vi "VIP_Phase_5.vi"() -> ()   [LabVIEW 2024]
uses:
  <vilib>/DAQmx/read.llb/DAQmx Read (Digital 1D Bool 1Chan 1Samp).vi
  <vilib>/Utility/file.llb/Write To Spreadsheet File (DBL).vi
  <vilib>/DAQmx/create/channels.llb/DAQmx Create Channel (DI-Digital Input).vi
  <vilib>/DAQmx/miscellaneous.llb/DAQmx Fill In Error Info.vi
  <vilib>/ptbypt/NI_PtbyPt.lvlib
panel:
  out "fault 4":dbl
  out "fault 3":dbl
  out "fault 2":dbl
  out "fault 1":dbl
  in  "LED 4":tag="Dev1/port0/line23"
  in  "LED 3":tag="Dev1/port0/line22"
  in  "LED 2":tag="Dev1/port0/line21"
  out "LED 4 (i)":dbl
  out "LED 3 (i)":dbl
  out "LED 2 (i)":dbl
  in  "LED 1":tag="Dev1/port0/line20"
  out "LED 1(i)":dbl
  out "4.2":bool
  out "mouse 4.2":cluster{"Y":dbl[], "Y":dbl[]}[](graph)
  out "mouse 4.1":cluster{"Y":dbl[], "Y":dbl[]}[](graph)
  in  "fake 4.2":bool
  in  "fake 4.1":bool
  out "ratio 4.2R":cluster{"Y":dbl[], "Y":dbl[]}[](graph)=[{"Y"=[2.5380001068115234, 12.063000202178955, 24.592000007629395, 36.145999908447266, 48.69600009918213, 58.23899984359741, 67.79099988937378, 81.40899991989136, 91.96199989318848, 99.9980001449585], "Y"=[0.0, 0.0, 0.0, 0.0, 0.0, 0.0, 0.0, 0.0, 0.0, 0.0]}]
  out "ratio 4.1L":cluster{"Y":dbl[], "Y":dbl[]}[](graph)=[{"Y"=[2.5380001068115234, 12.063000202178955, 24.592000007629395, 36.145999908447266, 48.69600009918213, 58.23899984359741, 67.79099988937378, 81.40899991989136, 91.96199989318848, 99.9980001449585], "Y"=[0.0, 0.0, 0.0, 0.0, 0.0, 0.0, 0.0, 0.0, 0.0, 0.0]}]
  out "ratio 4.2R":dbl
  out "ratio 4.1L":dbl
  in  "water dur (ms) 4.2":dbl=11.5
  in  "water port 4.2":tag="Dev1/port2/line0"
  out "Mouse path 4":path=path "C:/Users/Administrator/Documents/LabVIEW Data/a-lick-20140707-145848"
  out "Mouse file 4":string="a-lick-20140707-145848"
  in  "Mouse ID 4":string="test_4"
  in  "water dur (ms) 4.1":dbl=8.5
  in  "water port 4.1":tag="Dev1/port1/line7"
  in  "free water 4.2":bool
  in  "free water 4.1":bool
  out "4.1":bool
  out "state 4.2":enum16{"waiting", "sound", "ITI"}(ring)=enum."ITI"
  out "state 4.1":enum16{"waiting", "sound", "ITI"}(ring)=enum."ITI"
  out "water # 4.1L":dbl
  out "water # 4.2R":dbl
  out "lick # 4.2R":dbl
  out "lick # 4.1L":dbl
  out "last water 4.2R":dbl
  out "last water 4.1L":dbl
  out "mistake # 4.2R":dbl
  out "mistake # 4.1L":dbl
  out "ratio 3.2R":cluster{"Y":dbl[], "Y":dbl[]}[](graph)=[{"Y"=[2.5380001068115234, 12.063000202178955, 24.592000007629395, 36.145999908447266, 48.69600009918213, 58.23899984359741, 67.79099988937378, 81.40899991989136, 91.96199989318848, 99.9980001449585], "Y"=[0.0, 0.0, 0.0, 0.0, 0.0, 0.0, 0.0, 0.0, 0.0, 0.0]}]
  out "ratio 3.1L":cluster{"Y":dbl[], "Y":dbl[]}[](graph)=[{"Y"=[2.5380001068115234, 12.063000202178955, 24.592000007629395, 36.145999908447266, 48.69600009918213, 58.23899984359741, 67.79099988937378, 81.40899991989136, 91.96199989318848, 99.9980001449585], "Y"=[0.0, 0.0, 0.0, 0.0, 0.0, 0.0, 0.0, 0.0, 0.0, 0.0]}]
  in  "free water 3.2":bool
  in  "free water 3.1":bool
  in  "water dur (ms) 3. 2":dbl=25.0
  in  "water dur (ms) 3.1":dbl=25.0
  out "mouse 3.2":cluster{"Y":dbl[], "Y":dbl[]}[](graph)
  out "mouse 3.1":cluster{"Y":dbl[], "Y":dbl[]}[](graph)
  in  "fake 3.2":bool
  in  "fake 3.1":bool
  out "last water 3.2R":dbl
  out "last water 3.1L":dbl
  out "mistake # 3.2R":dbl
  out "mistake # 3.1L":dbl
  out "water # 3.2R":dbl
  out "water # 3.1L":dbl
  out "lick # 3.2R":dbl
  out "lick # 3.1L":dbl
  out "ratio 3.2R":dbl
  out "ratio 3.1L":dbl
  in  "water port 3.2":tag="Dev1/port1/line6"
  out "3.2":bool
  out "state 3.2":enum16{"waiting", "sound", "ITI"}(ring)=enum."ITI"
  out "state 3.1":enum16{"waiting", "sound", "ITI"}(ring)=enum."ITI"
  out "3.1":bool
  out "Mouse path 3":path=path "C:/Users/Administrator/Documents/LabVIEW Data/a-lick-20140707-145848"
  out "Mouse file 3":string="a-lick-20140707-145848"
  in  "water port 3.1":tag="Dev1/port1/line5"
  in  "Mouse ID 3":string="test_3"
  out "ratio 2.2R":cluster{"Y":dbl[], "Y":dbl[]}[](graph)=[{"Y"=[2.5380001068115234, 12.063000202178955, 24.592000007629395, 36.145999908447266, 48.69600009918213, 58.23899984359741, 67.79099988937378, 81.40899991989136, 91.96199989318848, 99.9980001449585], "Y"=[0.0, 0.0, 0.0, 0.0, 0.0, 0.0, 0.0, 0.0, 0.0, 0.0]}]
  out "ratio 2.1L":cluster{"Y":dbl[], "Y":dbl[]}[](graph)=[{"Y"=[2.5380001068115234, 12.063000202178955, 24.592000007629395, 36.145999908447266, 48.69600009918213, 58.23899984359741, 67.79099988937378, 81.40899991989136, 91.96199989318848, 99.9980001449585], "Y"=[0.0, 0.0, 0.0, 0.0, 0.0, 0.0, 0.0, 0.0, 0.0, 0.0]}]
  out "ratio 1.2R":cluster{"Y":dbl[], "Y":dbl[]}[](graph)=[{"Y"=[2.5380001068115234, 12.063000202178955, 24.592000007629395, 36.145999908447266, 48.69600009918213, 58.23899984359741, 67.79099988937378, 81.40899991989136, 91.96199989318848, 99.9980001449585], "Y"=[0.0, 0.0, 0.0, 0.0, 0.0, 0.0, 0.0, 0.0, 0.0, 0.0]}]
  out "mouse 2.2":cluster{"Y":dbl[], "Y":dbl[]}[](graph)
  out "mouse 2.1":cluster{"Y":dbl[], "Y":dbl[]}[](graph)
  in  "free water 2.2":bool
  in  "free water 2.1":bool
  out "last water 2.2R":dbl
  out "last water 2.1L":dbl
  out "mistake # 2.2R":dbl
  out "mistake # 2.1L":dbl
  out "water # 2.2R":dbl
  out "water # 2.1L":dbl
  out "lick  #  2.2R":dbl
  out "lick  #  2.1L":dbl
  out "2.1":bool
  out "ratio 2.2R":dbl
  out "ratio 2.1L":dbl
  out "2.2":bool
  in  "fake 2.2":bool
  in  "fake 2.1":bool
  out "Mouse path 2":path=path "C:/Users/Administrator/Documents/LabVIEW Data/a-lick-20140707-145848"
  out "Mouse file 2":string="a-lick-20140707-145848"
  in  "Mouse ID 2":string="test_2"
  in  "water dur (ms) 2.2":dbl=25.5
  in  "water dur (ms) 2.1":dbl=34.5
  in  "water port 2.2":tag="Dev1/port1/line4"
  in  "water port 2.1":tag="Dev1/port1/line3"
  out "state 2.2":enum16{"waiting", "sound", "ITI"}(ring)=enum."ITI"
  out "state 2.1":enum16{"waiting", "sound", "ITI"}(ring)=enum."ITI"
  in  "sound port 2":tag="Dev1/ao1"
  out "time (s)":dbl=103.38100004196167
  out "mistake # 1.2R":dbl
  out "mistake # 1.1L":dbl
  in  "water dur (ms) 1.1":dbl=31.0
  in  "water port 1.1":tag="Dev1/port1/line1"
  in  "water dur (ms) 1.2":dbl=25.0
  in  "water port 1.2":tag="Dev1/port1/line2"
  out "1.1":bool
  out "1.2":bool
  out "state 1.2":enum16{"waiting", "sound", "ITI"}(ring)=enum."ITI"
  out "lick # 1.2R":dbl
  out "water # 1.2R":dbl
  in  "fake 1.2":bool
  in  "free water 1.2":bool
  out "mouse 1.2":cluster{"Y":dbl[], "Y":dbl[]}[](graph)
  out "ratio 1.2R":dbl
  out "last water 1.2R":dbl
  out "ratio 1.1L":dbl
  out "ratio 1.1L":cluster{"Y":dbl[], "Y":dbl[]}[](graph)=[{"Y"=[2.5380001068115234, 12.063000202178955, 24.592000007629395, 36.145999908447266, 48.69600009918213, 58.23899984359741, 67.79099988937378, 81.40899991989136, 91.96199989318848, 99.9980001449585], "Y"=[0.0, 0.0, 0.0, 0.0, 0.0, 0.0, 0.0, 0.0, 0.0, 0.0]}]
  in  "free water 1.1":bool
  out "Right Speaker":dbl=5.0
  out "Left Speaker":dbl=5.0
  in  "sound file 2":path=path "C:/Users/cvm-gritton-lab/Documents/Lab View Programs/Lab View Programs/LabVIEW VIs/Tones/New_Phase_2_Sounds/200k_target2.wav"
  in  "ITI max (ms)":dbl=7000.0
  in  "ITI min (ms)":dbl=5000.0
  in  "reaction dur (ms)":dbl=1750.0
  in  "sound dur (ms)":dbl=3000.0
  in  "sound file 1":path=path "C:/Users/cvm-gritton-lab/Documents/Lab View Programs/Lab View Programs/LabVIEW VIs/Tones/New_Phase_2_Sounds/200k_target1.wav"
  in  "sound port 1":tag="Dev1/ao0"
  out "trial state":T1(ring)=enum."ITI"
  out "trial #":dbl=10.0
  out "current sound":dbl=1.0
  out "next sound":dbl[](array[numeric])
  out "Mouse path 1":path=path "C:/Users/Administrator/Documents/LabVIEW Data/a-lick-20140707-145848"
  in  "fake 1.1":bool
  out "mouse 1.1":cluster{"Y":dbl[], "Y":dbl[]}[](graph)
  out "ITI (s)":dbl=6.5
  out "last water 1.1L":dbl
  out "state 1.1":enum16{"waiting", "sound", "ITI"}(ring)=enum."ITI"
  out "water # 1.1L":dbl
  out "lick # 1.1L":dbl
  out "Mouse file 1":string="a-lick-20140707-145848"
  out "data folder":path=path "C:/LabVIEW VIs/LabVIEW data"
  in  "Mouse ID 1":string="test_1"
  in  "lick port":tag="Dev1/port0/line0:7"
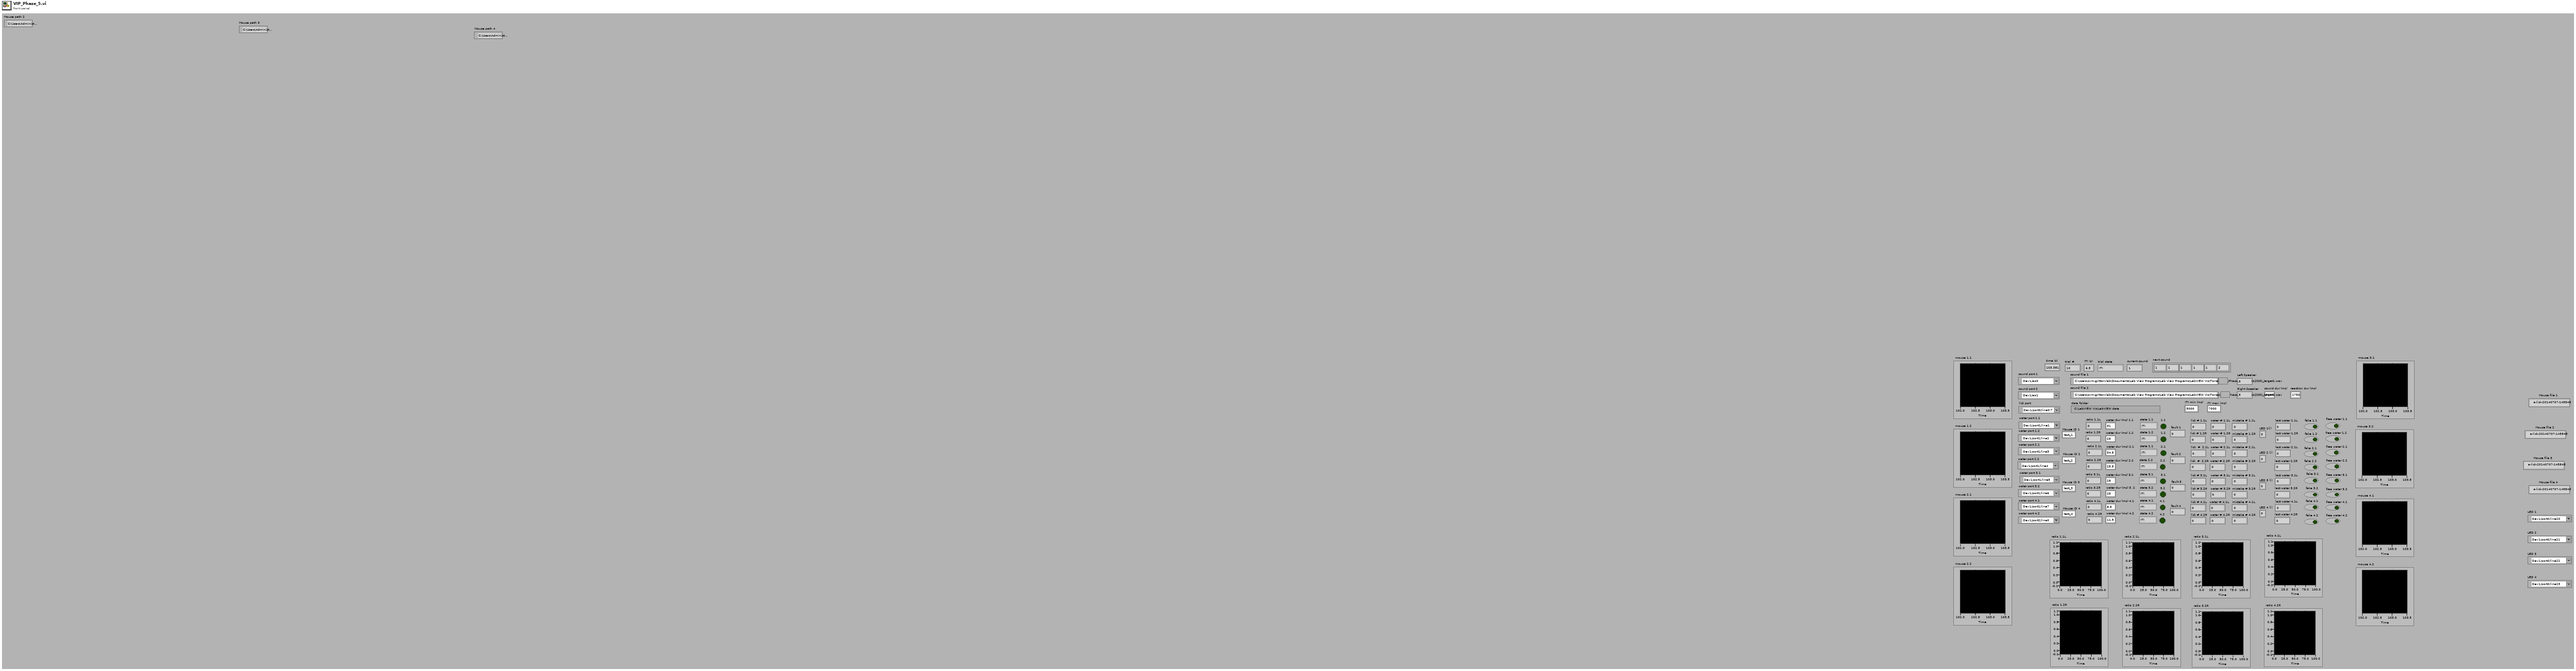
[diagram p1: front panel]
types:
  T1 = enum16{"prepare", "sound", "reaction window", "ITI", "free water", "graph", "data collection"}
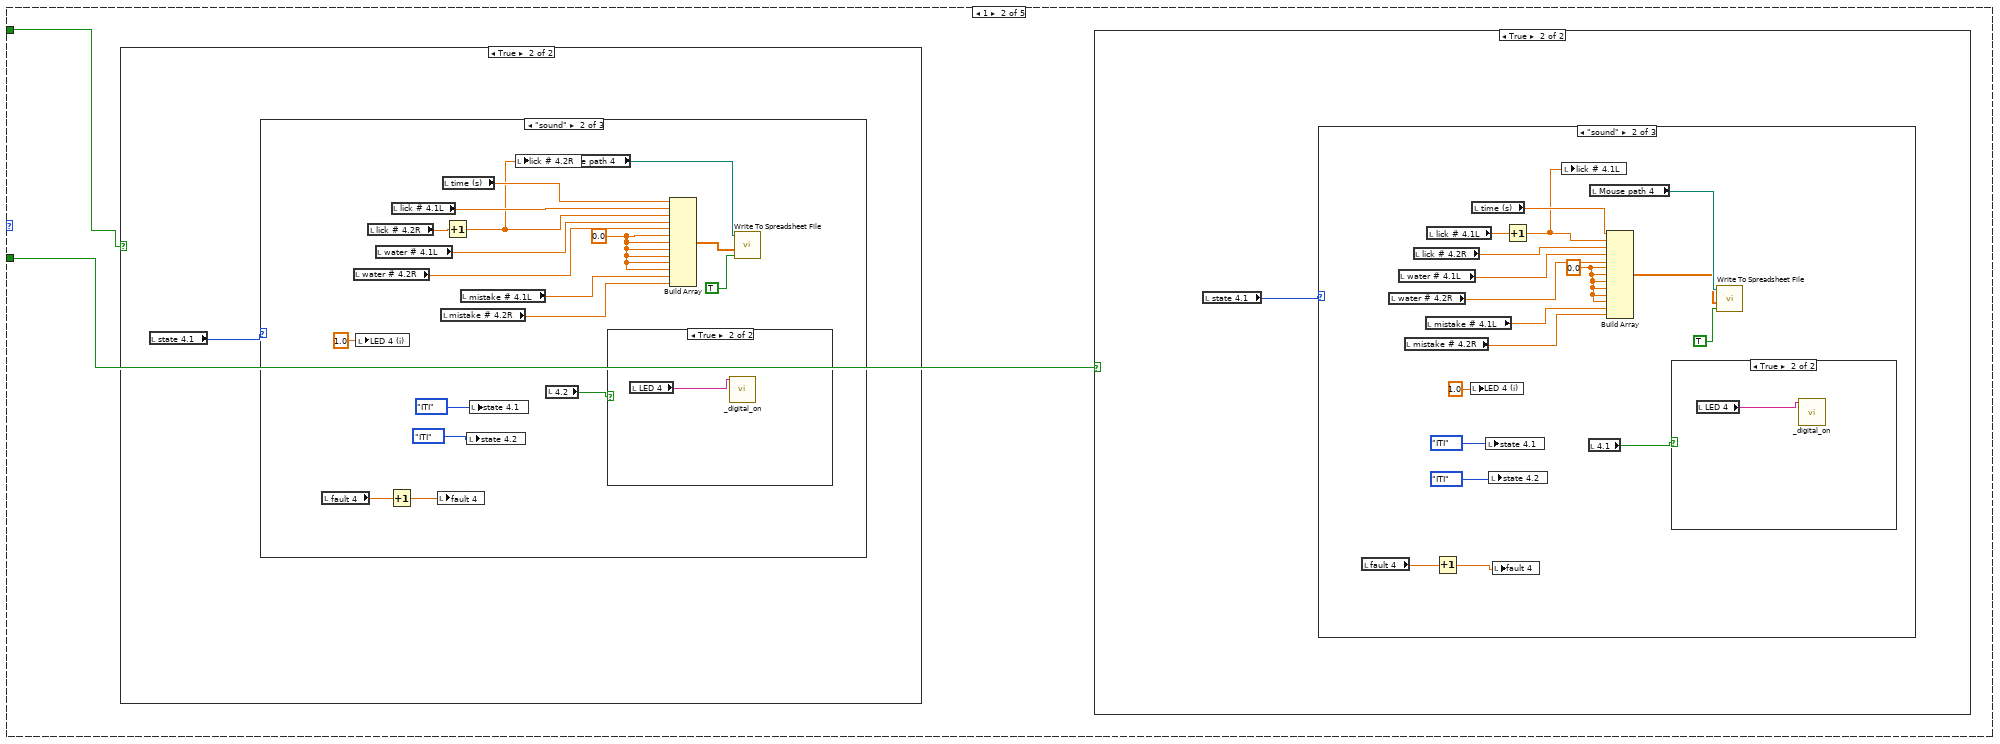
[diagram p3: hidden frame]
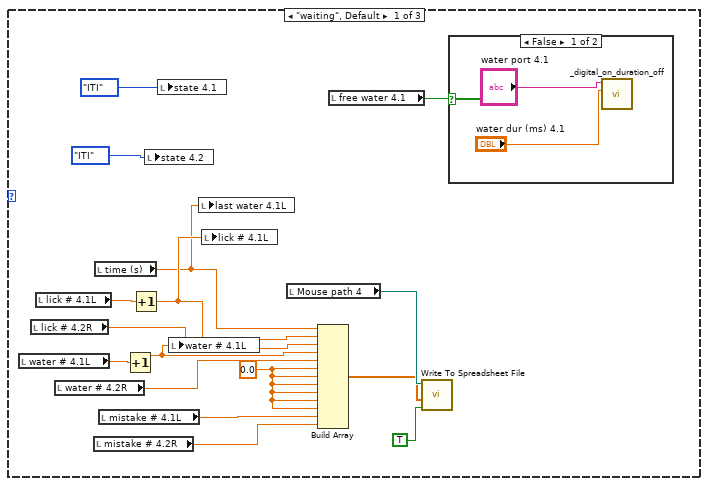
[diagram p5: hidden frame]
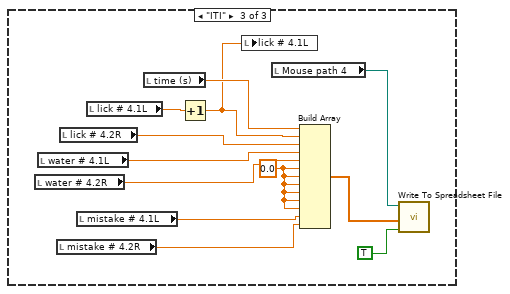
[diagram p8: hidden frame]
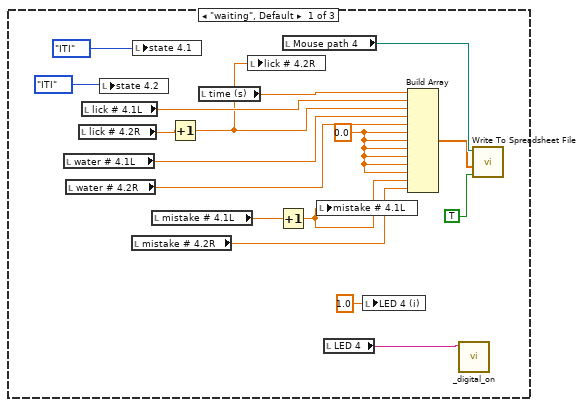
[diagram p10: hidden frame]
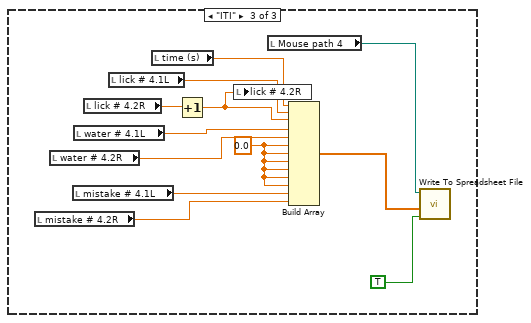
[diagram p12: hidden frame]
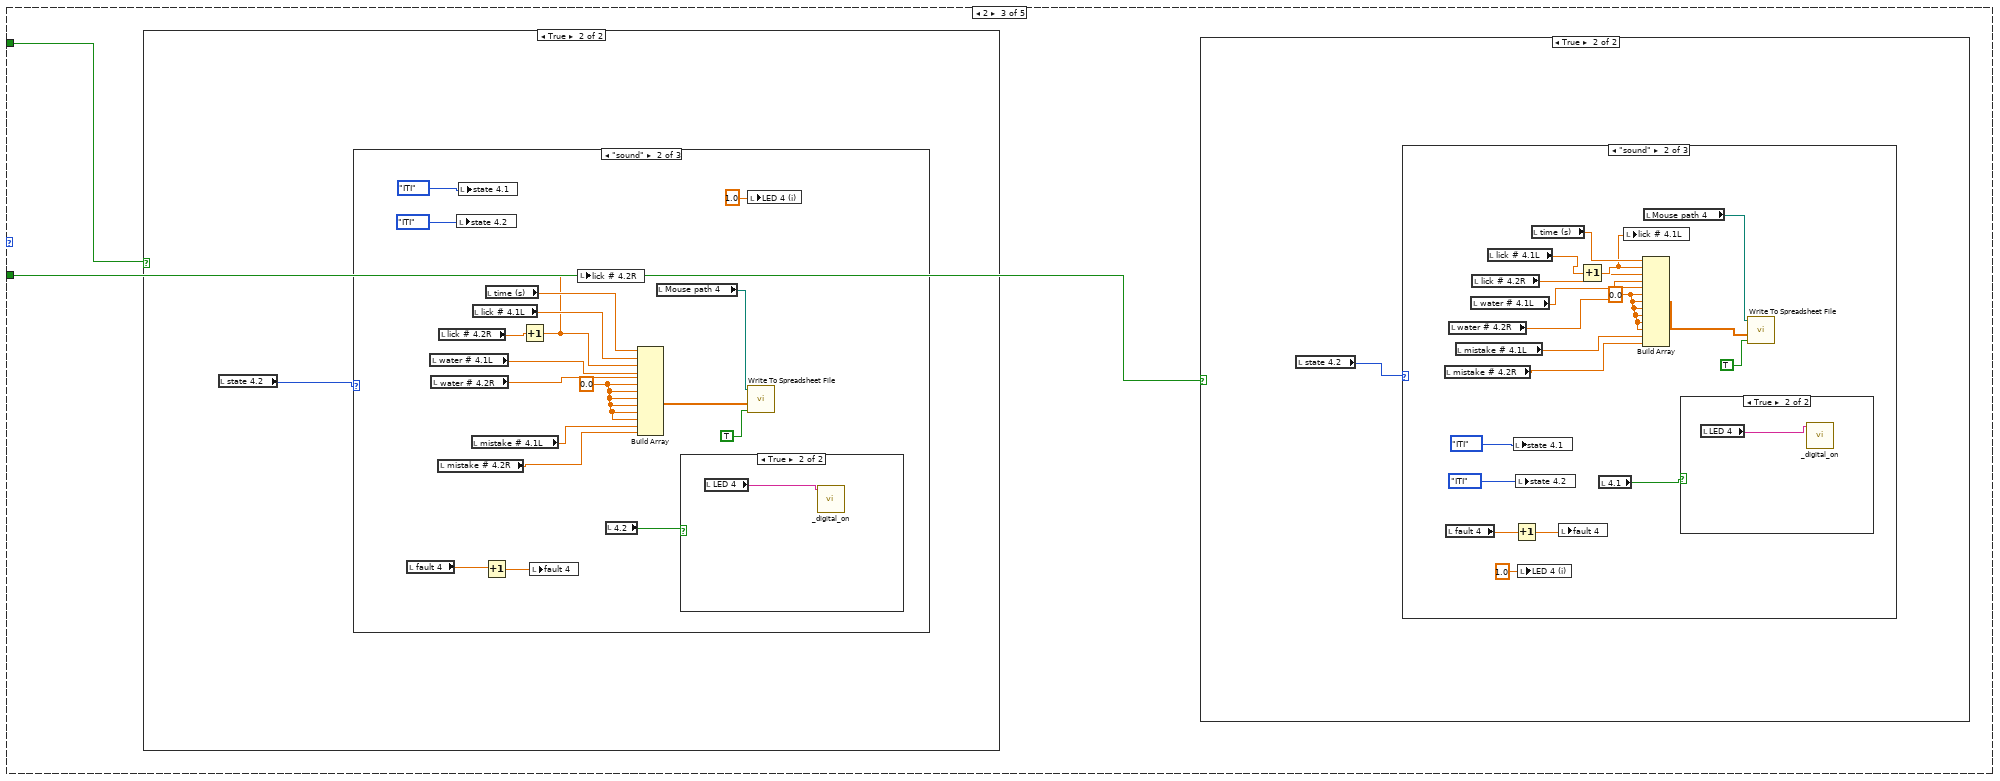
[diagram p13: hidden frame]
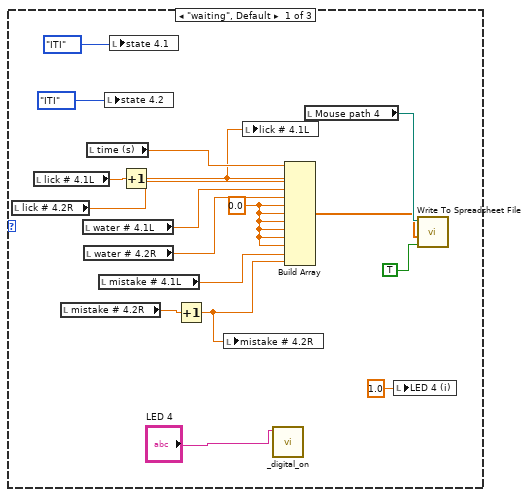
[diagram p15: hidden frame]
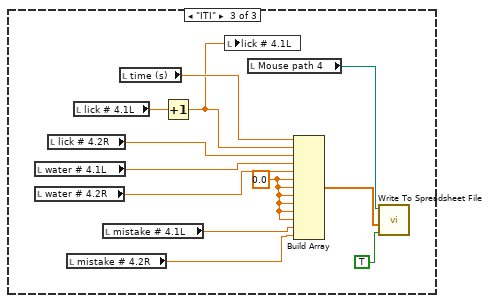
[diagram p17: hidden frame]
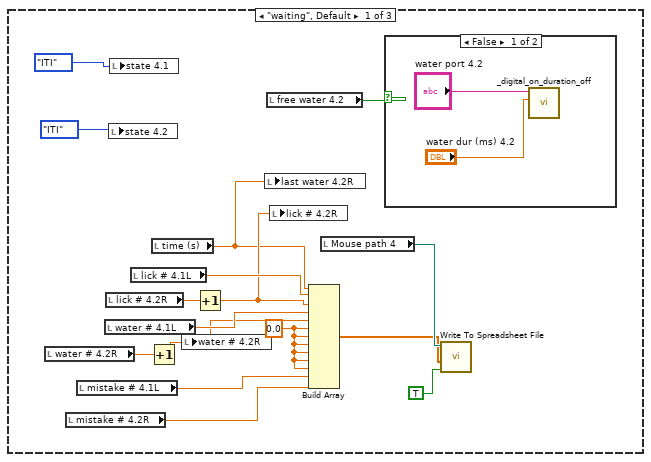
[diagram p19: hidden frame]
diagram:
  n1 = flat-sequence {
    frame #0 {
      w1 = 0.0 ("fault 1")
      w2 = 0.0 ("LED 1 (R)")
      w12 = 0.0 ("mistake # 1.1L")
      w4 = 0
      w22 = 0
      w11 = 0
      w3 = 0
      w10 = enum16{"waiting", "sound", "ITI"}."sound"
      n2 = Get Date/Time In Seconds() -> (seconds since 1Jan1904=w24:timestamp)
      n3 = call <vilib>:"Dflt Data Dir.vi"() -> ("App:Default Data Directory"=w6:path)
      "data folder" <- w6
      n4 = Format Date/Time String(time format string (%c)="%m%d%Y-%H%M%S-", seconds (now)=w24) -> (date/time string=w9:string)  [unwired: 1 in]
      n5 = Concatenate Strings(w9, "Mouse ID 1") -> (w27:string)
      "Mouse file 1" <- w27
      n6 = Concatenate Strings(w9, "Mouse ID 4") -> (w7:string)
      "Mouse file 4" <- w7
      n7 = Concatenate Strings(w9, "Mouse ID 2") -> (w17:string)
      "Mouse file 2" <- w17
      n8 = Concatenate Strings(w9, "Mouse ID 3") -> (w14:string)
      "Mouse file 3" <- w14
      n9 = Build Path(base path=w6, name or relative path=w27) -> (appended path=→"Mouse path 1":path)
      n10 = Build Path(base path=w6, name or relative path=w17) -> (appended path=→"Mouse path 2":path)
      n11 = Build Path(base path=w6, name or relative path=w14) -> (appended path=→"Mouse path 3":path)
      n12 = Build Path(base path=w6, name or relative path=w7) -> (appended path=→"Mouse path 4":path)
      n13 = call "_array_shuffle.vi"("total number"=40, "input array"=i32[] [1, 2, 3, 4, 1, 2, 3, 4]) -> ("output array"=→"next sound":dbl[])  [unwired: 9 in]
      n14 = local write "time (s)"(w22) -> ()
      "water # 1.1L" <- w3
      "lick # 1.1L" <- w3
      "state 1.1" <- w10
      "last water 1.1L" <- w11
      "current sound" <- w22
      "trial #" <- w22
      "ITI (s)" <- w22
      "Left Speaker" <- w22
      "Right Speaker" <- w22
      "ratio 1.1L" <- w4
      "last water 1.2R" <- w11
      "ratio 1.2R" <- w4
      "water # 1.2R" <- w3
      "lick # 1.2R" <- w3
      "state 1.2" <- w10
      "mistake # 1.1L" <- w12
      "mistake # 1.2R" <- w12
      "state 2.1" <- w10
      "state 2.2" <- w10
      "ratio 2.1L" <- w4
      "ratio 2.2R" <- w4
      "lick  #  2.1L" <- w3
      "lick  #  2.2R" <- w3
      "water # 2.1L" <- w3
      "water # 2.2R" <- w3
      "mistake # 2.1L" <- w12
      "mistake # 2.2R" <- w12
      "last water 2.1L" <- w11
      "last water 2.2R" <- w11
      "state 3.1" <- w10
      "state 3.2" <- w10
      "ratio 3.1L" <- w4
      "ratio 3.2R" <- w4
      "lick # 3.1L" <- w3
      "lick # 3.2R" <- w3
      "water # 3.1L" <- w3
      "water # 3.2R" <- w3
      "mistake # 3.1L" <- w12
      "mistake # 3.2R" <- w12
      "last water 3.1L" <- w11
      "last water 3.2R" <- w11
      "mistake # 4.1L" <- w12
      "mistake # 4.2R" <- w12
      "last water 4.1L" <- w11
      "last water 4.2R" <- w11
      "lick # 4.1L" <- w3
      "lick # 4.2R" <- w3
      "water # 4.2R" <- w3
      "water # 4.1L" <- w3
      "state 4.1" <- w10
      "state 4.2" <- w10
      "ratio 4.1L" <- w4
      "ratio 4.2R" <- w4
      "LED 1(i)" <- w2
      "LED 2 (i)" <- w2
      "LED 3 (i)" <- w2
      "LED 4 (i)" <- w2
      "fault 1" <- w1
      "fault 2" <- w1
      "fault 3" <- w1
      "fault 4" <- w1
    }
    frame #1 {
      # "file format:\n1. time stamp\n2. lick #\n3. water #\n4. water triggered by lick?\n5. trial start?\n6. trial #\n7. trial sound\n8. trial ITI\n9. free water?"
      n15 = call-poly <vilib>:"DAQmx Create Virtual Channel.vi"("lines"="lick port") -> ("task out"=w29:refnum<k21>)  [unwired: 13 in, 1 out]
      n16 = call <vilib>:"DAQmx Start Task.vi"("task/channels in"=w29) -> ("task out"=w30:refnum<k21>)  [unwired: 13 in, 1 out]
      n17 = while {
        tunnel: w30 -> [w89]
        tunnel: [w88] -> w31
        shift-right: [w79] -> _
        shift-left: _ -> [w87]
        shift-right: [w84] -> _
        shift-left: _ -> [w85]
        stop <- FALSE stop-if-true
        n18 = call-poly <vilib>:"DAQmx Read.vi"("task/channels in"=w89) -> ("task out"=w88:refnum<k21>, "data"=w80:bool[])  [unwired: 12 in, 1 out]
        n19 = Build Array("fake 1.1", "fake 1.2", "fake 2.1", "fake 2.2", "fake 3.1", "fake 3.2", "fake 4.1", "fake 4.2") -> (w76:bool[])
        n20 = Or(x=w80, y=w76) -> (x .or. y?=w79:bool[])
        n21 = Index Array(array=w79) -> (element #1=w82:bool, element #2=w68:bool, element #3=w59:bool, element #4=w56:bool, element #5=w48:bool, element #6=w45:bool, element #7=w40:bool, element #8=w36:bool)  [unwired: 8 in]
        n22 = call "Collector1."("Signals"=w59) -> ("Collected Signals"=w60:dynamicdata)  [unwired: 9 in, 1 out]
        n23 = call "Collector1.2"("Signals"=w68) -> ("Collected Signals"=w67:dynamicdata)  [unwired: 9 in, 1 out]
        n24 = call "Collector1.7"("Signals"=w36) -> ("Collected Signals"=w38:dynamicdata)  [unwired: 9 in, 1 out]
        n25 = call "Collector1.3"("Signals"=w56) -> ("Collected Signals"=w57:dynamicdata)  [unwired: 9 in, 1 out]
        n26 = call "Collector1.6"("Signals"=w40) -> ("Collected Signals"=w41:dynamicdata)  [unwired: 9 in, 1 out]
        n27 = call "Collector1.1"("Signals"=w82) -> ("Collected Signals"=w69:dynamicdata)  [unwired: 9 in, 1 out]
        n28 = call "Collector1.5"("Signals"=w45) -> ("Collected Signals"=w46:dynamicdata)  [unwired: 9 in, 1 out]
        n29 = call "Collector1.4"("Signals"=w48) -> ("Collected Signals"=w49:dynamicdata)  [unwired: 9 in, 1 out]
        n30 = local read "time (s)"() -> (w83:dbl)
        n31 = call "Collector"("Signals"=w83) -> ("Collected Signals"=w35:dynamicdata)  [unwired: 9 in, 1 out]
        n32 = call "Build XY Graph1.1"("Y Input"=w69, "X Input"=w35) -> ("XY Graph"=→"mouse 1.1":cluster{"Y":dbl[], "Y":dbl[]}[])  [unwired: 3 in, 6 out]
        n33 = call "Build XY Graph1."("Y Input"=w60, "X Input"=w35) -> ("XY Graph"=→"mouse 2.1":cluster{"Y":dbl[], "Y":dbl[]}[])  [unwired: 3 in, 6 out]
        n34 = call "Build XY Graph1.2"("Y Input"=w67, "X Input"=w35) -> ("XY Graph"=→"mouse 1.2":cluster{"Y":dbl[], "Y":dbl[]}[])  [unwired: 3 in, 6 out]
        n35 = call "Build XY Graph1.7"("Y Input"=w38, "X Input"=w35) -> ("XY Graph"=→"mouse 4.2":cluster{"Y":dbl[], "Y":dbl[]}[])  [unwired: 3 in, 6 out]
        n36 = call "Build XY Graph1.3"("Y Input"=w57, "X Input"=w35) -> ("XY Graph"=→"mouse 2.2":cluster{"Y":dbl[], "Y":dbl[]}[])  [unwired: 3 in, 6 out]
        n37 = call "Build XY Graph1.6"("Y Input"=w41, "X Input"=w35) -> ("XY Graph"=→"mouse 4.1":cluster{"Y":dbl[], "Y":dbl[]}[])  [unwired: 3 in, 6 out]
        n38 = call "Build XY Graph1.5"("Y Input"=w46, "X Input"=w35) -> ("XY Graph"=→"mouse 3.2":cluster{"Y":dbl[], "Y":dbl[]}[])  [unwired: 3 in, 6 out]
        n39 = call "Build XY Graph1.4"("Y Input"=w49, "X Input"=w35) -> ("XY Graph"=→"mouse 3.1":cluster{"Y":dbl[], "Y":dbl[]}[])  [unwired: 3 in, 6 out]
        n40 = Greater?(x=w79, y=w87) -> (0:w86:bool[])
        n41 = Index Array(array=w86) -> (element #1=w74:bool, element #2=w73:bool, element #3=w62:bool, element #4=w63:bool, element #5=w54:bool, element #6=w53:bool, element #7=w33:bool, element #8=w34:bool)  [unwired: 8 in]
        "1.2" <- w73
        "1.1" <- w74
        "2.2" <- w63
        "2.1" <- w62
        "3.1" <- w54
        "3.2" <- w53
        "4.1" <- w33
        "4.2" <- w34
        n42 = local read "current sound"() -> (w72:dbl)
        n43 = local read "current sound"() -> (w66:dbl)
        n44 = local read "current sound"() -> (w44:dbl)
        n45 = local read "current sound"() -> (w55:dbl)
        n46 = case shown="1" w55 {
          tunnel: w54 -> [_ w495 w596 w697 w798]
          tunnel: w53 -> [_ w494 w595 w696 w797]
          frame 0, Default {
          }
          frame 1 {
            n47 = case shown="True" w495 {
              frame False {
              }
              frame True {
                n48 = local read "state 3.1"() -> (w545:enum16{"waiting", "sound", "ITI"})
                n49 = case shown="\"sound\"" w545 {
                  frame "waiting", Default {
                    w550 = 0.0 ("element")
                    n50 = local write "state 3.2"(enum16{"waiting", "sound", "ITI"}."ITI") -> ()
                    n51 = local read "free water 3.1"() -> (w561:bool)
                    n52 = local write "state 3.1"(enum16{"waiting", "sound", "ITI"}."ITI") -> ()
                    n53 = local read "water # 3.1L"() -> (w553:dbl)
                    n54 = local read "lick # 3.2R"() -> (w554:dbl)
                    n55 = local read "lick # 3.1L"() -> (w556:dbl)
                    n56 = local read "water # 3.2R"() -> (w551:dbl)
                    n57 = case shown="False" w561 {
                      frame False {
                        n58 = call "_digital_on_duration_off.vi"("duration (ms)"="water dur (ms) 3.1", "digital port"="water port 3.1") -> ()  [unwired: 10 in]
                      }
                      frame True {
                      }
                    }
                    n59 = local read "mistake # 3.2R"() -> (w548:dbl)
                    n60 = local read "mistake # 3.1L"() -> (w549:dbl)
                    n61 = Increment(x=w553) -> (x+1=w552:dbl)
                    n62 = Increment(x=w556) -> (x+1=w555:dbl)
                    n63 = local read "time (s)"() -> (w557:dbl)
                    n64 = local write "water # 3.1L"(w552) -> ()
                    n65 = local write "lick # 3.1L"(w555) -> ()
                    n66 = local write "last water 3.1L"(w557) -> ()
                    n67 = local read "Mouse path 3"() -> (w560:path)
                    n68 = Build Array(w557, w555, w554, w552, w551, w550, w550, w550, w550, w550, w550, w549, w548) -> (w558:dbl[])
                    n69 = call-poly <vilib>:"Write To Spreadsheet File.vi"("append to file? (new file:F)"=TRUE, "1D data"=w558, "file path (dialog if empty)"=w560) -> ()  [unwired: 5 in, 1 out]
                  }
                  frame "sound" {
                    w572 = 0.0 ("element")
                    n70 = local write "LED 3 (i)"(1.0 ("LED 3 (i)")) -> ()
                    n71 = local write "state 3.2"(enum16{"waiting", "sound", "ITI"}."ITI") -> ()
                    n72 = local write "state 3.1"(enum16{"waiting", "sound", "ITI"}."ITI") -> ()
                    n73 = local read "fault 3"() -> (w565:dbl)
                    n74 = local read "water # 3.2R"() -> (w573:dbl)
                    n75 = local read "water # 3.1L"() -> (w574:dbl)
                    n76 = local read "lick # 3.2R"() -> (w575:dbl)
                    n77 = local read "mistake # 3.2R"() -> (w570:dbl)
                    n78 = local read "lick # 3.1L"() -> (w577:dbl)
                    n79 = local read "mistake # 3.1L"() -> (w571:dbl)
                    n80 = Increment(x=w565) -> (x+1=w566:dbl)
                    n81 = local read "time (s)"() -> (w578:dbl)
                    n82 = Increment(x=w577) -> (x+1=w576:dbl)
                    n83 = local read "3.1"() -> (w567:bool)
                    n84 = local write "fault 3"(w566) -> ()
                    n85 = local write "lick # 3.1L"(w576) -> ()
                    n86 = local read "Mouse path 3"() -> (w581:path)
                    n87 = case shown="True" w567 {
                      frame False {
                      }
                      frame True {
                        n88 = local read "LED 3"() -> (w582:tag)
                        n89 = call "_digital_on.vi"("digital port"=w582) -> ()  [unwired: 11 in]
                      }
                    }
                    n90 = Build Array(w578, w576, w575, w574, w573, w572, w572, w572, w572, w572, w572, w571, w570) -> (w579:dbl[])
                    n91 = call-poly <vilib>:"Write To Spreadsheet File.vi"("append to file? (new file:F)"=TRUE, "1D data"=w579, "file path (dialog if empty)"=w581) -> ()  [unwired: 5 in, 1 out]
                  }
                  frame "ITI" {
                    w585 = 0.0 ("element")
                    n92 = local read "water # 3.2R"() -> (w586:dbl)
                    n93 = local read "lick # 3.2R"() -> (w588:dbl)
                    n94 = local read "lick # 3.1L"() -> (w590:dbl)
                    n95 = local read "water # 3.1L"() -> (w587:dbl)
                    n96 = local read "time (s)"() -> (w591:dbl)
                    n97 = Increment(x=w590) -> (x+1=w589:dbl)
                    n98 = local read "mistake # 3.1L"() -> (w584:dbl)
                    n99 = local read "mistake # 3.2R"() -> (w583:dbl)
                    n100 = local write "lick # 3.1L"(w589) -> ()
                    n101 = local read "Mouse path 3"() -> (w594:path)
                    n102 = Build Array(w591, w589, w588, w587, w586, w585, w585, w585, w585, w585, w585, w584, w583) -> (w592:dbl[])
                    n103 = call-poly <vilib>:"Write To Spreadsheet File.vi"("append to file? (new file:F)"=TRUE, "1D data"=w592, "file path (dialog if empty)"=w594) -> ()  [unwired: 5 in, 1 out]
                  }
                }
              }
            }
            n104 = case shown="True" w494 {
              frame False {
              }
              frame True {
                n105 = local read "state 3.1"() -> (w496:enum16{"waiting", "sound", "ITI"})
                n106 = case shown="\"sound\"" w496 {
                  frame "waiting", Default {
                    w502 = 0.0 ("element")
                    n107 = local write "state 3.2"(enum16{"waiting", "sound", "ITI"}."ITI") -> ()
                    n108 = local write "state 3.1"(enum16{"waiting", "sound", "ITI"}."ITI") -> ()
                    n109 = local read "water # 3.2R"() -> (w503:dbl)
                    n110 = local read "water # 3.1L"() -> (w504:dbl)
                    n111 = local read "lick # 3.2R"() -> (w506:dbl)
                    n112 = local read "mistake # 3.1L"() -> (w501:dbl)
                    n113 = local read "lick # 3.1L"() -> (w507:dbl)
                    n114 = local read "mistake # 3.2R"() -> (w499:dbl)
                    n115 = local read "time (s)"() -> (w508:dbl)
                    n116 = Increment(x=w506) -> (x+1=w505:dbl)
                    n117 = local write "lick # 3.2R"(w505) -> ()
                    n118 = Increment(x=w501) -> (x+1=w500:dbl)
                    n119 = local write "mistake # 3.1L"(w500) -> ()
                    n120 = Build Array(w508, w507, w505, w504, w503, w502, w502, w502, w502, w502, w502, w500, w499) -> (w509:dbl[])
                    n121 = local read "Mouse path 3"() -> (w511:path)
                    n122 = call "_digital_on.vi"("digital port"="LED 3") -> ()  [unwired: 11 in]
                    n123 = call-poly <vilib>:"Write To Spreadsheet File.vi"("append to file? (new file:F)"=TRUE, "1D data"=w509, "file path (dialog if empty)"=w511) -> ()  [unwired: 5 in, 1 out]
                    n124 = local write "LED 3 (i)"(1.0 ("LED 3 (i)")) -> ()
                  }
                  frame "sound" {
                    w522 = 0.0 ("element")
                    n125 = local write "LED 3 (i)"(1.0 ("LED 3 (i)")) -> ()
                    n126 = local read "water # 3.1L"() -> (w524:dbl)
                    n127 = local read "lick # 3.2R"() -> (w526:dbl)
                    n128 = local write "state 3.1"(enum16{"waiting", "sound", "ITI"}."ITI") -> ()
                    n129 = local write "state 3.2"(enum16{"waiting", "sound", "ITI"}."ITI") -> ()
                    n130 = local read "water # 3.2R"() -> (w523:dbl)
                    n131 = local read "lick # 3.1L"() -> (w527:dbl)
                    n132 = local read "fault 3"() -> (w515:dbl)
                    n133 = local read "time (s)"() -> (w528:dbl)
                    n134 = Increment(x=w526) -> (x+1=w525:dbl)
                    n135 = local read "mistake # 3.2R"() -> (w520:dbl)
                    n136 = local read "mistake # 3.1L"() -> (w521:dbl)
                    n137 = local write "lick # 3.2R"(w525) -> ()
                    n138 = Increment(x=w515) -> (x+1=w516:dbl)
                    n139 = local read "3.2"() -> (w517:bool)
                    n140 = local write "fault 3"(w516) -> ()
                    n141 = case shown="True" w517 {
                      frame False {
                      }
                      frame True {
                        n142 = local read "LED 3"() -> (w532:tag)
                        n143 = call "_digital_on.vi"("digital port"=w532) -> ()  [unwired: 11 in]
                      }
                    }
                    n144 = local read "Mouse path 3"() -> (w530:path)
                    n145 = Build Array(w528, w527, w525, w524, w523, w522, w522, w522, w522, w522, w522, w521, w520) -> (w529:dbl[])
                    n146 = call-poly <vilib>:"Write To Spreadsheet File.vi"("append to file? (new file:F)"=TRUE, "1D data"=w529, "file path (dialog if empty)"=w530) -> ()  [unwired: 5 in, 1 out]
                  }
                  frame "ITI" {
                    w535 = 0.0 ("element")
                    n147 = local read "water # 3.2R"() -> (w536:dbl)
                    n148 = local read "water # 3.1L"() -> (w537:dbl)
                    n149 = local read "lick # 3.2R"() -> (w539:dbl)
                    n150 = local read "lick # 3.1L"() -> (w540:dbl)
                    n151 = Increment(x=w539) -> (x+1=w538:dbl)
                    n152 = local read "time (s)"() -> (w541:dbl)
                    n153 = local read "mistake # 3.2R"() -> (w533:dbl)
                    n154 = local read "mistake # 3.1L"() -> (w534:dbl)
                    n155 = local write "lick # 3.2R"(w538) -> ()
                    n156 = local read "Mouse path 3"() -> (w543:path)
                    n157 = Build Array(w541, w540, w538, w537, w536, w535, w535, w535, w535, w535, w535, w534, w533) -> (w542:dbl[])
                    n158 = call-poly <vilib>:"Write To Spreadsheet File.vi"("append to file? (new file:F)"=TRUE, "1D data"=w542, "file path (dialog if empty)"=w543) -> ()  [unwired: 5 in, 1 out]
                  }
                }
              }
            }
          }
          frame 2 {
            n159 = case shown="True" w596 {
              frame False {
              }
              frame True {
                n160 = local read "state 3.2"() -> (w647:enum16{"waiting", "sound", "ITI"})
                n161 = case shown="\"sound\"" w647 {
                  frame "waiting", Default {
                    w653 = 0.0 ("element")
                    n162 = local read "water # 3.2R"() -> (w654:dbl)
                    n163 = local read "water # 3.1L"() -> (w655:dbl)
                    n164 = local read "LED 3"() -> (w649:tag)
                    n165 = local read "lick # 3.2R"() -> (w656:dbl)
                    n166 = local read "lick # 3.1L"() -> (w658:dbl)
                    n167 = local write "state 3.2"(enum16{"waiting", "sound", "ITI"}."ITI") -> ()
                    n168 = local read "time (s)"() -> (w659:dbl)
                    n169 = local write "state 3.1"(enum16{"waiting", "sound", "ITI"}."ITI") -> ()
                    n170 = local read "mistake # 3.1L"() -> (w652:dbl)
                    n171 = local read "mistake # 3.2R"() -> (w651:dbl)
                    n172 = local write "LED 3 (i)"(1.0 ("LED 3 (i)")) -> ()
                    n173 = call "_digital_on.vi"("digital port"=w649) -> ()  [unwired: 11 in]
                    n174 = Increment(x=w658) -> (x+1=w657:dbl)
                    n175 = local write "lick # 3.1L"(w657) -> ()
                    n176 = local read "Mouse path 3"() -> (w661:path)
                    n177 = Increment(x=w651) -> (x+1=w650:dbl)
                    n178 = local write "mistake # 3.2R"(w650) -> ()
                    n179 = Build Array(w659, w657, w656, w655, w654, w653, w653, w653, w653, w653, w653, w652, w650) -> (w660:dbl[])
                    n180 = call-poly <vilib>:"Write To Spreadsheet File.vi"("append to file? (new file:F)"=TRUE, "1D data"=w660, "file path (dialog if empty)"=w661) -> ()  [unwired: 5 in, 1 out]
                  }
                  frame "sound" {
                    w673 = 0.0 ("element")
                    n181 = local read "water # 3.2R"() -> (w674:dbl)
                    n182 = local read "water # 3.1L"() -> (w675:dbl)
                    n183 = local read "lick # 3.2R"() -> (w676:dbl)
                    n184 = local read "fault 3"() -> (w665:dbl)
                    n185 = local read "lick # 3.1L"() -> (w678:dbl)
                    n186 = local read "mistake # 3.2R"() -> (w671:dbl)
                    n187 = local read "mistake # 3.1L"() -> (w672:dbl)
                    n188 = local read "time (s)"() -> (w679:dbl)
                    n189 = local write "LED 3 (i)"(1.0 ("LED 3 (i)")) -> ()
                    n190 = local write "state 3.2"(enum16{"waiting", "sound", "ITI"}."ITI") -> ()
                    n191 = Increment(x=w665) -> (x+1=w666:dbl)
                    n192 = local write "state 3.1"(enum16{"waiting", "sound", "ITI"}."ITI") -> ()
                    n193 = Increment(x=w678) -> (x+1=w677:dbl)
                    n194 = local write "fault 3"(w666) -> ()
                    n195 = local write "lick # 3.1L"(w677) -> ()
                    n196 = local read "3.1"() -> (w668:bool)
                    n197 = local read "Mouse path 3"() -> (w681:path)
                    n198 = Build Array(w679, w677, w676, w675, w674, w673, w673, w673, w673, w673, w673, w672, w671) -> (w680:dbl[])
                    n199 = case shown="True" w668 {
                      frame False {
                      }
                      frame True {
                        n200 = local read "LED 3"() -> (w683:tag)
                        n201 = call "_digital_on.vi"("digital port"=w683) -> ()  [unwired: 11 in]
                      }
                    }
                    n202 = call-poly <vilib>:"Write To Spreadsheet File.vi"("append to file? (new file:F)"=TRUE, "1D data"=w680, "file path (dialog if empty)"=w681) -> ()  [unwired: 5 in, 1 out]
                  }
                  frame "ITI" {
                    w686 = 0.0 ("element")
                    n203 = local read "mistake # 3.2R"() -> (w684:dbl)
                    n204 = local read "mistake # 3.1L"() -> (w685:dbl)
                    n205 = local read "water # 3.2R"() -> (w687:dbl)
                    n206 = local read "water # 3.1L"() -> (w688:dbl)
                    n207 = local read "lick # 3.2R"() -> (w689:dbl)
                    n208 = local read "lick # 3.1L"() -> (w691:dbl)
                    n209 = local read "time (s)"() -> (w692:dbl)
                    n210 = Increment(x=w691) -> (x+1=w690:dbl)
                    n211 = local write "lick # 3.1L"(w690) -> ()
                    n212 = local read "Mouse path 3"() -> (w694:path)
                    n213 = Build Array(w692, w690, w689, w688, w687, w686, w686, w686, w686, w686, w686, w685, w684) -> (w693:dbl[])
                    n214 = call-poly <vilib>:"Write To Spreadsheet File.vi"("append to file? (new file:F)"=TRUE, "1D data"=w693, "file path (dialog if empty)"=w694) -> ()  [unwired: 5 in, 1 out]
                  }
                }
              }
            }
            n215 = case shown="True" w595 {
              frame False {
              }
              frame True {
                n216 = local read "state 3.2"() -> (w597:enum16{"waiting", "sound", "ITI"})
                n217 = case shown="\"sound\"" w597 {
                  frame "waiting", Default {
                    w601 = 0.0 ("element")
                    n218 = local read "water # 3.2R"() -> (w603:dbl)
                    n219 = local read "mistake # 3.2R"() -> (w599:dbl)
                    n220 = local read "lick # 3.2R"() -> (w606:dbl)
                    n221 = local read "water # 3.1L"() -> (w604:dbl)
                    n222 = local read "mistake # 3.1L"() -> (w600:dbl)
                    n223 = local write "state 3.1"(enum16{"waiting", "sound", "ITI"}."ITI") -> ()
                    n224 = local write "state 3.2"(enum16{"waiting", "sound", "ITI"}."ITI") -> ()
                    n225 = local read "lick # 3.1L"() -> (w607:dbl)
                    n226 = local read "time (s)"() -> (w598:dbl)
                    n227 = Increment(x=w603) -> (x+1=w602:dbl)
                    n228 = Increment(x=w606) -> (x+1=w605:dbl)
                    n229 = local read "free water 3.2"() -> (w613:bool)
                    n230 = local write "water # 3.2R"(w602) -> ()
                    n231 = local write "last water 3.2R"(w598) -> ()
                    n232 = local write "lick # 3.2R"(w605) -> ()
                    n233 = local read "Mouse path 3"() -> (w609:path)
                    n234 = Build Array(w598, w607, w605, w604, w602, w601, w601, w601, w601, w601, w601, w600, w599) -> (w608:dbl[])
                    n235 = case shown="False" w613 {
                      frame False {
                        n236 = call "_digital_on_duration_off.vi"("duration (ms)"="water dur (ms) 3. 2", "digital port"="water port 3.2") -> ()  [unwired: 10 in]
                      }
                      frame True {
                      }
                    }
                    n237 = call-poly <vilib>:"Write To Spreadsheet File.vi"("append to file? (new file:F)"=TRUE, "1D data"=w608, "file path (dialog if empty)"=w609) -> ()  [unwired: 5 in, 1 out]
                  }
                  frame "sound" {
                    w624 = 0.0 ("element")
                    n238 = local read "fault 3"() -> (w616:dbl)
                    n239 = local read "lick # 3.2R"() -> (w628:dbl)
                    n240 = local read "water # 3.1L"() -> (w626:dbl)
                    n241 = local read "water # 3.2R"() -> (w625:dbl)
                    n242 = local read "lick # 3.1L"() -> (w629:dbl)
                    n243 = local read "mistake # 3.2R"() -> (w622:dbl)
                    n244 = Increment(x=w616) -> (x+1=w617:dbl)
                    n245 = local read "mistake # 3.1L"() -> (w623:dbl)
                    n246 = Increment(x=w628) -> (x+1=w627:dbl)
                    n247 = local write "LED 3 (i)"(1.0 ("LED 3 (i)")) -> ()
                    n248 = local read "time (s)"() -> (w630:dbl)
                    n249 = local write "state 3.2"(enum16{"waiting", "sound", "ITI"}."ITI") -> ()
                    n250 = local write "state 3.1"(enum16{"waiting", "sound", "ITI"}."ITI") -> ()
                    n251 = local write "fault 3"(w617) -> ()
                    n252 = local write "lick # 3.2R"(w627) -> ()
                    n253 = local read "Mouse path 3"() -> (w633:path)
                    n254 = local read "3.2"() -> (w619:bool)
                    n255 = case shown="True" w619 {
                      frame False {
                      }
                      frame True {
                        n256 = local read "LED 3"() -> (w634:tag)
                        n257 = call "_digital_on.vi"("digital port"=w634) -> ()  [unwired: 11 in]
                      }
                    }
                    n258 = Build Array(w630, w629, w627, w626, w625, w624, w624, w624, w624, w624, w624, w623, w622) -> (w631:dbl[])
                    n259 = call-poly <vilib>:"Write To Spreadsheet File.vi"("append to file? (new file:F)"=TRUE, "1D data"=w631, "file path (dialog if empty)"=w633) -> ()  [unwired: 5 in, 1 out]
                  }
                  frame "ITI" {
                    w637 = 0.0 ("element")
                    n260 = local read "water # 3.2R"() -> (w638:dbl)
                    n261 = local read "lick # 3.2R"() -> (w641:dbl)
                    n262 = local read "water # 3.1L"() -> (w639:dbl)
                    n263 = local read "lick # 3.1L"() -> (w642:dbl)
                    n264 = local read "mistake # 3.2R"() -> (w635:dbl)
                    n265 = local read "mistake # 3.1L"() -> (w636:dbl)
                    n266 = local read "time (s)"() -> (w643:dbl)
                    n267 = Increment(x=w641) -> (x+1=w640:dbl)
                    n268 = local write "lick # 3.2R"(w640) -> ()
                    n269 = local read "Mouse path 3"() -> (w645:path)
                    n270 = Build Array(w643, w642, w640, w639, w638, w637, w637, w637, w637, w637, w637, w636, w635) -> (w644:dbl[])
                    n271 = call-poly <vilib>:"Write To Spreadsheet File.vi"("append to file? (new file:F)"=TRUE, "1D data"=w644, "file path (dialog if empty)"=w645) -> ()  [unwired: 5 in, 1 out]
                  }
                }
              }
            }
          }
          frame 3 {
            n272 = case shown="True" w697 {
              frame False {
              }
              frame True {
                n273 = local read "state 3.1"() -> (w747:enum16{"waiting", "sound", "ITI"})
                n274 = case shown="\"sound\"" w747 {
                  frame "waiting", Default {
                    w750 = 0.0 ("element")
                    n275 = local read "water # 3.2R"() -> (w752:dbl)
                    n276 = local read "water # 3.1L"() -> (w754:dbl)
                    n277 = local read "lick # 3.1L"() -> (w757:dbl)
                    n278 = local write "state 3.2"(enum16{"waiting", "sound", "ITI"}."ITI") -> ()
                    n279 = local read "lick # 3.2R"() -> (w755:dbl)
                    n280 = local write "state 3.1"(enum16{"waiting", "sound", "ITI"}."ITI") -> ()
                    n281 = local read "time (s)"() -> (w751:dbl)
                    n282 = Increment(x=w757) -> (x+1=w756:dbl)
                    n283 = Increment(x=w754) -> (x+1=w753:dbl)
                    n284 = local read "mistake # 3.2R"() -> (w748:dbl)
                    n285 = local read "mistake # 3.1L"() -> (w749:dbl)
                    n286 = local read "free water 3.1"() -> (w761:bool)
                    n287 = local write "water # 3.1L"(w753) -> ()
                    n288 = local write "lick # 3.1L"(w756) -> ()
                    n289 = local write "last water 3.1L"(w751) -> ()
                    n290 = local read "Mouse path 3"() -> (w760:path)
                    n291 = case shown="False" w761 {
                      frame False {
                        n292 = local read "water dur (ms) 3.1"() -> (w764:dbl)
                        n293 = local read "water port 3.1"() -> (w765:tag)
                        n294 = call "_digital_on_duration_off.vi"("duration (ms)"=w764, "digital port"=w765) -> ()  [unwired: 10 in]
                      }
                      frame True {
                      }
                    }
                    n295 = Build Array(w751, w756, w755, w753, w752, w750, w750, w750, w750, w750, w750, w749, w748) -> (w758:dbl[])
                    n296 = call-poly <vilib>:"Write To Spreadsheet File.vi"("append to file? (new file:F)"=TRUE, "1D data"=w758, "file path (dialog if empty)"=w760) -> ()  [unwired: 5 in, 1 out]
                  }
                  frame "sound" {
                    w774 = 0.0 ("element")
                    n297 = local read "lick # 3.2R"() -> (w777:dbl)
                    n298 = local read "water # 3.2R"() -> (w775:dbl)
                    n299 = local read "water # 3.1L"() -> (w776:dbl)
                    n300 = local read "lick # 3.1L"() -> (w779:dbl)
                    n301 = local read "mistake # 3.2R"() -> (w772:dbl)
                    n302 = local read "mistake # 3.1L"() -> (w773:dbl)
                    n303 = local read "fault 3"() -> (w766:dbl)
                    n304 = Increment(x=w779) -> (x+1=w778:dbl)
                    n305 = local read "time (s)"() -> (w780:dbl)
                    n306 = local write "state 3.2"(enum16{"waiting", "sound", "ITI"}."ITI") -> ()
                    n307 = Increment(x=w766) -> (x+1=w767:dbl)
                    n308 = local write "state 3.1"(enum16{"waiting", "sound", "ITI"}."ITI") -> ()
                    n309 = local write "LED 3 (i)"(1.0 ("LED 3 (i)")) -> ()
                    n310 = local write "lick # 3.1L"(w778) -> ()
                    n311 = local read "Mouse path 3"() -> (w782:path)
                    n312 = local write "fault 3"(w767) -> ()
                    n313 = local read "3.1"() -> (w769:bool)
                    n314 = Build Array(w780, w778, w777, w776, w775, w774, w774, w774, w774, w774, w774, w773, w772) -> (w781:dbl[])
                    n315 = case shown="True" w769 {
                      frame False {
                      }
                      frame True {
                        n316 = local read "LED 3"() -> (w784:tag)
                        n317 = call "_digital_on.vi"("digital port"=w784) -> ()  [unwired: 11 in]
                      }
                    }
                    n318 = call-poly <vilib>:"Write To Spreadsheet File.vi"("append to file? (new file:F)"=TRUE, "1D data"=w781, "file path (dialog if empty)"=w782) -> ()  [unwired: 5 in, 1 out]
                  }
                  frame "ITI" {
                    w787 = 0.0 ("element")
                    n319 = local read "water # 3.2R"() -> (w788:dbl)
                    n320 = local read "water # 3.1L"() -> (w789:dbl)
                    n321 = local read "lick # 3.2R"() -> (w790:dbl)
                    n322 = local read "lick # 3.1L"() -> (w792:dbl)
                    n323 = local read "mistake # 3.2R"() -> (w785:dbl)
                    n324 = local read "mistake # 3.1L"() -> (w786:dbl)
                    n325 = local read "time (s)"() -> (w793:dbl)
                    n326 = Increment(x=w792) -> (x+1=w791:dbl)
                    n327 = local write "lick # 3.1L"(w791) -> ()
                    n328 = local read "Mouse path 3"() -> (w795:path)
                    n329 = Build Array(w793, w791, w790, w789, w788, w787, w787, w787, w787, w787, w787, w786, w785) -> (w794:dbl[])
                    n330 = call-poly <vilib>:"Write To Spreadsheet File.vi"("append to file? (new file:F)"=TRUE, "1D data"=w794, "file path (dialog if empty)"=w795) -> ()  [unwired: 5 in, 1 out]
                  }
                }
              }
            }
            n331 = case shown="True" w696 {
              frame False {
              }
              frame True {
                n332 = local read "state 3.1"() -> (w698:enum16{"waiting", "sound", "ITI"})
                n333 = case shown="\"sound\"" w698 {
                  frame "waiting", Default {
                    w704 = 0.0 ("element")
                    n334 = local write "state 3.2"(enum16{"waiting", "sound", "ITI"}."ITI") -> ()
                    n335 = local write "state 3.1"(enum16{"waiting", "sound", "ITI"}."ITI") -> ()
                    n336 = local read "LED 3"() -> (w700:tag)
                    n337 = local read "lick # 3.2R"() -> (w708:dbl)
                    n338 = local read "water # 3.2R"() -> (w705:dbl)
                    n339 = local read "water # 3.1L"() -> (w706:dbl)
                    n340 = local write "LED 3 (i)"(1.0 ("LED 3 (i)")) -> ()
                    n341 = local read "lick # 3.1L"() -> (w709:dbl)
                    n342 = local read "mistake # 3.1L"() -> (w703:dbl)
                    n343 = local read "mistake # 3.2R"() -> (w701:dbl)
                    n344 = local read "time (s)"() -> (w710:dbl)
                    n345 = call "_digital_on.vi"("digital port"=w700) -> ()  [unwired: 11 in]
                    n346 = Increment(x=w708) -> (x+1=w707:dbl)
                    n347 = local write "lick # 3.2R"(w707) -> ()
                    n348 = Increment(x=w703) -> (x+1=w702:dbl)
                    n349 = local write "mistake # 3.1L"(w702) -> ()
                    n350 = local read "Mouse path 3"() -> (w711:path)
                    n351 = Build Array(w710, w709, w707, w706, w705, w704, w704, w704, w704, w704, w704, w702, w701) -> (w712:dbl[])
                    n352 = call-poly <vilib>:"Write To Spreadsheet File.vi"("append to file? (new file:F)"=TRUE, "1D data"=w712, "file path (dialog if empty)"=w711) -> ()  [unwired: 5 in, 1 out]
                  }
                  frame "sound" {
                    w724 = 0.0 ("element")
                    n353 = local read "fault 3"() -> (w717:dbl)
                    n354 = Increment(x=w717) -> (x+1=w718:dbl)
                    n355 = local write "LED 3 (i)"(1.0 ("LED 3 (i)")) -> ()
                    n356 = local write "state 3.2"(enum16{"waiting", "sound", "ITI"}."ITI") -> ()
                    n357 = local write "state 3.1"(enum16{"waiting", "sound", "ITI"}."ITI") -> ()
                    n358 = local write "fault 3"(w718) -> ()
                    n359 = local read "water # 3.2R"() -> (w725:dbl)
                    n360 = local read "water # 3.1L"() -> (w726:dbl)
                    n361 = local read "mistake # 3.2R"() -> (w722:dbl)
                    n362 = local read "lick # 3.2R"() -> (w728:dbl)
                    n363 = local read "mistake # 3.1L"() -> (w723:dbl)
                    n364 = local read "lick # 3.1L"() -> (w729:dbl)
                    n365 = local read "time (s)"() -> (w730:dbl)
                    n366 = Increment(x=w728) -> (x+1=w727:dbl)
                    n367 = local read "3.2"() -> (w716:bool)
                    n368 = local read "Mouse path 3"() -> (w732:path)
                    n369 = local write "lick # 3.2R"(w727) -> ()
                    n370 = case shown="True" w716 {
                      frame False {
                      }
                      frame True {
                        n371 = local read "LED 3"() -> (w734:tag)
                        n372 = call "_digital_on.vi"("digital port"=w734) -> ()  [unwired: 11 in]
                      }
                    }
                    n373 = Build Array(w730, w729, w727, w726, w725, w724, w724, w724, w724, w724, w724, w723, w722) -> (w731:dbl[])
                    n374 = call-poly <vilib>:"Write To Spreadsheet File.vi"("append to file? (new file:F)"=TRUE, "1D data"=w731, "file path (dialog if empty)"=w732) -> ()  [unwired: 5 in, 1 out]
                  }
                  frame "ITI" {
                    w737 = 0.0 ("element")
                    n375 = local read "lick # 3.2R"() -> (w741:dbl)
                    n376 = local read "water # 3.2R"() -> (w738:dbl)
                    n377 = local read "water # 3.1L"() -> (w739:dbl)
                    n378 = local read "lick # 3.1L"() -> (w742:dbl)
                    n379 = local read "mistake # 3.1L"() -> (w736:dbl)
                    n380 = local read "mistake # 3.2R"() -> (w735:dbl)
                    n381 = Increment(x=w741) -> (x+1=w740:dbl)
                    n382 = local read "time (s)"() -> (w743:dbl)
                    n383 = local write "lick # 3.2R"(w740) -> ()
                    n384 = local read "Mouse path 3"() -> (w745:path)
                    n385 = Build Array(w743, w742, w740, w739, w738, w737, w737, w737, w737, w737, w737, w736, w735) -> (w744:dbl[])
                    n386 = call-poly <vilib>:"Write To Spreadsheet File.vi"("append to file? (new file:F)"=TRUE, "1D data"=w744, "file path (dialog if empty)"=w745) -> ()  [unwired: 5 in, 1 out]
                  }
                }
              }
            }
          }
          frame 4 {
            n387 = case shown="True" w798 {
              frame False {
              }
              frame True {
                n388 = local read "state 3.2"() -> (w847:enum16{"waiting", "sound", "ITI"})
                n389 = case shown="\"sound\"" w847 {
                  frame "waiting", Default {
                    w853 = 0.0 ("element")
                    n390 = local read "mistake # 3.2R"() -> (w851:dbl)
                    n391 = local read "mistake # 3.1L"() -> (w852:dbl)
                    n392 = local read "water # 3.2R"() -> (w854:dbl)
                    n393 = local read "water # 3.1L"() -> (w855:dbl)
                    n394 = local read "lick # 3.2R"() -> (w856:dbl)
                    n395 = local read "lick # 3.1L"() -> (w858:dbl)
                    n396 = local write "state 3.2"(enum16{"waiting", "sound", "ITI"}."ITI") -> ()
                    n397 = local read "LED 3"() -> (w848:tag)
                    n398 = local write "state 3.1"(enum16{"waiting", "sound", "ITI"}."ITI") -> ()
                    n399 = local write "LED 3 (i)"(1.0 ("LED 3 (i)")) -> ()
                    n400 = local read "time (s)"() -> (w859:dbl)
                    n401 = Increment(x=w851) -> (x+1=w850:dbl)
                    n402 = Increment(x=w858) -> (x+1=w857:dbl)
                    n403 = local write "mistake # 3.2R"(w850) -> ()
                    n404 = local write "lick # 3.1L"(w857) -> ()
                    n405 = local read "Mouse path 3"() -> (w861:path)
                    n406 = Build Array(w859, w857, w856, w855, w854, w853, w853, w853, w853, w853, w853, w852, w850) -> (w860:dbl[])
                    n407 = call "_digital_on.vi"("digital port"=w848) -> ()  [unwired: 11 in]
                    n408 = call-poly <vilib>:"Write To Spreadsheet File.vi"("append to file? (new file:F)"=TRUE, "1D data"=w860, "file path (dialog if empty)"=w861) -> ()  [unwired: 5 in, 1 out]
                  }
                  frame "sound" {
                    w873 = 0.0 ("element")
                    n409 = local read "mistake # 3.2R"() -> (w871:dbl)
                    n410 = local read "water # 3.2R"() -> (w874:dbl)
                    n411 = local read "mistake # 3.1L"() -> (w872:dbl)
                    n412 = local read "water # 3.1L"() -> (w875:dbl)
                    n413 = local read "lick # 3.2R"() -> (w876:dbl)
                    n414 = local read "lick # 3.1L"() -> (w878:dbl)
                    n415 = local read "fault 3"() -> (w865:dbl)
                    n416 = local write "state 3.2"(enum16{"waiting", "sound", "ITI"}."ITI") -> ()
                    n417 = local read "time (s)"() -> (w879:dbl)
                    n418 = Increment(x=w878) -> (x+1=w877:dbl)
                    n419 = local write "state 3.1"(enum16{"waiting", "sound", "ITI"}."ITI") -> ()
                    n420 = Increment(x=w865) -> (x+1=w866:dbl)
                    n421 = local read "Mouse path 3"() -> (w881:path)
                    n422 = local write "lick # 3.1L"(w877) -> ()
                    n423 = local write "fault 3"(w866) -> ()
                    n424 = Build Array(w879, w877, w876, w875, w874, w873, w873, w873, w873, w873, w873, w872, w871) -> (w880:dbl[])
                    n425 = local read "3.1"() -> (w868:bool)
                    n426 = call-poly <vilib>:"Write To Spreadsheet File.vi"("append to file? (new file:F)"=TRUE, "1D data"=w880, "file path (dialog if empty)"=w881) -> ()  [unwired: 5 in, 1 out]
                    n427 = case shown="True" w868 {
                      frame False {
                      }
                      frame True {
                        n428 = local read "LED 3"() -> (w883:tag)
                        n429 = call "_digital_on.vi"("digital port"=w883) -> ()  [unwired: 11 in]
                      }
                    }
                    n430 = local write "LED 3 (i)"(1.0 ("LED 3 (i)")) -> ()
                  }
                  frame "ITI" {
                    w886 = 0.0 ("element")
                    n431 = local read "water # 3.1L"() -> (w888:dbl)
                    n432 = local read "water # 3.2R"() -> (w887:dbl)
                    n433 = local read "lick # 3.2R"() -> (w889:dbl)
                    n434 = local read "lick # 3.1L"() -> (w891:dbl)
                    n435 = local read "mistake # 3.1L"() -> (w885:dbl)
                    n436 = local read "mistake # 3.2R"() -> (w884:dbl)
                    n437 = local read "time (s)"() -> (w892:dbl)
                    n438 = Increment(x=w891) -> (x+1=w890:dbl)
                    n439 = local write "lick # 3.1L"(w890) -> ()
                    n440 = Build Array(w892, w890, w889, w888, w887, w886, w886, w886, w886, w886, w886, w885, w884) -> (w893:dbl[])
                    n441 = local read "Mouse path 3"() -> (w894:path)
                    n442 = call-poly <vilib>:"Write To Spreadsheet File.vi"("append to file? (new file:F)"=TRUE, "1D data"=w893, "file path (dialog if empty)"=w894) -> ()  [unwired: 5 in, 1 out]
                  }
                }
              }
            }
            n443 = case shown="True" w797 {
              frame False {
              }
              frame True {
                n444 = local read "state 3.2"() -> (w799:enum16{"waiting", "sound", "ITI"})
                n445 = case shown="\"sound\"" w799 {
                  frame "waiting", Default {
                    w804 = 0.0 ("element")
                    n446 = local read "lick # 3.2R"() -> (w809:dbl)
                    n447 = local read "water # 3.2R"() -> (w806:dbl)
                    n448 = local read "water # 3.1L"() -> (w807:dbl)
                    n449 = local read "lick # 3.1L"() -> (w810:dbl)
                    n450 = local read "mistake # 3.1L"() -> (w803:dbl)
                    n451 = local read "mistake # 3.2R"() -> (w802:dbl)
                    n452 = local read "time (s)"() -> (w800:dbl)
                    n453 = Increment(x=w809) -> (x+1=w808:dbl)
                    n454 = Increment(x=w806) -> (x+1=w805:dbl)
                    n455 = local write "water # 3.2R"(w805) -> ()
                    n456 = local write "state 3.2"(enum16{"waiting", "sound", "ITI"}."ITI") -> ()
                    n457 = local write "state 3.1"(enum16{"waiting", "sound", "ITI"}."ITI") -> ()
                    n458 = local write "last water 3.2R"(w800) -> ()
                    n459 = local write "lick # 3.2R"(w808) -> ()
                    n460 = local read "Mouse path 3"() -> (w812:path)
                    n461 = local read "free water 3.2"() -> (w801:bool)
                    n462 = Build Array(w800, w810, w808, w807, w805, w804, w804, w804, w804, w804, w804, w803, w802) -> (w811:dbl[])
                    n463 = call-poly <vilib>:"Write To Spreadsheet File.vi"("append to file? (new file:F)"=TRUE, "1D data"=w811, "file path (dialog if empty)"=w812) -> ()  [unwired: 5 in, 1 out]
                    n464 = case shown="False" w801 {
                      frame False {
                        n465 = local read "water dur (ms) 3. 2"() -> (w817:dbl)
                        n466 = local read "water port 3.2"() -> (w816:tag)
                        n467 = call "_digital_on_duration_off.vi"("duration (ms)"=w817, "digital port"=w816) -> ()  [unwired: 10 in]
                      }
                      frame True {
                      }
                    }
                  }
                  frame "sound" {
                    w824 = 0.0 ("element")
                    n468 = local read "water # 3.2R"() -> (w825:dbl)
                    n469 = local read "water # 3.1L"() -> (w826:dbl)
                    n470 = local read "lick # 3.2R"() -> (w828:dbl)
                    n471 = local read "mistake # 3.2R"() -> (w822:dbl)
                    n472 = local read "lick # 3.1L"() -> (w829:dbl)
                    n473 = local read "mistake # 3.1L"() -> (w823:dbl)
                    n474 = local read "time (s)"() -> (w830:dbl)
                    n475 = local write "state 3.2"(enum16{"waiting", "sound", "ITI"}."ITI") -> ()
                    n476 = Increment(x=w828) -> (x+1=w827:dbl)
                    n477 = local write "state 3.1"(enum16{"waiting", "sound", "ITI"}."ITI") -> ()
                    n478 = local write "lick # 3.2R"(w827) -> ()
                    n479 = local read "Mouse path 3"() -> (w832:path)
                    n480 = Build Array(w830, w829, w827, w826, w825, w824, w824, w824, w824, w824, w824, w823, w822) -> (w831:dbl[])
                    n481 = local read "3.2"() -> (w818:bool)
                    n482 = case shown="True" w818 {
                      frame False {
                      }
                      frame True {
                        n483 = local read "LED 3"() -> (w834:tag)
                        n484 = call "_digital_on.vi"("digital port"=w834) -> ()  [unwired: 11 in]
                      }
                    }
                    n485 = call-poly <vilib>:"Write To Spreadsheet File.vi"("append to file? (new file:F)"=TRUE, "1D data"=w831, "file path (dialog if empty)"=w832) -> ()  [unwired: 5 in, 1 out]
                    n486 = local write "LED 3 (i)"(1.0 ("LED 3 (i)")) -> ()
                  }
                  frame "ITI" {
                    w837 = 0.0 ("element")
                    n487 = local read "water # 3.2R"() -> (w838:dbl)
                    n488 = local read "lick # 3.2R"() -> (w841:dbl)
                    n489 = local read "water # 3.1L"() -> (w839:dbl)
                    n490 = local read "mistake # 3.2R"() -> (w835:dbl)
                    n491 = local read "lick # 3.1L"() -> (w842:dbl)
                    n492 = local read "mistake # 3.1L"() -> (w836:dbl)
                    n493 = local read "time (s)"() -> (w843:dbl)
                    n494 = Increment(x=w841) -> (x+1=w840:dbl)
                    n495 = local write "lick # 3.2R"(w840) -> ()
                    n496 = local read "Mouse path 3"() -> (w845:path)
                    n497 = Build Array(w843, w842, w840, w839, w838, w837, w837, w837, w837, w837, w837, w836, w835) -> (w844:dbl[])
                    n498 = call-poly <vilib>:"Write To Spreadsheet File.vi"("append to file? (new file:F)"=TRUE, "1D data"=w844, "file path (dialog if empty)"=w845) -> ()  [unwired: 5 in, 1 out]
                  }
                }
              }
            }
          }
        }
        n499 = case shown="1" w66 {
          tunnel: w62 -> [_ w897 w998 w1099 w1200]
          tunnel: w63 -> [_ w896 w997 w1098 w1199]
          frame 0, Default {
          }
          frame 1 {
            n500 = case shown="True" w897 {
              frame False {
              }
              frame True {
                n501 = local read "state 2.1"() -> (w947:enum16{"waiting", "sound", "ITI"})
                n502 = case shown="\"sound\"" w947 {
                  frame "waiting", Default {
                    w952 = 0.0 ("element")
                    n503 = local read "free water 2.1"() -> (w948:bool)
                    n504 = case shown="False" w948 {
                      frame False {
                        n505 = call "_digital_on_duration_off.vi"("duration (ms)"="water dur (ms) 2.1", "digital port"="water port 2.1") -> ()  [unwired: 10 in]
                      }
                      frame True {
                      }
                    }
                    n506 = local write "state 2.2"(enum16{"waiting", "sound", "ITI"}."ITI") -> ()
                    n507 = local write "state 2.1"(enum16{"waiting", "sound", "ITI"}."ITI") -> ()
                    n508 = local read "lick  #  2.1L"() -> (w958:dbl)
                    n509 = local read "water # 2.2R"() -> (w953:dbl)
                    n510 = local read "water # 2.1L"() -> (w955:dbl)
                    n511 = local read "lick  #  2.2R"() -> (w956:dbl)
                    n512 = Increment(x=w958) -> (x+1=w957:dbl)
                    n513 = local read "mistake # 2.2R"() -> (w950:dbl)
                    n514 = local read "mistake # 2.1L"() -> (w951:dbl)
                    n515 = Increment(x=w955) -> (x+1=w954:dbl)
                    n516 = local read "time (s)"() -> (w949:dbl)
                    n517 = local write "lick  #  2.1L"(w957) -> ()
                    n518 = local write "water # 2.1L"(w954) -> ()
                    n519 = local write "last water 2.1L"(w949) -> ()
                    n520 = local read "Mouse path 2"() -> (w961:path)
                    n521 = Build Array(w949, w957, w956, w954, w953, w952, w952, w952, w952, w952, w952, w951, w950) -> (w959:dbl[])
                    n522 = call-poly <vilib>:"Write To Spreadsheet File.vi"("append to file? (new file:F)"=TRUE, "1D data"=w959, "file path (dialog if empty)"=w961) -> ()  [unwired: 5 in, 1 out]
                  }
                  frame "sound" {
                    w974 = 0.0 ("element")
                    n523 = local read "fault 2"() -> (w966:dbl)
                    n524 = local write "state 2.2"(enum16{"waiting", "sound", "ITI"}."ITI") -> ()
                    n525 = local write "state 2.1"(enum16{"waiting", "sound", "ITI"}."ITI") -> ()
                    n526 = Increment(x=w966) -> (x+1=w967:dbl)
                    n527 = local read "water # 2.2R"() -> (w975:dbl)
                    n528 = local read "water # 2.1L"() -> (w976:dbl)
                    n529 = local read "lick  #  2.2R"() -> (w977:dbl)
                    n530 = local read "lick  #  2.1L"() -> (w979:dbl)
                    n531 = local write "fault 2"(w967) -> ()
                    n532 = local read "mistake # 2.2R"() -> (w972:dbl)
                    n533 = local read "mistake # 2.1L"() -> (w973:dbl)
                    n534 = local read "time (s)"() -> (w980:dbl)
                    n535 = Increment(x=w979) -> (x+1=w978:dbl)
                    n536 = local write "lick  #  2.1L"(w978) -> ()
                    n537 = local read "2.1"() -> (w968:bool)
                    n538 = local read "Mouse path 2"() -> (w983:path)
                    n539 = Build Array(w980, w978, w977, w976, w975, w974, w974, w974, w974, w974, w974, w973, w972) -> (w981:dbl[])
                    n540 = case shown="True" w968 {
                      frame False {
                      }
                      frame True {
                        n541 = local read "LED 2"() -> (w984:tag)
                        n542 = call "_digital_on.vi"("digital port"=w984) -> ()  [unwired: 11 in]
                      }
                    }
                    n543 = call-poly <vilib>:"Write To Spreadsheet File.vi"("append to file? (new file:F)"=TRUE, "1D data"=w981, "file path (dialog if empty)"=w983) -> ()  [unwired: 5 in, 1 out]
                    n544 = local write "LED 2 (i)"(1.0 ("LED 2 (i)")) -> ()
                  }
                  frame "ITI" {
                    w987 = 0.0 ("element")
                    n545 = local read "water # 2.2R"() -> (w988:dbl)
                    n546 = local read "water # 2.1L"() -> (w989:dbl)
                    n547 = local read "lick  #  2.2R"() -> (w990:dbl)
                    n548 = local read "lick  #  2.1L"() -> (w992:dbl)
                    n549 = local read "time (s)"() -> (w993:dbl)
                    n550 = local read "mistake # 2.2R"() -> (w985:dbl)
                    n551 = local read "mistake # 2.1L"() -> (w986:dbl)
                    n552 = Increment(x=w992) -> (x+1=w991:dbl)
                    n553 = local write "lick  #  2.1L"(w991) -> ()
                    n554 = local read "Mouse path 2"() -> (w995:path)
                    n555 = Build Array(w993, w991, w990, w989, w988, w987, w987, w987, w987, w987, w987, w986, w985) -> (w994:dbl[])
                    n556 = call-poly <vilib>:"Write To Spreadsheet File.vi"("append to file? (new file:F)"=TRUE, "1D data"=w994, "file path (dialog if empty)"=w995) -> ()  [unwired: 5 in, 1 out]
                  }
                }
              }
            }
            n557 = case shown="True" w896 {
              frame False {
              }
              frame True {
                n558 = local read "state 2.1"() -> (w898:enum16{"waiting", "sound", "ITI"})
                n559 = case shown="\"sound\"" w898 {
                  frame "waiting", Default {
                    w904 = 0.0 ("element")
                    n560 = local read "mistake # 2.1L"() -> (w903:dbl)
                    n561 = local read "mistake # 2.2R"() -> (w901:dbl)
                    n562 = local read "water # 2.2R"() -> (w905:dbl)
                    n563 = local read "lick  #  2.2R"() -> (w909:dbl)
                    n564 = local read "water # 2.1L"() -> (w906:dbl)
                    n565 = local read "lick  #  2.1L"() -> (w908:dbl)
                    n566 = local write "state 2.2"(enum16{"waiting", "sound", "ITI"}."ITI") -> ()
                    n567 = local read "time (s)"() -> (w910:dbl)
                    n568 = Increment(x=w909) -> (x+1=w907:dbl)
                    n569 = Increment(x=w903) -> (x+1=w902:dbl)
                    n570 = local write "state 2.1"(enum16{"waiting", "sound", "ITI"}."ITI") -> ()
                    n571 = local write "mistake # 2.1L"(w902) -> ()
                    n572 = local write "lick  #  2.2R"(w907) -> ()
                    n573 = local write "LED 2 (i)"(1.0 ("LED 2 (i)")) -> ()
                    n574 = local read "Mouse path 2"() -> (w913:path)
                    n575 = Build Array(w910, w908, w907, w906, w905, w904, w904, w904, w904, w904, w904, w902, w901) -> (w912:dbl[])
                    n576 = call "_digital_on.vi"("digital port"="LED 2") -> ()  [unwired: 11 in]
                    n577 = call-poly <vilib>:"Write To Spreadsheet File.vi"("append to file? (new file:F)"=TRUE, "1D data"=w912, "file path (dialog if empty)"=w913) -> ()  [unwired: 5 in, 1 out]
                  }
                  frame "ITI" {
                    w918 = 0.0 ("element")
                    n578 = local read "water # 2.2R"() -> (w919:dbl)
                    n579 = local read "lick  #  2.2R"() -> (w922:dbl)
                    n580 = local read "water # 2.1L"() -> (w920:dbl)
                    n581 = local read "lick  #  2.1L"() -> (w923:dbl)
                    n582 = local read "mistake # 2.2R"() -> (w916:dbl)
                    n583 = Increment(x=w922) -> (x+1=w921:dbl)
                    n584 = local read "time (s)"() -> (w924:dbl)
                    n585 = local read "mistake # 2.1L"() -> (w917:dbl)
                    n586 = local write "lick  #  2.2R"(w921) -> ()
                    n587 = local read "Mouse path 2"() -> (w926:path)
                    n588 = Build Array(w924, w923, w921, w920, w919, w918, w918, w918, w918, w918, w918, w917, w916) -> (w925:dbl[])
                    n589 = call-poly <vilib>:"Write To Spreadsheet File.vi"("append to file? (new file:F)"=TRUE, "1D data"=w925, "file path (dialog if empty)"=w926) -> ()  [unwired: 5 in, 1 out]
                  }
                  frame "sound" {
                    w936 = 0.0 ("element")
                    n590 = local read "water # 2.2R"() -> (w937:dbl)
                    n591 = local read "water # 2.1L"() -> (w938:dbl)
                    n592 = local read "lick  #  2.2R"() -> (w940:dbl)
                    n593 = local write "state 2.2"(enum16{"waiting", "sound", "ITI"}."ITI") -> ()
                    n594 = local write "state 2.1"(enum16{"waiting", "sound", "ITI"}."ITI") -> ()
                    n595 = local read "lick  #  2.1L"() -> (w941:dbl)
                    n596 = local read "mistake # 2.2R"() -> (w934:dbl)
                    n597 = local read "mistake # 2.1L"() -> (w935:dbl)
                    n598 = local write "LED 2 (i)"(1.0 ("LED 2 (i)")) -> ()
                    n599 = Increment(x=w940) -> (x+1=w939:dbl)
                    n600 = local read "time (s)"() -> (w942:dbl)
                    n601 = local read "2.2"() -> (w931:bool)
                    n602 = local write "lick  #  2.2R"(w939) -> ()
                    n603 = local read "fault 2"() -> (w928:dbl)
                    n604 = case shown="True" w931 {
                      frame False {
                      }
                      frame True {
                        n605 = local read "LED 2"() -> (w946:tag)
                        n606 = call "_digital_on.vi"("digital port"=w946) -> ()  [unwired: 11 in]
                      }
                    }
                    n607 = Increment(x=w928) -> (x+1=w929:dbl)
                    n608 = local read "Mouse path 2"() -> (w944:path)
                    n609 = Build Array(w942, w941, w939, w938, w937, w936, w936, w936, w936, w936, w936, w935, w934) -> (w943:dbl[])
                    n610 = local write "fault 2"(w929) -> ()
                    n611 = call-poly <vilib>:"Write To Spreadsheet File.vi"("append to file? (new file:F)"=TRUE, "1D data"=w943, "file path (dialog if empty)"=w944) -> ()  [unwired: 5 in, 1 out]
                  }
                }
              }
            }
          }
          frame 2 {
            n612 = case shown="True" w998 {
              frame False {
              }
              frame True {
                n613 = local read "state 2.2"() -> (w1049:enum16{"waiting", "sound", "ITI"})
                n614 = case shown="\"sound\"" w1049 {
                  frame "waiting", Default {
                    w1055 = 0.0 ("element")
                    n615 = local read "LED 2"() -> (w1050:tag)
                    n616 = local write "state 2.2"(enum16{"waiting", "sound", "ITI"}."ITI") -> ()
                    n617 = local write "state 2.1"(enum16{"waiting", "sound", "ITI"}."ITI") -> ()
                    n618 = local read "mistake # 2.2R"() -> (w1053:dbl)
                    n619 = local read "water # 2.2R"() -> (w1056:dbl)
                    n620 = local read "water # 2.1L"() -> (w1057:dbl)
                    n621 = local read "lick  #  2.2R"() -> (w1058:dbl)
                    n622 = local read "mistake # 2.1L"() -> (w1054:dbl)
                    n623 = local read "lick  #  2.1L"() -> (w1060:dbl)
                    n624 = call "_digital_on.vi"("digital port"=w1050) -> ()  [unwired: 11 in]
                    n625 = Increment(x=w1053) -> (x+1=w1052:dbl)
                    n626 = local read "time (s)"() -> (w1061:dbl)
                    n627 = Increment(x=w1060) -> (x+1=w1059:dbl)
                    n628 = local write "mistake # 2.2R"(w1052) -> ()
                    n629 = local write "lick  #  2.1L"(w1059) -> ()
                    n630 = local read "Mouse path 2"() -> (w1063:path)
                    n631 = Build Array(w1061, w1059, w1058, w1057, w1056, w1055, w1055, w1055, w1055, w1055, w1055, w1054, w1052) -> (w1062:dbl[])
                    n632 = local write "LED 2 (i)"(1.0 ("LED 2 (i)")) -> ()
                    n633 = call-poly <vilib>:"Write To Spreadsheet File.vi"("append to file? (new file:F)"=TRUE, "1D data"=w1062, "file path (dialog if empty)"=w1063) -> ()  [unwired: 5 in, 1 out]
                  }
                  frame "sound" {
                    w1075 = 0.0 ("element")
                    n634 = local read "fault 2"() -> (w1067:dbl)
                    n635 = local read "water # 2.2R"() -> (w1076:dbl)
                    n636 = local read "water # 2.1L"() -> (w1077:dbl)
                    n637 = local read "lick  #  2.2R"() -> (w1078:dbl)
                    n638 = local read "mistake # 2.2R"() -> (w1073:dbl)
                    n639 = local read "mistake # 2.1L"() -> (w1074:dbl)
                    n640 = local read "lick  #  2.1L"() -> (w1080:dbl)
                    n641 = Increment(x=w1067) -> (x+1=w1068:dbl)
                    n642 = local write "state 2.1"(enum16{"waiting", "sound", "ITI"}."ITI") -> ()
                    n643 = local write "state 2.2"(enum16{"waiting", "sound", "ITI"}."ITI") -> ()
                    n644 = Increment(x=w1080) -> (x+1=w1079:dbl)
                    n645 = local write "fault 2"(w1068) -> ()
                    n646 = local read "time (s)"() -> (w1081:dbl)
                    n647 = local write "lick  #  2.1L"(w1079) -> ()
                    n648 = local read "Mouse path 2"() -> (w1083:path)
                    n649 = Build Array(w1081, w1079, w1078, w1077, w1076, w1075, w1075, w1075, w1075, w1075, w1075, w1074, w1073) -> (w1082:dbl[])
                    n650 = local read "2.1"() -> (w1069:bool)
                    n651 = call-poly <vilib>:"Write To Spreadsheet File.vi"("append to file? (new file:F)"=TRUE, "1D data"=w1082, "file path (dialog if empty)"=w1083) -> ()  [unwired: 5 in, 1 out]
                    n652 = case shown="True" w1069 {
                      frame False {
                      }
                      frame True {
                        n653 = local read "LED 2"() -> (w1085:tag)
                        n654 = call "_digital_on.vi"("digital port"=w1085) -> ()  [unwired: 11 in]
                      }
                    }
                    n655 = local write "LED 2 (i)"(1.0 ("LED 2 (i)")) -> ()
                  }
                  frame "ITI" {
                    w1088 = 0.0 ("element")
                    n656 = local read "water # 2.2R"() -> (w1089:dbl)
                    n657 = local read "water # 2.1L"() -> (w1090:dbl)
                    n658 = local read "lick  #  2.1L"() -> (w1093:dbl)
                    n659 = local read "lick  #  2.2R"() -> (w1091:dbl)
                    n660 = local read "time (s)"() -> (w1094:dbl)
                    n661 = Increment(x=w1093) -> (x+1=w1092:dbl)
                    n662 = local write "lick  #  2.1L"(w1092) -> ()
                    n663 = local read "Mouse path 2"() -> (w1096:path)
                    n664 = local read "mistake # 2.2R"() -> (w1086:dbl)
                    n665 = local read "mistake # 2.1L"() -> (w1087:dbl)
                    n666 = Build Array(w1094, w1092, w1091, w1090, w1089, w1088, w1088, w1088, w1088, w1088, w1088, w1087, w1086) -> (w1095:dbl[])
                    n667 = call-poly <vilib>:"Write To Spreadsheet File.vi"("append to file? (new file:F)"=TRUE, "1D data"=w1095, "file path (dialog if empty)"=w1096) -> ()  [unwired: 5 in, 1 out]
                  }
                }
              }
            }
            n668 = case shown="True" w997 {
              frame False {
              }
              frame True {
                n669 = local read "state 2.2"() -> (w999:enum16{"waiting", "sound", "ITI"})
                n670 = case shown="\"sound\"" w999 {
                  frame "waiting", Default {
                    w1006 = 0.0 ("element")
                    n671 = local read "water # 2.2R"() -> (w1001:dbl)
                    n672 = local read "water # 2.1L"() -> (w1007:dbl)
                    n673 = local read "lick  #  2.2R"() -> (w1009:dbl)
                    n674 = local read "mistake # 2.2R"() -> (w1004:dbl)
                    n675 = local read "mistake # 2.1L"() -> (w1005:dbl)
                    n676 = local read "lick  #  2.1L"() -> (w1010:dbl)
                    n677 = local read "time (s)"() -> (w1003:dbl)
                    n678 = Increment(x=w1001) -> (x+1=w1000:dbl)
                    n679 = Increment(x=w1009) -> (x+1=w1008:dbl)
                    n680 = local write "water # 2.2R"(w1000) -> ()
                    n681 = local read "free water 2.2"() -> (w1002:bool)
                    n682 = local write "lick  #  2.2R"(w1008) -> ()
                    n683 = local write "last water 2.2R"(w1003) -> ()
                    n684 = local read "Mouse path 2"() -> (w1012:path)
                    n685 = Build Array(w1003, w1010, w1008, w1007, w1000, w1006, w1006, w1006, w1006, w1006, w1006, w1005, w1004) -> (w1011:dbl[])
                    n686 = case shown="False" w1002 {
                      frame False {
                        n687 = call "_digital_on_duration_off.vi"("duration (ms)"="water dur (ms) 2.2", "digital port"="water port 2.2") -> ()  [unwired: 10 in]
                      }
                      frame True {
                      }
                    }
                    n688 = local write "state 2.2"(enum16{"waiting", "sound", "ITI"}."ITI") -> ()
                    n689 = call-poly <vilib>:"Write To Spreadsheet File.vi"("append to file? (new file:F)"=TRUE, "1D data"=w1011, "file path (dialog if empty)"=w1012) -> ()  [unwired: 5 in, 1 out]
                    n690 = local write "state 2.1"(enum16{"waiting", "sound", "ITI"}."ITI") -> ()
                  }
                  frame "ITI" {
                    w1020 = 0.0 ("element")
                    n691 = local read "water # 2.2R"() -> (w1021:dbl)
                    n692 = local read "water # 2.1L"() -> (w1022:dbl)
                    n693 = local read "lick  #  2.2R"() -> (w1024:dbl)
                    n694 = local read "mistake # 2.2R"() -> (w1018:dbl)
                    n695 = local read "mistake # 2.1L"() -> (w1019:dbl)
                    n696 = local read "lick  #  2.1L"() -> (w1025:dbl)
                    n697 = local read "time (s)"() -> (w1026:dbl)
                    n698 = Increment(x=w1024) -> (x+1=w1023:dbl)
                    n699 = local write "lick  #  2.2R"(w1023) -> ()
                    n700 = local read "Mouse path 2"() -> (w1029:path)
                    n701 = Build Array(w1026, w1025, w1023, w1022, w1021, w1020, w1020, w1020, w1020, w1020, w1020, w1019, w1018) -> (w1027:dbl[])
                    n702 = call-poly <vilib>:"Write To Spreadsheet File.vi"("append to file? (new file:F)"=TRUE, "1D data"=w1027, "file path (dialog if empty)"=w1029) -> ()  [unwired: 5 in, 1 out]
                  }
                  frame "sound" {
                    w1038 = 0.0 ("element")
                    n703 = local read "lick  #  2.2R"() -> (w1042:dbl)
                    n704 = local read "fault 2"() -> (w1030:dbl)
                    n705 = local read "water # 2.2R"() -> (w1039:dbl)
                    n706 = local read "water # 2.1L"() -> (w1040:dbl)
                    n707 = local write "state 2.2"(enum16{"waiting", "sound", "ITI"}."ITI") -> ()
                    n708 = local write "state 2.1"(enum16{"waiting", "sound", "ITI"}."ITI") -> ()
                    n709 = local read "lick  #  2.1L"() -> (w1043:dbl)
                    n710 = local write "LED 2 (i)"(1.0 ("LED 2 (i)")) -> ()
                    n711 = local read "mistake # 2.2R"() -> (w1036:dbl)
                    n712 = local read "time (s)"() -> (w1044:dbl)
                    n713 = Increment(x=w1042) -> (x+1=w1041:dbl)
                    n714 = Increment(x=w1030) -> (x+1=w1031:dbl)
                    n715 = local read "mistake # 2.1L"() -> (w1037:dbl)
                    n716 = local write "fault 2"(w1031) -> ()
                    n717 = local read "2.2"() -> (w1033:bool)
                    n718 = local write "lick  #  2.2R"(w1041) -> ()
                    n719 = case shown="True" w1033 {
                      frame False {
                      }
                      frame True {
                        n720 = local read "LED 2"() -> (w1048:tag)
                        n721 = call "_digital_on.vi"("digital port"=w1048) -> ()  [unwired: 11 in]
                      }
                    }
                    n722 = local read "Mouse path 2"() -> (w1047:path)
                    n723 = Build Array(w1044, w1043, w1041, w1040, w1039, w1038, w1038, w1038, w1038, w1038, w1038, w1037, w1036) -> (w1045:dbl[])
                    n724 = call-poly <vilib>:"Write To Spreadsheet File.vi"("append to file? (new file:F)"=TRUE, "1D data"=w1045, "file path (dialog if empty)"=w1047) -> ()  [unwired: 5 in, 1 out]
                  }
                }
              }
            }
          }
          frame 3 {
            n725 = case shown="True" w1099 {
              frame False {
              }
              frame True {
                n726 = local read "state 2.1"() -> (w1149:enum16{"waiting", "sound", "ITI"})
                n727 = case shown="\"sound\"" w1149 {
                  frame "waiting", Default {
                    w1154 = 0.0 ("element")
                    n728 = local read "water # 2.1L"() -> (w1157:dbl)
                    n729 = local read "lick  #  2.2R"() -> (w1158:dbl)
                    n730 = local read "lick  #  2.1L"() -> (w1160:dbl)
                    n731 = local read "water # 2.2R"() -> (w1155:dbl)
                    n732 = local write "state 2.2"(enum16{"waiting", "sound", "ITI"}."ITI") -> ()
                    n733 = local write "state 2.1"(enum16{"waiting", "sound", "ITI"}."ITI") -> ()
                    n734 = local read "mistake # 2.2R"() -> (w1152:dbl)
                    n735 = Increment(x=w1157) -> (x+1=w1156:dbl)
                    n736 = local read "mistake # 2.1L"() -> (w1153:dbl)
                    n737 = Increment(x=w1160) -> (x+1=w1159:dbl)
                    n738 = local read "time (s)"() -> (w1151:dbl)
                    n739 = local read "free water 2.1"() -> (w1150:bool)
                    n740 = local write "water # 2.1L"(w1156) -> ()
                    n741 = local write "lick  #  2.1L"(w1159) -> ()
                    n742 = local write "last water 2.1L"(w1151) -> ()
                    n743 = case shown="False" w1150 {
                      frame False {
                        n744 = local read "water dur (ms) 2.1"() -> (w1167:dbl)
                        n745 = local read "water port 2.1"() -> (w1166:tag)
                        n746 = call "_digital_on_duration_off.vi"("duration (ms)"=w1167, "digital port"=w1166) -> ()  [unwired: 10 in]
                      }
                      frame True {
                      }
                    }
                    n747 = Build Array(w1151, w1159, w1158, w1156, w1155, w1154, w1154, w1154, w1154, w1154, w1154, w1153, w1152) -> (w1161:dbl[])
                    n748 = local read "Mouse path 2"() -> (w1162:path)
                    n749 = call-poly <vilib>:"Write To Spreadsheet File.vi"("append to file? (new file:F)"=TRUE, "1D data"=w1161, "file path (dialog if empty)"=w1162) -> ()  [unwired: 5 in, 1 out]
                  }
                  frame "ITI" {
                    w1170 = 0.0 ("element")
                    n750 = local read "lick  #  2.2R"() -> (w1173:dbl)
                    n751 = local read "water # 2.2R"() -> (w1171:dbl)
                    n752 = local read "water # 2.1L"() -> (w1172:dbl)
                    n753 = local read "lick  #  2.1L"() -> (w1175:dbl)
                    n754 = local read "mistake # 2.2R"() -> (w1168:dbl)
                    n755 = local read "mistake # 2.1L"() -> (w1169:dbl)
                    n756 = local read "time (s)"() -> (w1176:dbl)
                    n757 = Increment(x=w1175) -> (x+1=w1174:dbl)
                    n758 = local write "lick  #  2.1L"(w1174) -> ()
                    n759 = local read "Mouse path 2"() -> (w1178:path)
                    n760 = Build Array(w1176, w1174, w1173, w1172, w1171, w1170, w1170, w1170, w1170, w1170, w1170, w1169, w1168) -> (w1177:dbl[])
                    n761 = call-poly <vilib>:"Write To Spreadsheet File.vi"("append to file? (new file:F)"=TRUE, "1D data"=w1177, "file path (dialog if empty)"=w1178) -> ()  [unwired: 5 in, 1 out]
                  }
                  frame "sound" {
                    w1188 = 0.0 ("element")
                    n762 = local write "state 2.1"(enum16{"waiting", "sound", "ITI"}."ITI") -> ()
                    n763 = local write "state 2.2"(enum16{"waiting", "sound", "ITI"}."ITI") -> ()
                    n764 = local read "water # 2.2R"() -> (w1189:dbl)
                    n765 = local read "water # 2.1L"() -> (w1190:dbl)
                    n766 = local read "mistake # 2.2R"() -> (w1186:dbl)
                    n767 = local read "lick  #  2.1L"() -> (w1193:dbl)
                    n768 = local read "mistake # 2.1L"() -> (w1187:dbl)
                    n769 = local read "lick  #  2.2R"() -> (w1191:dbl)
                    n770 = local write "LED 2 (i)"(1.0 ("LED 2 (i)")) -> ()
                    n771 = local read "time (s)"() -> (w1194:dbl)
                    n772 = local read "2.1"() -> (w1183:bool)
                    n773 = Increment(x=w1193) -> (x+1=w1192:dbl)
                    n774 = local read "Mouse path 2"() -> (w1196:path)
                    n775 = local read "fault 2"() -> (w1180:dbl)
                    n776 = local write "lick  #  2.1L"(w1192) -> ()
                    n777 = case shown="True" w1183 {
                      frame False {
                      }
                      frame True {
                        n778 = local read "LED 2"() -> (w1198:tag)
                        n779 = call "_digital_on.vi"("digital port"=w1198) -> ()  [unwired: 11 in]
                      }
                    }
                    n780 = Build Array(w1194, w1192, w1191, w1190, w1189, w1188, w1188, w1188, w1188, w1188, w1188, w1187, w1186) -> (w1195:dbl[])
                    n781 = Increment(x=w1180) -> (x+1=w1181:dbl)
                    n782 = call-poly <vilib>:"Write To Spreadsheet File.vi"("append to file? (new file:F)"=TRUE, "1D data"=w1195, "file path (dialog if empty)"=w1196) -> ()  [unwired: 5 in, 1 out]
                    n783 = local write "fault 2"(w1181) -> ()
                  }
                }
              }
            }
            n784 = case shown="True" w1098 {
              frame False {
              }
              frame True {
                n785 = local read "state 2.1"() -> (w1100:enum16{"waiting", "sound", "ITI"})
                n786 = case shown="\"sound\"" w1100 {
                  frame "waiting", Default {
                    w1106 = 0.0 ("element")
                    n787 = local write "state 2.2"(enum16{"waiting", "sound", "ITI"}."ITI") -> ()
                    n788 = local write "state 2.1"(enum16{"waiting", "sound", "ITI"}."ITI") -> ()
                    n789 = local read "water # 2.2R"() -> (w1107:dbl)
                    n790 = local read "mistake # 2.2R"() -> (w1103:dbl)
                    n791 = local read "water # 2.1L"() -> (w1108:dbl)
                    n792 = local read "lick  #  2.2R"() -> (w1110:dbl)
                    n793 = local read "mistake # 2.1L"() -> (w1105:dbl)
                    n794 = local read "LED 2"() -> (w1102:tag)
                    n795 = local write "LED 2 (i)"(1.0 ("LED 2 (i)")) -> ()
                    n796 = local read "lick  #  2.1L"() -> (w1111:dbl)
                    n797 = local read "time (s)"() -> (w1112:dbl)
                    n798 = Increment(x=w1110) -> (x+1=w1109:dbl)
                    n799 = Increment(x=w1105) -> (x+1=w1104:dbl)
                    n800 = local write "mistake # 2.1L"(w1104) -> ()
                    n801 = call "_digital_on.vi"("digital port"=w1102) -> ()  [unwired: 11 in]
                    n802 = local write "lick  #  2.2R"(w1109) -> ()
                    n803 = local read "Mouse path 2"() -> (w1115:path)
                    n804 = Build Array(w1112, w1111, w1109, w1108, w1107, w1106, w1106, w1106, w1106, w1106, w1106, w1104, w1103) -> (w1113:dbl[])
                    n805 = call-poly <vilib>:"Write To Spreadsheet File.vi"("append to file? (new file:F)"=TRUE, "1D data"=w1113, "file path (dialog if empty)"=w1115) -> ()  [unwired: 5 in, 1 out]
                  }
                  frame "ITI" {
                    w1120 = 0.0 ("element")
                    n806 = local read "water # 2.2R"() -> (w1121:dbl)
                    n807 = local read "water # 2.1L"() -> (w1122:dbl)
                    n808 = local read "lick  #  2.2R"() -> (w1124:dbl)
                    n809 = local read "lick  #  2.1L"() -> (w1125:dbl)
                    n810 = local read "mistake # 2.2R"() -> (w1118:dbl)
                    n811 = local read "mistake # 2.1L"() -> (w1119:dbl)
                    n812 = local read "time (s)"() -> (w1126:dbl)
                    n813 = Increment(x=w1124) -> (x+1=w1123:dbl)
                    n814 = local write "lick  #  2.2R"(w1123) -> ()
                    n815 = local read "Mouse path 2"() -> (w1128:path)
                    n816 = Build Array(w1126, w1125, w1123, w1122, w1121, w1120, w1120, w1120, w1120, w1120, w1120, w1119, w1118) -> (w1127:dbl[])
                    n817 = call-poly <vilib>:"Write To Spreadsheet File.vi"("append to file? (new file:F)"=TRUE, "1D data"=w1127, "file path (dialog if empty)"=w1128) -> ()  [unwired: 5 in, 1 out]
                  }
                  frame "sound" {
                    w1138 = 0.0 ("element")
                    n818 = local read "fault 2"() -> (w1130:dbl)
                    n819 = local read "water # 2.2R"() -> (w1139:dbl)
                    n820 = local write "state 2.2"(enum16{"waiting", "sound", "ITI"}."ITI") -> ()
                    n821 = local read "water # 2.1L"() -> (w1140:dbl)
                    n822 = local read "lick  #  2.2R"() -> (w1142:dbl)
                    n823 = Increment(x=w1130) -> (x+1=w1131:dbl)
                    n824 = local write "state 2.1"(enum16{"waiting", "sound", "ITI"}."ITI") -> ()
                    n825 = local read "mistake # 2.2R"() -> (w1136:dbl)
                    n826 = local read "mistake # 2.1L"() -> (w1137:dbl)
                    n827 = local read "lick  #  2.1L"() -> (w1143:dbl)
                    n828 = local write "fault 2"(w1131) -> ()
                    n829 = Increment(x=w1142) -> (x+1=w1141:dbl)
                    n830 = local read "time (s)"() -> (w1144:dbl)
                    n831 = local read "2.2"() -> (w1132:bool)
                    n832 = local write "LED 2 (i)"(1.0 ("LED 2 (i)")) -> ()
                    n833 = local write "lick  #  2.2R"(w1141) -> ()
                    n834 = local read "Mouse path 2"() -> (w1146:path)
                    n835 = Build Array(w1144, w1143, w1141, w1140, w1139, w1138, w1138, w1138, w1138, w1138, w1138, w1137, w1136) -> (w1145:dbl[])
                    n836 = case shown="True" w1132 {
                      frame False {
                      }
                      frame True {
                        n837 = local read "LED 2"() -> (w1148:tag)
                        n838 = call "_digital_on.vi"("digital port"=w1148) -> ()  [unwired: 11 in]
                      }
                    }
                    n839 = call-poly <vilib>:"Write To Spreadsheet File.vi"("append to file? (new file:F)"=TRUE, "1D data"=w1145, "file path (dialog if empty)"=w1146) -> ()  [unwired: 5 in, 1 out]
                  }
                }
              }
            }
          }
          frame 4 {
            n840 = case shown="True" w1200 {
              frame False {
              }
              frame True {
                n841 = local read "state 2.2"() -> (w1251:enum16{"waiting", "sound", "ITI"})
                n842 = case shown="\"sound\"" w1251 {
                  frame "waiting", Default {
                    w1257 = 0.0 ("element")
                    n843 = local read "LED 2"() -> (w1253:tag)
                    n844 = local read "lick  #  2.2R"() -> (w1260:dbl)
                    n845 = local read "lick  #  2.1L"() -> (w1262:dbl)
                    n846 = local read "water # 2.2R"() -> (w1258:dbl)
                    n847 = local read "water # 2.1L"() -> (w1259:dbl)
                    n848 = local write "LED 2 (i)"(1.0 ("LED 2 (i)")) -> ()
                    n849 = local read "mistake # 2.2R"() -> (w1255:dbl)
                    n850 = local read "mistake # 2.1L"() -> (w1256:dbl)
                    n851 = local read "time (s)"() -> (w1263:dbl)
                    n852 = call "_digital_on.vi"("digital port"=w1253) -> ()  [unwired: 11 in]
                    n853 = Increment(x=w1262) -> (x+1=w1261:dbl)
                    n854 = local write "lick  #  2.1L"(w1261) -> ()
                    n855 = local read "Mouse path 2"() -> (w1265:path)
                    n856 = Increment(x=w1255) -> (x+1=w1254:dbl)
                    n857 = local write "mistake # 2.2R"(w1254) -> ()
                    n858 = Build Array(w1263, w1261, w1260, w1259, w1258, w1257, w1257, w1257, w1257, w1257, w1257, w1256, w1254) -> (w1264:dbl[])
                    n859 = call-poly <vilib>:"Write To Spreadsheet File.vi"("append to file? (new file:F)"=TRUE, "1D data"=w1264, "file path (dialog if empty)"=w1265) -> ()  [unwired: 5 in, 1 out]
                    n860 = local write "state 2.2"(enum16{"waiting", "sound", "ITI"}."ITI") -> ()
                    n861 = local write "state 2.1"(enum16{"waiting", "sound", "ITI"}."ITI") -> ()
                  }
                  frame "sound" {
                    w1277 = 0.0 ("element")
                    n862 = local read "2.1"() -> (w1271:bool)
                    n863 = local read "fault 2"() -> (w1269:dbl)
                    n864 = local write "LED 2 (i)"(1.0 ("LED 2 (i)")) -> ()
                    n865 = case shown="True" w1271 {
                      frame False {
                      }
                      frame True {
                        n866 = local read "LED 2"() -> (w1287:tag)
                        n867 = call "_digital_on.vi"("digital port"=w1287) -> ()  [unwired: 11 in]
                      }
                    }
                    n868 = local read "lick  #  2.2R"() -> (w1280:dbl)
                    n869 = local read "lick  #  2.1L"() -> (w1282:dbl)
                    n870 = local read "water # 2.2R"() -> (w1278:dbl)
                    n871 = Increment(x=w1269) -> (x+1=w1270:dbl)
                    n872 = local write "fault 2"(w1270) -> ()
                    n873 = local read "water # 2.1L"() -> (w1279:dbl)
                    n874 = local read "mistake # 2.2R"() -> (w1275:dbl)
                    n875 = local read "mistake # 2.1L"() -> (w1276:dbl)
                    n876 = local read "time (s)"() -> (w1283:dbl)
                    n877 = Increment(x=w1282) -> (x+1=w1281:dbl)
                    n878 = local write "lick  #  2.1L"(w1281) -> ()
                    n879 = local read "Mouse path 2"() -> (w1285:path)
                    n880 = Build Array(w1283, w1281, w1280, w1279, w1278, w1277, w1277, w1277, w1277, w1277, w1277, w1276, w1275) -> (w1284:dbl[])
                    n881 = call-poly <vilib>:"Write To Spreadsheet File.vi"("append to file? (new file:F)"=TRUE, "1D data"=w1284, "file path (dialog if empty)"=w1285) -> ()  [unwired: 5 in, 1 out]
                    n882 = local write "state 2.2"(enum16{"waiting", "sound", "ITI"}."ITI") -> ()
                    n883 = local write "state 2.1"(enum16{"waiting", "sound", "ITI"}."ITI") -> ()
                  }
                  frame "ITI" {
                    w1290 = 0.0 ("element")
                    n884 = local read "water # 2.1L"() -> (w1292:dbl)
                    n885 = local read "water # 2.2R"() -> (w1291:dbl)
                    n886 = local read "lick  #  2.2R"() -> (w1293:dbl)
                    n887 = local read "lick  #  2.1L"() -> (w1295:dbl)
                    n888 = local read "mistake # 2.2R"() -> (w1288:dbl)
                    n889 = local read "mistake # 2.1L"() -> (w1289:dbl)
                    n890 = local read "time (s)"() -> (w1296:dbl)
                    n891 = Increment(x=w1295) -> (x+1=w1294:dbl)
                    n892 = local write "lick  #  2.1L"(w1294) -> ()
                    n893 = local read "Mouse path 2"() -> (w1298:path)
                    n894 = Build Array(w1296, w1294, w1293, w1292, w1291, w1290, w1290, w1290, w1290, w1290, w1290, w1289, w1288) -> (w1297:dbl[])
                    n895 = call-poly <vilib>:"Write To Spreadsheet File.vi"("append to file? (new file:F)"=TRUE, "1D data"=w1297, "file path (dialog if empty)"=w1298) -> ()  [unwired: 5 in, 1 out]
                  }
                }
              }
            }
            n896 = case shown="True" w1199 {
              frame False {
              }
              frame True {
                n897 = local read "state 2.2"() -> (w1201:enum16{"waiting", "sound", "ITI"})
                n898 = case shown="\"sound\"" w1201 {
                  frame "waiting", Default {
                    w1205 = 0.0 ("element")
                    n899 = local read "water # 2.2R"() -> (w1207:dbl)
                    n900 = local read "lick  #  2.2R"() -> (w1210:dbl)
                    n901 = local read "water # 2.1L"() -> (w1208:dbl)
                    n902 = local read "lick  #  2.1L"() -> (w1211:dbl)
                    n903 = local read "mistake # 2.2R"() -> (w1203:dbl)
                    n904 = local read "time (s)"() -> (w1212:dbl)
                    n905 = local read "mistake # 2.1L"() -> (w1204:dbl)
                    n906 = Increment(x=w1210) -> (x+1=w1209:dbl)
                    n907 = Increment(x=w1207) -> (x+1=w1206:dbl)
                    n908 = local write "state 2.1"(enum16{"waiting", "sound", "ITI"}."ITI") -> ()
                    n909 = local write "state 2.2"(enum16{"waiting", "sound", "ITI"}."ITI") -> ()
                    n910 = local write "water # 2.2R"(w1206) -> ()
                    n911 = local write "lick  #  2.2R"(w1209) -> ()
                    n912 = local read "Mouse path 2"() -> (w1214:path)
                    n913 = Build Array(w1212, w1211, w1209, w1208, w1206, w1205, w1205, w1205, w1205, w1205, w1205, w1204, w1203) -> (w1213:dbl[])
                    n914 = call-poly <vilib>:"Write To Spreadsheet File.vi"("append to file? (new file:F)"=TRUE, "1D data"=w1213, "file path (dialog if empty)"=w1214) -> ()  [unwired: 5 in, 1 out]
                    n915 = local read "free water 2.2"() -> (w1202:bool)
                    n916 = case shown="False" w1202 {
                      frame False {
                        n917 = local read "water dur (ms) 2.2"() -> (w1219:dbl)
                        n918 = local read "water port 2.2"() -> (w1218:tag)
                        n919 = call "_digital_on_duration_off.vi"("duration (ms)"=w1219, "digital port"=w1218) -> ()  [unwired: 10 in]
                      }
                      frame True {
                      }
                    }
                  }
                  frame "sound" {
                    w1228 = 0.0 ("element")
                    n920 = local read "2.2"() -> (w1222:bool)
                    n921 = local write "LED 2 (i)"(1.0 ("LED 2 (i)")) -> ()
                    n922 = local read "fault 2"() -> (w1220:dbl)
                    n923 = case shown="True" w1222 {
                      frame False {
                      }
                      frame True {
                        n924 = local read "LED 2"() -> (w1238:tag)
                        n925 = call "_digital_on.vi"("digital port"=w1238) -> ()  [unwired: 11 in]
                      }
                    }
                    n926 = local read "water # 2.1L"() -> (w1230:dbl)
                    n927 = local read "water # 2.2R"() -> (w1229:dbl)
                    n928 = local read "lick  #  2.2R"() -> (w1232:dbl)
                    n929 = local read "lick  #  2.1L"() -> (w1233:dbl)
                    n930 = Increment(x=w1220) -> (x+1=w1221:dbl)
                    n931 = local read "mistake # 2.2R"() -> (w1226:dbl)
                    n932 = local read "mistake # 2.1L"() -> (w1227:dbl)
                    n933 = local read "time (s)"() -> (w1234:dbl)
                    n934 = local write "fault 2"(w1221) -> ()
                    n935 = Increment(x=w1232) -> (x+1=w1231:dbl)
                    n936 = local write "lick  #  2.2R"(w1231) -> ()
                    n937 = local read "Mouse path 2"() -> (w1237:path)
                    n938 = Build Array(w1234, w1233, w1231, w1230, w1229, w1228, w1228, w1228, w1228, w1228, w1228, w1227, w1226) -> (w1235:dbl[])
                    n939 = local write "state 2.2"(enum16{"waiting", "sound", "ITI"}."ITI") -> ()
                    n940 = local write "state 2.1"(enum16{"waiting", "sound", "ITI"}."ITI") -> ()
                    n941 = call-poly <vilib>:"Write To Spreadsheet File.vi"("append to file? (new file:F)"=TRUE, "1D data"=w1235, "file path (dialog if empty)"=w1237) -> ()  [unwired: 5 in, 1 out]
                  }
                  frame "ITI" {
                    w1241 = 0.0 ("element")
                    n942 = local read "water # 2.2R"() -> (w1242:dbl)
                    n943 = local read "water # 2.1L"() -> (w1243:dbl)
                    n944 = local read "lick  #  2.2R"() -> (w1245:dbl)
                    n945 = local read "lick  #  2.1L"() -> (w1246:dbl)
                    n946 = local read "time (s)"() -> (w1247:dbl)
                    n947 = Increment(x=w1245) -> (x+1=w1244:dbl)
                    n948 = local read "mistake # 2.2R"() -> (w1239:dbl)
                    n949 = local read "mistake # 2.1L"() -> (w1240:dbl)
                    n950 = local write "lick  #  2.2R"(w1244) -> ()
                    n951 = local read "Mouse path 2"() -> (w1248:path)
                    n952 = Build Array(w1247, w1246, w1244, w1243, w1242, w1241, w1241, w1241, w1241, w1241, w1241, w1240, w1239) -> (w1249:dbl[])
                    n953 = call-poly <vilib>:"Write To Spreadsheet File.vi"("append to file? (new file:F)"=TRUE, "1D data"=w1249, "file path (dialog if empty)"=w1248) -> ()  [unwired: 5 in, 1 out]
                  }
                }
              }
            }
          }
        }
        n954 = case shown="4" w44 {
          tunnel: w33 -> [_ w90 w192 w293 w394]
          tunnel: w34 -> [_ w91 w191 w292 w393]
          frame 0, Default {
          }
          frame 1 {
            n955 = case shown="True" w91 {
              frame False {
              }
              frame True {
                n956 = local read "state 4.1"() -> (w142:enum16{"waiting", "sound", "ITI"})
                n957 = case shown="\"sound\"" w142 {
                  frame "waiting", Default {
                    w148 = 0.0 ("element")
                    n958 = local read "water # 4.1L"() -> (w150:dbl)
                    n959 = local read "water # 4.2R"() -> (w149:dbl)
                    n960 = local read "lick # 4.2R"() -> (w152:dbl)
                    n961 = local read "lick # 4.1L"() -> (w153:dbl)
                    n962 = local write "state 4.2"(enum16{"waiting", "sound", "ITI"}."ITI") -> ()
                    n963 = local read "mistake # 4.2R"() -> (w145:dbl)
                    n964 = local write "state 4.1"(enum16{"waiting", "sound", "ITI"}."ITI") -> ()
                    n965 = local read "mistake # 4.1L"() -> (w147:dbl)
                    n966 = Increment(x=w152) -> (x+1=w151:dbl)
                    n967 = local read "time (s)"() -> (w154:dbl)
                    n968 = local write "lick # 4.2R"(w151) -> ()
                    n969 = Increment(x=w147) -> (x+1=w146:dbl)
                    n970 = local read "Mouse path 4"() -> (w156:path)
                    n971 = local write "mistake # 4.1L"(w146) -> ()
                    n972 = local read "LED 4"() -> (w143:tag)
                    n973 = local write "LED 4 (i)"(1.0 ("LED 4 (i)")) -> ()
                    n974 = Build Array(w154, w153, w151, w150, w149, w148, w148, w148, w148, w148, w148, w146, w145) -> (w155:dbl[])
                    n975 = call "_digital_on.vi"("digital port"=w143) -> ()  [unwired: 11 in]
                    n976 = call-poly <vilib>:"Write To Spreadsheet File.vi"("append to file? (new file:F)"=TRUE, "1D data"=w155, "file path (dialog if empty)"=w156) -> ()  [unwired: 5 in, 1 out]
                  }
                  frame "sound" {
                    w168 = 0.0 ("element")
                    n977 = local read "fault 4"() -> (w162:dbl)
                    n978 = local read "water # 4.2R"() -> (w169:dbl)
                    n979 = local write "LED 4 (i)"(1.0 ("LED 4 (i)")) -> ()
                    n980 = local read "lick # 4.2R"() -> (w172:dbl)
                    n981 = local read "water # 4.1L"() -> (w170:dbl)
                    n982 = Increment(x=w162) -> (x+1=w161:dbl)
                    n983 = local read "lick # 4.1L"() -> (w173:dbl)
                    n984 = local write "fault 4"(w161) -> ()
                    n985 = local read "mistake # 4.2R"() -> (w166:dbl)
                    n986 = local read "time (s)"() -> (w174:dbl)
                    n987 = Increment(x=w172) -> (x+1=w171:dbl)
                    n988 = local read "mistake # 4.1L"() -> (w167:dbl)
                    n989 = local write "state 4.2"(enum16{"waiting", "sound", "ITI"}."ITI") -> ()
                    n990 = local write "state 4.1"(enum16{"waiting", "sound", "ITI"}."ITI") -> ()
                    n991 = local write "lick # 4.2R"(w171) -> ()
                    n992 = local read "4.2"() -> (w163:bool)
                    n993 = local read "Mouse path 4"() -> (w176:path)
                    n994 = case shown="True" w163 {
                      frame False {
                      }
                      frame True {
                        n995 = local read "LED 4"() -> (w178:tag)
                        n996 = call "_digital_on.vi"("digital port"=w178) -> ()  [unwired: 11 in]
                      }
                    }
                    n997 = Build Array(w174, w173, w171, w170, w169, w168, w168, w168, w168, w168, w168, w167, w166) -> (w175:dbl[])
                    n998 = call-poly <vilib>:"Write To Spreadsheet File.vi"("append to file? (new file:F)"=TRUE, "1D data"=w175, "file path (dialog if empty)"=w176) -> ()  [unwired: 5 in, 1 out]
                  }
                  frame "ITI" {
                    w181 = 0.0 ("element")
                    n999 = local read "mistake # 4.2R"() -> (w179:dbl)
                    n1000 = local read "water # 4.2R"() -> (w182:dbl)
                    n1001 = local read "mistake # 4.1L"() -> (w180:dbl)
                    n1002 = local read "water # 4.1L"() -> (w183:dbl)
                    n1003 = local read "lick # 4.2R"() -> (w185:dbl)
                    n1004 = local read "lick # 4.1L"() -> (w186:dbl)
                    n1005 = local read "time (s)"() -> (w187:dbl)
                    n1006 = Increment(x=w185) -> (x+1=w184:dbl)
                    n1007 = local write "lick # 4.2R"(w184) -> ()
                    n1008 = local read "Mouse path 4"() -> (w189:path)
                    n1009 = Build Array(w187, w186, w184, w183, w182, w181, w181, w181, w181, w181, w181, w180, w179) -> (w188:dbl[])
                    n1010 = call-poly <vilib>:"Write To Spreadsheet File.vi"("append to file? (new file:F)"=TRUE, "1D data"=w188, "file path (dialog if empty)"=w189) -> ()  [unwired: 5 in, 1 out]
                  }
                }
              }
            }
            n1011 = case shown="True" w90 {
              frame False {
              }
              frame True {
                n1012 = local read "state 4.1"() -> (w92:enum16{"waiting", "sound", "ITI"})
                n1013 = case shown="\"sound\"" w92 {
                  frame "waiting", Default {
                    w96 = 0.0 ("element")
                    n1014 = local read "water # 4.1L"() -> (w99:dbl)
                    n1015 = local read "lick # 4.2R"() -> (w100:dbl)
                    n1016 = local read "lick # 4.1L"() -> (w102:dbl)
                    n1017 = local read "water # 4.2R"() -> (w97:dbl)
                    n1018 = local read "mistake # 4.2R"() -> (w94:dbl)
                    n1019 = local read "time (s)"() -> (w93:dbl)
                    n1020 = local read "mistake # 4.1L"() -> (w95:dbl)
                    n1021 = Increment(x=w99) -> (x+1=w98:dbl)
                    n1022 = Increment(x=w102) -> (x+1=w101:dbl)
                    n1023 = local write "state 4.2"(enum16{"waiting", "sound", "ITI"}."ITI") -> ()
                    n1024 = local write "state 4.1"(enum16{"waiting", "sound", "ITI"}."ITI") -> ()
                    n1025 = local write "water # 4.1L"(w98) -> ()
                    n1026 = local write "last water 4.1L"(w93) -> ()
                    n1027 = local write "lick # 4.1L"(w101) -> ()
                    n1028 = local read "Mouse path 4"() -> (w104:path)
                    n1029 = Build Array(w93, w101, w100, w98, w97, w96, w96, w96, w96, w96, w96, w95, w94) -> (w103:dbl[])
                    n1030 = local read "free water 4.1"() -> (w106:bool)
                    n1031 = call-poly <vilib>:"Write To Spreadsheet File.vi"("append to file? (new file:F)"=TRUE, "1D data"=w103, "file path (dialog if empty)"=w104) -> ()  [unwired: 5 in, 1 out]
                    n1032 = case shown="False" w106 {
                      frame False {
                        n1033 = call "_digital_on_duration_off.vi"("duration (ms)"="water dur (ms) 4.1", "digital port"="water port 4.1") -> ()  [unwired: 10 in]
                      }
                      frame True {
                      }
                    }
                  }
                  frame "sound" {
                    w119 = 0.0 ("element")
                    n1034 = local read "fault 4"() -> (w112:dbl)
                    n1035 = local read "water # 4.2R"() -> (w120:dbl)
                    n1036 = local read "water # 4.1L"() -> (w121:dbl)
                    n1037 = local read "mistake # 4.2R"() -> (w117:dbl)
                    n1038 = local read "lick # 4.2R"() -> (w122:dbl)
                    n1039 = local read "mistake # 4.1L"() -> (w118:dbl)
                    n1040 = local read "lick # 4.1L"() -> (w124:dbl)
                    n1041 = Increment(x=w112) -> (x+1=w111:dbl)
                    n1042 = local write "LED 4 (i)"(1.0 ("LED 4 (i)")) -> ()
                    n1043 = local read "time (s)"() -> (w125:dbl)
                    n1044 = local write "state 4.1"(enum16{"waiting", "sound", "ITI"}."ITI") -> ()
                    n1045 = local write "state 4.2"(enum16{"waiting", "sound", "ITI"}."ITI") -> ()
                    n1046 = local write "fault 4"(w111) -> ()
                    n1047 = Increment(x=w124) -> (x+1=w123:dbl)
                    n1048 = local write "lick # 4.1L"(w123) -> ()
                    n1049 = local read "4.1"() -> (w113:bool)
                    n1050 = local read "Mouse path 4"() -> (w127:path)
                    n1051 = Build Array(w125, w123, w122, w121, w120, w119, w119, w119, w119, w119, w119, w118, w117) -> (w126:dbl[])
                    n1052 = case shown="True" w113 {
                      frame False {
                      }
                      frame True {
                        n1053 = local read "LED 4"() -> (w129:tag)
                        n1054 = call "_digital_on.vi"("digital port"=w129) -> ()  [unwired: 11 in]
                      }
                    }
                    n1055 = call-poly <vilib>:"Write To Spreadsheet File.vi"("append to file? (new file:F)"=TRUE, "1D data"=w126, "file path (dialog if empty)"=w127) -> ()  [unwired: 5 in, 1 out]
                  }
                  frame "ITI" {
                    w132 = 0.0 ("element")
                    n1056 = local read "water # 4.2R"() -> (w133:dbl)
                    n1057 = local read "water # 4.1L"() -> (w134:dbl)
                    n1058 = local read "mistake # 4.2R"() -> (w130:dbl)
                    n1059 = local read "lick # 4.2R"() -> (w135:dbl)
                    n1060 = local read "mistake # 4.1L"() -> (w131:dbl)
                    n1061 = local read "lick # 4.1L"() -> (w137:dbl)
                    n1062 = local read "time (s)"() -> (w138:dbl)
                    n1063 = Increment(x=w137) -> (x+1=w136:dbl)
                    n1064 = local write "lick # 4.1L"(w136) -> ()
                    n1065 = local read "Mouse path 4"() -> (w140:path)
                    n1066 = Build Array(w138, w136, w135, w134, w133, w132, w132, w132, w132, w132, w132, w131, w130) -> (w139:dbl[])
                    n1067 = call-poly <vilib>:"Write To Spreadsheet File.vi"("append to file? (new file:F)"=TRUE, "1D data"=w139, "file path (dialog if empty)"=w140) -> ()  [unwired: 5 in, 1 out]
                  }
                }
              }
            }
          }
          frame 2 {
            n1068 = case shown="True" w191 {
              frame False {
              }
              frame True {
                n1069 = local read "state 4.2"() -> (w242:enum16{"waiting", "sound", "ITI"})
                n1070 = case shown="\"sound\"" w242 {
                  frame "waiting", Default {
                    w246 = 0.0 ("element")
                    n1071 = local read "water # 4.2R"() -> (w248:dbl)
                    n1072 = local read "mistake # 4.2R"() -> (w244:dbl)
                    n1073 = local read "mistake # 4.1L"() -> (w245:dbl)
                    n1074 = local read "water # 4.1L"() -> (w249:dbl)
                    n1075 = local read "lick # 4.2R"() -> (w251:dbl)
                    n1076 = local write "state 4.2"(enum16{"waiting", "sound", "ITI"}."ITI") -> ()
                    n1077 = local write "state 4.1"(enum16{"waiting", "sound", "ITI"}."ITI") -> ()
                    n1078 = local read "lick # 4.1L"() -> (w252:dbl)
                    n1079 = Increment(x=w248) -> (x+1=w247:dbl)
                    n1080 = local read "time (s)"() -> (w243:dbl)
                    n1081 = local write "water # 4.2R"(w247) -> ()
                    n1082 = Increment(x=w251) -> (x+1=w250:dbl)
                    n1083 = local write "last water 4.2R"(w243) -> ()
                    n1084 = local read "free water 4.2"() -> (w256:bool)
                    n1085 = local write "lick # 4.2R"(w250) -> ()
                    n1086 = Build Array(w243, w252, w250, w249, w247, w246, w246, w246, w246, w246, w246, w245, w244) -> (w253:dbl[])
                    n1087 = local read "Mouse path 4"() -> (w254:path)
                    n1088 = case shown="False" w256 {
                      frame False {
                        n1089 = call "_digital_on_duration_off.vi"("duration (ms)"="water dur (ms) 4.2", "digital port"="water port 4.2") -> ()  [unwired: 10 in]
                      }
                      frame True {
                      }
                    }
                    n1090 = call-poly <vilib>:"Write To Spreadsheet File.vi"("append to file? (new file:F)"=TRUE, "1D data"=w253, "file path (dialog if empty)"=w254) -> ()  [unwired: 5 in, 1 out]
                  }
                  frame "sound" {
                    w269 = 0.0 ("element")
                    n1091 = local read "fault 4"() -> (w264:dbl)
                    n1092 = local read "water # 4.1L"() -> (w271:dbl)
                    n1093 = local read "water # 4.2R"() -> (w270:dbl)
                    n1094 = local read "mistake # 4.2R"() -> (w267:dbl)
                    n1095 = local read "lick # 4.2R"() -> (w273:dbl)
                    n1096 = local write "state 4.2"(enum16{"waiting", "sound", "ITI"}."ITI") -> ()
                    n1097 = local write "state 4.1"(enum16{"waiting", "sound", "ITI"}."ITI") -> ()
                    n1098 = local read "mistake # 4.1L"() -> (w268:dbl)
                    n1099 = local read "lick # 4.1L"() -> (w274:dbl)
                    n1100 = Increment(x=w264) -> (x+1=w263:dbl)
                    n1101 = local read "time (s)"() -> (w275:dbl)
                    n1102 = Increment(x=w273) -> (x+1=w272:dbl)
                    n1103 = local write "fault 4"(w263) -> ()
                    n1104 = local write "lick # 4.2R"(w272) -> ()
                    n1105 = local read "4.2"() -> (w262:bool)
                    n1106 = Build Array(w275, w274, w272, w271, w270, w269, w269, w269, w269, w269, w269, w268, w267) -> (w276:dbl[])
                    n1107 = local read "Mouse path 4"() -> (w277:path)
                    n1108 = case shown="True" w262 {
                      frame False {
                      }
                      frame True {
                        n1109 = local read "LED 4"() -> (w279:tag)
                        n1110 = call "_digital_on.vi"("digital port"=w279) -> ()  [unwired: 11 in]
                      }
                    }
                    n1111 = local write "LED 4 (i)"(1.0 ("LED 4 (i)")) -> ()
                    n1112 = call-poly <vilib>:"Write To Spreadsheet File.vi"("append to file? (new file:F)"=TRUE, "1D data"=w276, "file path (dialog if empty)"=w277) -> ()  [unwired: 5 in, 1 out]
                  }
                  frame "ITI" {
                    w282 = 0.0 ("element")
                    n1113 = local read "water # 4.2R"() -> (w283:dbl)
                    n1114 = local read "water # 4.1L"() -> (w284:dbl)
                    n1115 = local read "lick # 4.2R"() -> (w286:dbl)
                    n1116 = local read "lick # 4.1L"() -> (w287:dbl)
                    n1117 = local read "mistake # 4.2R"() -> (w280:dbl)
                    n1118 = Increment(x=w286) -> (x+1=w285:dbl)
                    n1119 = local read "mistake # 4.1L"() -> (w281:dbl)
                    n1120 = local read "time (s)"() -> (w288:dbl)
                    n1121 = local write "lick # 4.2R"(w285) -> ()
                    n1122 = Build Array(w288, w287, w285, w284, w283, w282, w282, w282, w282, w282, w282, w281, w280) -> (w289:dbl[])
                    n1123 = local read "Mouse path 4"() -> (w290:path)
                    n1124 = call-poly <vilib>:"Write To Spreadsheet File.vi"("append to file? (new file:F)"=TRUE, "1D data"=w289, "file path (dialog if empty)"=w290) -> ()  [unwired: 5 in, 1 out]
                  }
                }
              }
            }
            n1125 = case shown="True" w192 {
              frame False {
              }
              frame True {
                n1126 = local read "state 4.2"() -> (w193:enum16{"waiting", "sound", "ITI"})
                n1127 = case shown="\"sound\"" w193 {
                  frame "waiting", Default {
                    w199 = 0.0 ("element")
                    n1128 = local read "lick # 4.2R"() -> (w202:dbl)
                    n1129 = local read "lick # 4.1L"() -> (w204:dbl)
                    n1130 = local read "mistake # 4.2R"() -> (w197:dbl)
                    n1131 = local read "water # 4.1L"() -> (w201:dbl)
                    n1132 = local read "water # 4.2R"() -> (w200:dbl)
                    n1133 = local read "time (s)"() -> (w205:dbl)
                    n1134 = local read "mistake # 4.1L"() -> (w198:dbl)
                    n1135 = local write "state 4.2"(enum16{"waiting", "sound", "ITI"}."ITI") -> ()
                    n1136 = local write "state 4.1"(enum16{"waiting", "sound", "ITI"}."ITI") -> ()
                    n1137 = Increment(x=w204) -> (x+1=w203:dbl)
                    n1138 = Increment(x=w197) -> (x+1=w196:dbl)
                    n1139 = local write "mistake # 4.2R"(w196) -> ()
                    n1140 = local write "lick # 4.1L"(w203) -> ()
                    n1141 = call "_digital_on.vi"("digital port"="LED 4") -> ()  [unwired: 11 in]
                    n1142 = Build Array(w205, w203, w202, w201, w200, w199, w199, w199, w199, w199, w199, w198, w196) -> (w206:dbl[])
                    n1143 = local read "Mouse path 4"() -> (w207:path)
                    n1144 = local write "LED 4 (i)"(1.0 ("LED 4 (i)")) -> ()
                    n1145 = call-poly <vilib>:"Write To Spreadsheet File.vi"("append to file? (new file:F)"=TRUE, "1D data"=w206, "file path (dialog if empty)"=w207) -> ()  [unwired: 5 in, 1 out]
                  }
                  frame "sound" {
                    w219 = 0.0 ("element")
                    n1146 = local read "mistake # 4.2R"() -> (w217:dbl)
                    n1147 = local read "fault 4"() -> (w214:dbl)
                    n1148 = local read "water # 4.2R"() -> (w220:dbl)
                    n1149 = local read "mistake # 4.1L"() -> (w218:dbl)
                    n1150 = local read "water # 4.1L"() -> (w221:dbl)
                    n1151 = local read "lick # 4.2R"() -> (w222:dbl)
                    n1152 = local read "lick # 4.1L"() -> (w224:dbl)
                    n1153 = local write "state 4.1"(enum16{"waiting", "sound", "ITI"}."ITI") -> ()
                    n1154 = Increment(x=w214) -> (x+1=w213:dbl)
                    n1155 = local write "state 4.2"(enum16{"waiting", "sound", "ITI"}."ITI") -> ()
                    n1156 = local write "LED 4 (i)"(1.0 ("LED 4 (i)")) -> ()
                    n1157 = local read "time (s)"() -> (w225:dbl)
                    n1158 = local write "fault 4"(w213) -> ()
                    n1159 = Increment(x=w224) -> (x+1=w223:dbl)
                    n1160 = local read "4.1"() -> (w211:bool)
                    n1161 = local write "lick # 4.1L"(w223) -> ()
                    n1162 = Build Array(w225, w223, w222, w221, w220, w219, w219, w219, w219, w219, w219, w218, w217) -> (w226:dbl[])
                    n1163 = local read "Mouse path 4"() -> (w227:path)
                    n1164 = case shown="True" w211 {
                      frame False {
                      }
                      frame True {
                        n1165 = local read "LED 4"() -> (w229:tag)
                        n1166 = call "_digital_on.vi"("digital port"=w229) -> ()  [unwired: 11 in]
                      }
                    }
                    n1167 = call-poly <vilib>:"Write To Spreadsheet File.vi"("append to file? (new file:F)"=TRUE, "1D data"=w226, "file path (dialog if empty)"=w227) -> ()  [unwired: 5 in, 1 out]
                  }
                  frame "ITI" {
                    w232 = 0.0 ("element")
                    n1168 = local read "water # 4.1L"() -> (w234:dbl)
                    n1169 = local read "water # 4.2R"() -> (w233:dbl)
                    n1170 = local read "lick # 4.2R"() -> (w235:dbl)
                    n1171 = local read "mistake # 4.2R"() -> (w230:dbl)
                    n1172 = local read "lick # 4.1L"() -> (w237:dbl)
                    n1173 = local read "mistake # 4.1L"() -> (w231:dbl)
                    n1174 = local read "time (s)"() -> (w238:dbl)
                    n1175 = Increment(x=w237) -> (x+1=w236:dbl)
                    n1176 = local write "lick # 4.1L"(w236) -> ()
                    n1177 = local read "Mouse path 4"() -> (w240:path)
                    n1178 = Build Array(w238, w236, w235, w234, w233, w232, w232, w232, w232, w232, w232, w231, w230) -> (w239:dbl[])
                    n1179 = call-poly <vilib>:"Write To Spreadsheet File.vi"("append to file? (new file:F)"=TRUE, "1D data"=w239, "file path (dialog if empty)"=w240) -> ()  [unwired: 5 in, 1 out]
                  }
                }
              }
            }
          }
          frame 3 {
            n1180 = case shown="True" w292 {
              frame False {
              }
              frame True {
                n1181 = local read "state 4.1"() -> (w344:enum16{"waiting", "sound", "ITI"})
                n1182 = case shown="\"sound\"" w344 {
                  frame "waiting", Default {
                    w350 = 0.0 ("element")
                    n1183 = local write "state 4.2"(enum16{"waiting", "sound", "ITI"}."ITI") -> ()
                    n1184 = local write "state 4.1"(enum16{"waiting", "sound", "ITI"}."ITI") -> ()
                    n1185 = local read "water # 4.2R"() -> (w351:dbl)
                    n1186 = local read "mistake # 4.1L"() -> (w349:dbl)
                    n1187 = local read "water # 4.1L"() -> (w352:dbl)
                    n1188 = local read "mistake # 4.2R"() -> (w347:dbl)
                    n1189 = local read "lick # 4.2R"() -> (w354:dbl)
                    n1190 = local read "lick # 4.1L"() -> (w355:dbl)
                    n1191 = local read "time (s)"() -> (w356:dbl)
                    n1192 = Increment(x=w349) -> (x+1=w348:dbl)
                    n1193 = Increment(x=w354) -> (x+1=w353:dbl)
                    n1194 = local write "mistake # 4.1L"(w348) -> ()
                    n1195 = local write "lick # 4.2R"(w353) -> ()
                    n1196 = local read "Mouse path 4"() -> (w358:path)
                    n1197 = local read "LED 4"() -> (w345:tag)
                    n1198 = local write "LED 4 (i)"(1.0 ("LED 4 (i)")) -> ()
                    n1199 = Build Array(w356, w355, w353, w352, w351, w350, w350, w350, w350, w350, w350, w348, w347) -> (w357:dbl[])
                    n1200 = call "_digital_on.vi"("digital port"=w345) -> ()  [unwired: 11 in]
                    n1201 = call-poly <vilib>:"Write To Spreadsheet File.vi"("append to file? (new file:F)"=TRUE, "1D data"=w357, "file path (dialog if empty)"=w358) -> ()  [unwired: 5 in, 1 out]
                  }
                  frame "sound" {
                    w371 = 0.0 ("element")
                    n1202 = local read "lick # 4.2R"() -> (w375:dbl)
                    n1203 = local read "water # 4.1L"() -> (w373:dbl)
                    n1204 = local read "water # 4.2R"() -> (w372:dbl)
                    n1205 = local read "mistake # 4.2R"() -> (w369:dbl)
                    n1206 = local read "lick # 4.1L"() -> (w376:dbl)
                    n1207 = local read "time (s)"() -> (w377:dbl)
                    n1208 = local read "mistake # 4.1L"() -> (w370:dbl)
                    n1209 = local write "state 4.2"(enum16{"waiting", "sound", "ITI"}."ITI") -> ()
                    n1210 = local write "state 4.1"(enum16{"waiting", "sound", "ITI"}."ITI") -> ()
                    n1211 = Increment(x=w375) -> (x+1=w374:dbl)
                    n1212 = local write "LED 4 (i)"(1.0 ("LED 4 (i)")) -> ()
                    n1213 = local write "lick # 4.2R"(w374) -> ()
                    n1214 = local read "4.2"() -> (w366:bool)
                    n1215 = Build Array(w377, w376, w374, w373, w372, w371, w371, w371, w371, w371, w371, w370, w369) -> (w378:dbl[])
                    n1216 = local read "fault 4"() -> (w364:dbl)
                    n1217 = local read "Mouse path 4"() -> (w379:path)
                    n1218 = case shown="True" w366 {
                      frame False {
                      }
                      frame True {
                        (unwired) TRUE ("append to file? (new file:F)")
                        n1219 = local read "LED 4"() -> (w380:tag)
                        n1220 = call "_digital_on.vi"("digital port"=w380) -> ()  [unwired: 11 in]
                      }
                    }
                    n1221 = Increment(x=w364) -> (x+1=w363:dbl)
                    n1222 = call-poly <vilib>:"Write To Spreadsheet File.vi"("append to file? (new file:F)"=TRUE, "1D data"=w378, "file path (dialog if empty)"=w379) -> ()  [unwired: 5 in, 1 out]
                    n1223 = local write "fault 4"(w363) -> ()
                  }
                  frame "ITI" {
                    w383 = 0.0 ("element")
                    n1224 = local read "water # 4.2R"() -> (w384:dbl)
                    n1225 = local read "water # 4.1L"() -> (w385:dbl)
                    n1226 = local read "mistake # 4.1L"() -> (w382:dbl)
                    n1227 = local read "mistake # 4.2R"() -> (w381:dbl)
                    n1228 = local read "lick # 4.2R"() -> (w387:dbl)
                    n1229 = local read "lick # 4.1L"() -> (w388:dbl)
                    n1230 = local read "time (s)"() -> (w389:dbl)
                    n1231 = Increment(x=w387) -> (x+1=w386:dbl)
                    n1232 = local write "lick # 4.2R"(w386) -> ()
                    n1233 = local read "Mouse path 4"() -> (w391:path)
                    n1234 = Build Array(w389, w388, w386, w385, w384, w383, w383, w383, w383, w383, w383, w382, w381) -> (w390:dbl[])
                    n1235 = call-poly <vilib>:"Write To Spreadsheet File.vi"("append to file? (new file:F)"=TRUE, "1D data"=w390, "file path (dialog if empty)"=w391) -> ()  [unwired: 5 in, 1 out]
                  }
                }
              }
            }
            n1236 = case shown="True" w293 {
              frame False {
              }
              frame True {
                n1237 = local read "state 4.1"() -> (w294:enum16{"waiting", "sound", "ITI"})
                n1238 = case shown="\"sound\"" w294 {
                  frame "waiting", Default {
                    w298 = 0.0 ("element")
                    n1239 = local read "water # 4.1L"() -> (w301:dbl)
                    n1240 = local write "state 4.2"(enum16{"waiting", "sound", "ITI"}."ITI") -> ()
                    n1241 = local read "water # 4.2R"() -> (w299:dbl)
                    n1242 = local write "state 4.1"(enum16{"waiting", "sound", "ITI"}."ITI") -> ()
                    n1243 = local read "lick # 4.2R"() -> (w302:dbl)
                    n1244 = local read "lick # 4.1L"() -> (w304:dbl)
                    n1245 = local read "time (s)"() -> (w295:dbl)
                    n1246 = local read "mistake # 4.2R"() -> (w296:dbl)
                    n1247 = Increment(x=w301) -> (x+1=w300:dbl)
                    n1248 = local read "mistake # 4.1L"() -> (w297:dbl)
                    n1249 = Increment(x=w304) -> (x+1=w303:dbl)
                    n1250 = local write "water # 4.1L"(w300) -> ()
                    n1251 = local write "last water 4.1L"(w295) -> ()
                    n1252 = local read "free water 4.1"() -> (w310:bool)
                    n1253 = local write "lick # 4.1L"(w303) -> ()
                    n1254 = local read "Mouse path 4"() -> (w306:path)
                    n1255 = Build Array(w295, w303, w302, w300, w299, w298, w298, w298, w298, w298, w298, w297, w296) -> (w305:dbl[])
                    n1256 = case shown="False" w310 {
                      frame False {
                        n1257 = local read "water dur (ms) 4.1"() -> (w311:dbl)
                        n1258 = local read "water port 4.1"() -> (w312:tag)
                        n1259 = call "_digital_on_duration_off.vi"("duration (ms)"=w311, "digital port"=w312) -> ()  [unwired: 10 in]
                      }
                      frame True {
                      }
                    }
                    n1260 = call-poly <vilib>:"Write To Spreadsheet File.vi"("append to file? (new file:F)"=TRUE, "1D data"=w305, "file path (dialog if empty)"=w306) -> ()  [unwired: 5 in, 1 out]
                  }
                  frame "sound" {
                    w321 = 0.0 ("element")
                    n1261 = local read "fault 4"() -> (w314:dbl)
                    n1262 = local read "water # 4.1L"() -> (w323:dbl)
                    n1263 = local read "water # 4.2R"() -> (w322:dbl)
                    n1264 = local read "lick # 4.2R"() -> (w324:dbl)
                    n1265 = Increment(x=w314) -> (x+1=w313:dbl)
                    n1266 = local read "lick # 4.1L"() -> (w326:dbl)
                    n1267 = local write "state 4.2"(enum16{"waiting", "sound", "ITI"}."ITI") -> ()
                    n1268 = local write "fault 4"(w313) -> ()
                    n1269 = local write "LED 4 (i)"(1.0 ("LED 4 (i)")) -> ()
                    n1270 = local write "state 4.1"(enum16{"waiting", "sound", "ITI"}."ITI") -> ()
                    n1271 = local read "mistake # 4.2R"() -> (w319:dbl)
                    n1272 = local read "mistake # 4.1L"() -> (w320:dbl)
                    n1273 = Increment(x=w326) -> (x+1=w325:dbl)
                    n1274 = local read "time (s)"() -> (w327:dbl)
                    n1275 = local write "lick # 4.1L"(w325) -> ()
                    n1276 = local read "4.1"() -> (w316:bool)
                    n1277 = Build Array(w327, w325, w324, w323, w322, w321, w321, w321, w321, w321, w321, w320, w319) -> (w328:dbl[])
                    n1278 = local read "Mouse path 4"() -> (w329:path)
                    n1279 = case shown="True" w316 {
                      frame False {
                      }
                      frame True {
                        n1280 = local read "LED 4"() -> (w331:tag)
                        n1281 = call "_digital_on.vi"("digital port"=w331) -> ()  [unwired: 11 in]
                      }
                    }
                    n1282 = call-poly <vilib>:"Write To Spreadsheet File.vi"("append to file? (new file:F)"=TRUE, "1D data"=w328, "file path (dialog if empty)"=w329) -> ()  [unwired: 5 in, 1 out]
                  }
                  frame "ITI" {
                    w334 = 0.0 ("element")
                    n1283 = local read "water # 4.2R"() -> (w335:dbl)
                    n1284 = local read "lick # 4.2R"() -> (w337:dbl)
                    n1285 = local read "water # 4.1L"() -> (w336:dbl)
                    n1286 = local read "lick # 4.1L"() -> (w339:dbl)
                    n1287 = local read "mistake # 4.1L"() -> (w333:dbl)
                    n1288 = local read "mistake # 4.2R"() -> (w332:dbl)
                    n1289 = Increment(x=w339) -> (x+1=w338:dbl)
                    n1290 = local read "time (s)"() -> (w340:dbl)
                    n1291 = local write "lick # 4.1L"(w338) -> ()
                    n1292 = local read "Mouse path 4"() -> (w342:path)
                    n1293 = Build Array(w340, w338, w337, w336, w335, w334, w334, w334, w334, w334, w334, w333, w332) -> (w341:dbl[])
                    n1294 = call-poly <vilib>:"Write To Spreadsheet File.vi"("append to file? (new file:F)"=TRUE, "1D data"=w341, "file path (dialog if empty)"=w342) -> ()  [unwired: 5 in, 1 out]
                  }
                }
              }
            }
          }
          frame 4 {
            n1295 = case shown="True" w393 {
              frame False {
              }
              frame True {
                n1296 = local read "state 4.2"() -> (w444:enum16{"waiting", "sound", "ITI"})
                n1297 = case shown="\"sound\"" w444 {
                  frame "waiting", Default {
                    w448 = 0.0 ("element")
                    n1298 = local read "water # 4.2R"() -> (w450:dbl)
                    n1299 = local read "lick # 4.2R"() -> (w453:dbl)
                    n1300 = local read "water # 4.1L"() -> (w451:dbl)
                    n1301 = local read "lick # 4.1L"() -> (w454:dbl)
                    n1302 = local read "mistake # 4.2R"() -> (w446:dbl)
                    n1303 = local read "time (s)"() -> (w445:dbl)
                    n1304 = local read "mistake # 4.1L"() -> (w447:dbl)
                    n1305 = Increment(x=w453) -> (x+1=w452:dbl)
                    n1306 = Increment(x=w450) -> (x+1=w449:dbl)
                    n1307 = local write "state 4.2"(enum16{"waiting", "sound", "ITI"}."ITI") -> ()
                    n1308 = local write "water # 4.2R"(w449) -> ()
                    n1309 = local write "lick # 4.2R"(w452) -> ()
                    n1310 = local write "last water 4.2R"(w445) -> ()
                    n1311 = local read "Mouse path 4"() -> (w456:path)
                    n1312 = local write "state 4.1"(enum16{"waiting", "sound", "ITI"}."ITI") -> ()
                    n1313 = local read "free water 4.2"() -> (w458:bool)
                    n1314 = Build Array(w445, w454, w452, w451, w449, w448, w448, w448, w448, w448, w448, w447, w446) -> (w455:dbl[])
                    n1315 = call-poly <vilib>:"Write To Spreadsheet File.vi"("append to file? (new file:F)"=TRUE, "1D data"=w455, "file path (dialog if empty)"=w456) -> ()  [unwired: 5 in, 1 out]
                    n1316 = case shown="False" w458 {
                      frame False {
                        n1317 = local read "water dur (ms) 4.2"() -> (w461:dbl)
                        n1318 = local read "water port 4.2"() -> (w462:tag)
                        n1319 = call "_digital_on_duration_off.vi"("duration (ms)"=w461, "digital port"=w462) -> ()  [unwired: 10 in]
                      }
                      frame True {
                      }
                    }
                  }
                  frame "sound" {
                    w471 = 0.0 ("element")
                    n1320 = local read "fault 4"() -> (w464:dbl)
                    n1321 = local read "water # 4.2R"() -> (w472:dbl)
                    n1322 = local read "water # 4.1L"() -> (w473:dbl)
                    n1323 = local read "lick # 4.2R"() -> (w475:dbl)
                    n1324 = local write "LED 4 (i)"(1.0 ("LED 4 (i)")) -> ()
                    n1325 = Increment(x=w464) -> (x+1=w463:dbl)
                    n1326 = local read "lick # 4.1L"() -> (w476:dbl)
                    n1327 = local read "mistake # 4.2R"() -> (w469:dbl)
                    n1328 = local write "state 4.2"(enum16{"waiting", "sound", "ITI"}."ITI") -> ()
                    n1329 = local write "state 4.1"(enum16{"waiting", "sound", "ITI"}."ITI") -> ()
                    n1330 = local read "mistake # 4.1L"() -> (w470:dbl)
                    n1331 = local write "fault 4"(w463) -> ()
                    n1332 = Increment(x=w475) -> (x+1=w474:dbl)
                    n1333 = local write "lick # 4.2R"(w474) -> ()
                    n1334 = local read "time (s)"() -> (w477:dbl)
                    n1335 = local read "4.2"() -> (w466:bool)
                    n1336 = Build Array(w477, w476, w474, w473, w472, w471, w471, w471, w471, w471, w471, w470, w469) -> (w478:dbl[])
                    n1337 = local read "Mouse path 4"() -> (w479:path)
                    n1338 = case shown="True" w466 {
                      frame False {
                      }
                      frame True {
                        n1339 = local read "LED 4"() -> (w481:tag)
                        n1340 = call "_digital_on.vi"("digital port"=w481) -> ()  [unwired: 11 in]
                      }
                    }
                    n1341 = call-poly <vilib>:"Write To Spreadsheet File.vi"("append to file? (new file:F)"=TRUE, "1D data"=w478, "file path (dialog if empty)"=w479) -> ()  [unwired: 5 in, 1 out]
                  }
                  frame "ITI" {
                    w484 = 0.0 ("element")
                    n1342 = local read "water # 4.2R"() -> (w485:dbl)
                    n1343 = local read "lick # 4.2R"() -> (w488:dbl)
                    n1344 = local read "water # 4.1L"() -> (w486:dbl)
                    n1345 = local read "lick # 4.1L"() -> (w489:dbl)
                    n1346 = local read "mistake # 4.2R"() -> (w482:dbl)
                    n1347 = local read "mistake # 4.1L"() -> (w483:dbl)
                    n1348 = Increment(x=w488) -> (x+1=w487:dbl)
                    n1349 = local read "time (s)"() -> (w490:dbl)
                    n1350 = local write "lick # 4.2R"(w487) -> ()
                    n1351 = Build Array(w490, w489, w487, w486, w485, w484, w484, w484, w484, w484, w484, w483, w482) -> (w491:dbl[])
                    n1352 = local read "Mouse path 4"() -> (w492:path)
                    n1353 = call-poly <vilib>:"Write To Spreadsheet File.vi"("append to file? (new file:F)"=TRUE, "1D data"=w491, "file path (dialog if empty)"=w492) -> ()  [unwired: 5 in, 1 out]
                  }
                }
              }
            }
            n1354 = case shown="True" w394 {
              frame False {
              }
              frame True {
                n1355 = local read "state 4.2"() -> (w395:enum16{"waiting", "sound", "ITI"})
                n1356 = case shown="\"sound\"" w395 {
                  frame "waiting", Default {
                    w401 = 0.0 ("element")
                    n1357 = local read "LED 4"() -> (w397:tag)
                    n1358 = local read "water # 4.2R"() -> (w402:dbl)
                    n1359 = local read "water # 4.1L"() -> (w403:dbl)
                    n1360 = local read "lick # 4.2R"() -> (w404:dbl)
                    n1361 = local read "lick # 4.1L"() -> (w406:dbl)
                    n1362 = local write "LED 4 (i)"(1.0 ("LED 4 (i)")) -> ()
                    n1363 = local read "mistake # 4.2R"() -> (w399:dbl)
                    n1364 = local read "mistake # 4.1L"() -> (w400:dbl)
                    n1365 = local read "time (s)"() -> (w407:dbl)
                    n1366 = Increment(x=w406) -> (x+1=w405:dbl)
                    n1367 = call "_digital_on.vi"("digital port"=w397) -> ()  [unwired: 11 in]
                    n1368 = Increment(x=w399) -> (x+1=w398:dbl)
                    n1369 = local write "lick # 4.1L"(w405) -> ()
                    n1370 = local write "mistake # 4.2R"(w398) -> ()
                    n1371 = local read "Mouse path 4"() -> (w409:path)
                    n1372 = Build Array(w407, w405, w404, w403, w402, w401, w401, w401, w401, w401, w400, w398) -> (w408:dbl[])
                    n1373 = local write "state 4.1"(enum16{"waiting", "sound", "ITI"}."ITI") -> ()
                    n1374 = local write "state 4.2"(enum16{"waiting", "sound", "ITI"}."ITI") -> ()
                    n1375 = call-poly <vilib>:"Write To Spreadsheet File.vi"("append to file? (new file:F)"=TRUE, "1D data"=w408, "file path (dialog if empty)"=w409) -> ()  [unwired: 5 in, 1 out]
                  }
                  frame "sound" {
                    w421 = 0.0 ("element")
                    n1376 = local read "fault 4"() -> (w418:dbl)
                    n1377 = local read "lick # 4.2R"() -> (w424:dbl)
                    n1378 = local read "water # 4.2R"() -> (w422:dbl)
                    n1379 = local read "water # 4.1L"() -> (w423:dbl)
                    n1380 = local write "state 4.1"(enum16{"waiting", "sound", "ITI"}."ITI") -> ()
                    n1381 = local write "state 4.2"(enum16{"waiting", "sound", "ITI"}."ITI") -> ()
                    n1382 = local read "lick # 4.1L"() -> (w426:dbl)
                    n1383 = local write "LED 4 (i)"(1.0 ("LED 4 (i)")) -> ()
                    n1384 = Increment(x=w418) -> (x+1=w417:dbl)
                    n1385 = local read "mistake # 4.2R"() -> (w419:dbl)
                    n1386 = local read "mistake # 4.1L"() -> (w420:dbl)
                    n1387 = local read "time (s)"() -> (w427:dbl)
                    n1388 = local write "fault 4"(w417) -> ()
                    n1389 = Increment(x=w426) -> (x+1=w425:dbl)
                    n1390 = local read "4.1"() -> (w413:bool)
                    n1391 = local write "lick # 4.1L"(w425) -> ()
                    n1392 = local read "Mouse path 4"() -> (w429:path)
                    n1393 = Build Array(w427, w425, w424, w423, w422, w421, w421, w421, w421, w421, w421, w420, w419) -> (w428:dbl[])
                    n1394 = case shown="True" w413 {
                      frame False {
                      }
                      frame True {
                        n1395 = local read "LED 4"() -> (w431:tag)
                        n1396 = call "_digital_on.vi"("digital port"=w431) -> ()  [unwired: 11 in]
                      }
                    }
                    n1397 = call-poly <vilib>:"Write To Spreadsheet File.vi"("append to file? (new file:F)"=TRUE, "1D data"=w428, "file path (dialog if empty)"=w429) -> ()  [unwired: 5 in, 1 out]
                  }
                  frame "ITI" {
                    w434 = 0.0 ("element")
                    n1398 = local read "water # 4.2R"() -> (w435:dbl)
                    n1399 = local read "water # 4.1L"() -> (w436:dbl)
                    n1400 = local read "lick # 4.2R"() -> (w437:dbl)
                    n1401 = local read "lick # 4.1L"() -> (w439:dbl)
                    n1402 = local read "mistake # 4.1L"() -> (w433:dbl)
                    n1403 = local read "mistake # 4.2R"() -> (w432:dbl)
                    n1404 = local read "time (s)"() -> (w440:dbl)
                    n1405 = Increment(x=w439) -> (x+1=w438:dbl)
                    n1406 = local write "lick # 4.1L"(w438) -> ()
                    n1407 = local read "Mouse path 4"() -> (w442:path)
                    n1408 = Build Array(w440, w438, w437, w436, w435, w434, w434, w434, w434, w434, w434, w433, w432) -> (w441:dbl[])
                    n1409 = call-poly <vilib>:"Write To Spreadsheet File.vi"("append to file? (new file:F)"=TRUE, "1D data"=w441, "file path (dialog if empty)"=w442) -> ()  [unwired: 5 in, 1 out]
                  }
                }
              }
            }
          }
        }
        n1410 = case shown="4" w72 {
          tunnel: w74 -> [_ w1301 w1422 w1545 w1665]
          tunnel: w73 -> [_ w1300 w1423 w1544 w1664]
          frame 0, Default {
          }
          frame 1 {
            n1411 = case shown="True" w1300 {
              frame False {
              }
              frame True {
                n1412 = local read "state 1.2"() -> (w1302:enum16{"waiting", "sound", "ITI"})
                n1413 = case shown="\"sound\"" w1302 {
                  frame "waiting", Default {
                    w1313 = 0
                    n1414 = local read "LED 1"() -> (w1303:tag)
                    n1415 = local read "water # 1.2R"() -> (w1307:dbl)
                    n1416 = call "_digital_on.vi"("digital port"=w1303) -> ()  [unwired: 11 in]
                    n1417 = local read "lick # 1.2R"() -> (w1317:dbl)
                    n1418 = local read "lick # 1.1L"() -> (w1316:dbl)
                    n1419 = local read "water # 1.1L"() -> (w1319:dbl)
                    n1420 = local read "current sound"() -> (w1321:dbl)
                    n1421 = local read "time (s)"() -> (w1315:dbl)
                    n1422 = local read "trial #"() -> (w1320:dbl)
                    n1423 = local write "LED 1(i)"(1.0 ("LED 1(i)")) -> ()
                    n1424 = local read "mistake # 1.1L"() -> (w1309:dbl)
                    n1425 = Increment(x=w1317) -> (x+1=w1318:dbl)
                    n1426 = local read "mistake # 1.2R"() -> (w1311:dbl)
                    n1427 = local write "lick # 1.2R"(w1318) -> ()
                    n1428 = local write "state 1.2"(enum16{"waiting", "sound", "ITI"}."ITI") -> ()
                    n1429 = local write "state 1.1"(enum16{"waiting", "sound", "ITI"}."ITI") -> ()
                    n1430 = local read "ITI (s)"() -> (w1322:dbl)
                    n1431 = Increment(x=w1309) -> (x+1=w1308:dbl)
                    n1432 = local read "Mouse path 1"() -> (w1312:path)
                    n1433 = local write "mistake # 1.1L"(w1308) -> ()
                    n1434 = Build Array(w1315, w1316, w1318, w1319, w1307, 0.0 ("element"), w1313, w1320, w1321, w1322, w1313, w1308, w1311) -> (w1323:dbl[])
                    n1435 = call-poly <vilib>:"Write To Spreadsheet File.vi"("append to file? (new file:F)"=TRUE, "1D data"=w1323, "file path (dialog if empty)"=w1312) -> ()  [unwired: 5 in, 1 out]
                  }
                  frame "ITI" {
                    w1326 = 0 ("element")
                    n1436 = local read "lick # 1.2R"() -> (w1333:dbl)
                    n1437 = local read "water # 1.1L"() -> (w1331:dbl)
                    n1438 = local read "water # 1.2R"() -> (w1330:dbl)
                    n1439 = local read "lick # 1.1L"() -> (w1334:dbl)
                    n1440 = local read "mistake # 1.2R"() -> (w1324:dbl)
                    n1441 = local read "current sound"() -> (w1328:dbl)
                    n1442 = local read "mistake # 1.1L"() -> (w1325:dbl)
                    n1443 = local read "time (s)"() -> (w1335:dbl)
                    n1444 = local read "trial #"() -> (w1329:dbl)
                    n1445 = local read "ITI (s)"() -> (w1327:dbl)
                    n1446 = Increment(x=w1333) -> (x+1=w1332:dbl)
                    n1447 = local write "lick # 1.2R"(w1332) -> ()
                    n1448 = local read "Mouse path 1"() -> (w1338:path)
                    n1449 = Build Array(w1335, w1334, w1332, w1331, w1330, w1326, w1326, w1329, w1328, w1327, w1326, w1325, w1324) -> (w1336:dbl[])
                    n1450 = call-poly <vilib>:"Write To Spreadsheet File.vi"("append to file? (new file:F)"=TRUE, "1D data"=w1336, "file path (dialog if empty)"=w1338) -> ()  [unwired: 5 in, 1 out]
                  }
                  frame "sound" {
                    w1347 = 0 ("element")
                    n1451 = local read "1.2"() -> (w1343:bool)
                    n1452 = case shown="True" w1343 {
                      frame False {
                      }
                      frame True {
                        n1453 = local read "LED 1"() -> (w1360:tag)
                        n1454 = call "_digital_on.vi"("digital port"=w1360) -> ()  [unwired: 11 in]
                      }
                    }
                    n1455 = local read "water # 1.2R"() -> (w1351:dbl)
                    n1456 = local read "water # 1.1L"() -> (w1352:dbl)
                    n1457 = local read "lick # 1.2R"() -> (w1354:dbl)
                    n1458 = local read "lick # 1.1L"() -> (w1355:dbl)
                    n1459 = Increment(x=w1354) -> (x+1=w1353:dbl)
                    n1460 = local read "mistake # 1.2R"() -> (w1345:dbl)
                    n1461 = local read "mistake # 1.1L"() -> (w1346:dbl)
                    n1462 = local read "current sound"() -> (w1349:dbl)
                    n1463 = local read "time (s)"() -> (w1356:dbl)
                    n1464 = local write "lick # 1.2R"(w1353) -> ()
                    n1465 = local read "ITI (s)"() -> (w1348:dbl)
                    n1466 = local read "trial #"() -> (w1350:dbl)
                    n1467 = local read "Mouse path 1"() -> (w1359:path)
                    n1468 = local read "fault 1"() -> (w1341:dbl)
                    n1469 = Build Array(w1356, w1355, w1353, w1352, w1351, w1347, w1347, w1350, w1349, w1348, w1347, w1346, w1345) -> (w1357:dbl[])
                    n1470 = call-poly <vilib>:"Write To Spreadsheet File.vi"("append to file? (new file:F)"=TRUE, "1D data"=w1357, "file path (dialog if empty)"=w1359) -> ()  [unwired: 5 in, 1 out]
                    n1471 = Increment(x=w1341) -> (x+1=w1342:dbl)
                    n1472 = local write "state 1.2"(enum16{"waiting", "sound", "ITI"}."ITI") -> ()
                    n1473 = local write "state 1.1"(enum16{"waiting", "sound", "ITI"}."ITI") -> ()
                    n1474 = local write "LED 1(i)"(1.0 ("LED 1(i)")) -> ()
                    n1475 = local write "fault 1"(w1342) -> ()
                  }
                }
              }
            }
            n1476 = case shown="True" w1301 {
              frame False {
              }
              frame True {
                n1477 = local read "Mouse path 1"() -> (w1361:path)
                n1478 = local read "state 1.1"() -> (w1362:enum16{"waiting", "sound", "ITI"})
                n1479 = case shown="\"sound\"" w1362 {
                  tunnel: w1361 -> [w1369 _ w1409]
                  frame "waiting", Default {
                    w1374 = 0
                    n1480 = local read "time (s)"() -> (w1381:dbl)
                    n1481 = local read "lick # 1.1L"() -> (w1380:dbl)
                    n1482 = local read "water # 1.1L"() -> (w1379:dbl)
                    n1483 = local write "state 1.2"(enum16{"waiting", "sound", "ITI"}."ITI") -> ()
                    n1484 = local write "state 1.1"(enum16{"waiting", "sound", "ITI"}."ITI") -> ()
                    n1485 = local write "last water 1.1L"(w1381) -> ()
                    n1486 = Increment(x=w1379) -> (x+1=w1377:dbl)
                    n1487 = Increment(x=w1380) -> (x+1=w1378:dbl)
                    n1488 = local write "lick # 1.1L"(w1378) -> ()
                    n1489 = local write "water # 1.1L"(w1377) -> ()
                    n1490 = local read "lick # 1.2R"() -> (w1368:dbl)
                    n1491 = local read "free water 1.1"() -> (w1365:bool)
                    n1492 = local read "current sound"() -> (w1372:dbl)
                    n1493 = local read "trial #"() -> (w1373:dbl)
                    n1494 = local read "water # 1.2R"() -> (w1376:dbl)
                    n1495 = case shown="False" w1365 {
                      frame False {
                        n1496 = call "_digital_on_duration_off.vi"("duration (ms)"="water dur (ms) 1.1", "digital port"="water port 1.1") -> ()  [unwired: 10 in]
                      }
                      frame True {
                      }
                    }
                    n1497 = local read "ITI (s)"() -> (w1371:dbl)
                    n1498 = local read "mistake # 1.1L"() -> (w1367:dbl)
                    n1499 = local read "mistake # 1.2R"() -> (w1366:dbl)
                    n1500 = Build Array(w1381, w1378, w1368, w1377, w1376, 1, w1374, w1373, w1372, w1371, w1374, w1367, w1366) -> (w1370:dbl[])
                    n1501 = call-poly <vilib>:"Write To Spreadsheet File.vi"("append to file? (new file:F)"=TRUE, "1D data"=w1370, "file path (dialog if empty)"=w1369) -> ()  [unwired: 5 in, 1 out]
                  }
                  frame "sound" {
                    w1393 = 0 ("element")
                    n1502 = local read "1.1"() -> (w1389:bool)
                    n1503 = local read "fault 1"() -> (w1385:dbl)
                    n1504 = local write "state 1.2"(enum16{"waiting", "sound", "ITI"}."ITI") -> ()
                    n1505 = case shown="True" w1389 {
                      frame False {
                      }
                      frame True {
                        n1506 = local read "LED 1"() -> (w1406:tag)
                        n1507 = call "_digital_on.vi"("digital port"=w1406) -> ()  [unwired: 11 in]
                      }
                    }
                    n1508 = local write "state 1.1"(enum16{"waiting", "sound", "ITI"}."ITI") -> ()
                    n1509 = Increment(x=w1385) -> (x+1=w1386:dbl)
                    n1510 = local write "LED 1(i)"(1.0 ("LED 1(i)")) -> ()
                    n1511 = local write "fault 1"(w1386) -> ()
                    n1512 = local read "mistake # 1.2R"() -> (w1391:dbl)
                    n1513 = local read "water # 1.2R"() -> (w1397:dbl)
                    n1514 = local read "water # 1.1L"() -> (w1398:dbl)
                    n1515 = local read "mistake # 1.1L"() -> (w1392:dbl)
                    n1516 = local read "current sound"() -> (w1395:dbl)
                    n1517 = local read "trial #"() -> (w1396:dbl)
                    n1518 = local read "lick # 1.2R"() -> (w1399:dbl)
                    n1519 = local read "lick # 1.1L"() -> (w1401:dbl)
                    n1520 = local read "ITI (s)"() -> (w1394:dbl)
                    n1521 = Increment(x=w1401) -> (x+1=w1400:dbl)
                    n1522 = local read "time (s)"() -> (w1402:dbl)
                    n1523 = local write "lick # 1.1L"(w1400) -> ()
                    n1524 = local read "Mouse path 1"() -> (w1404:path)
                    n1525 = Build Array(w1402, w1400, w1399, w1398, w1397, w1393, w1393, w1396, w1395, w1394, w1393, w1392, w1391) -> (w1403:dbl[])
                    n1526 = call-poly <vilib>:"Write To Spreadsheet File.vi"("append to file? (new file:F)"=TRUE, "1D data"=w1403, "file path (dialog if empty)"=w1404) -> ()  [unwired: 5 in, 1 out]
                  }
                  frame "ITI" {
                    w1415 = 0
                    n1527 = local read "time (s)"() -> (w1420:dbl)
                    n1528 = local read "lick # 1.1L"() -> (w1419:dbl)
                    n1529 = local read "lick # 1.2R"() -> (w1410:dbl)
                    n1530 = Increment(x=w1419) -> (x+1=w1418:dbl)
                    n1531 = local read "water # 1.1L"() -> (w1417:dbl)
                    n1532 = local read "water # 1.2R"() -> (w1416:dbl)
                    n1533 = local write "lick # 1.1L"(w1418) -> ()
                    n1534 = local read "current sound"() -> (w1413:dbl)
                    n1535 = local read "ITI (s)"() -> (w1412:dbl)
                    n1536 = local read "trial #"() -> (w1414:dbl)
                    n1537 = local read "mistake # 1.2R"() -> (w1407:dbl)
                    n1538 = local read "mistake # 1.1L"() -> (w1408:dbl)
                    n1539 = Build Array(w1420, w1418, w1410, w1417, w1416, w1415, w1415, w1414, w1413, w1412, w1415, w1408, w1407) -> (w1411:dbl[])
                    n1540 = call-poly <vilib>:"Write To Spreadsheet File.vi"("append to file? (new file:F)"=TRUE, "1D data"=w1411, "file path (dialog if empty)"=w1409) -> ()  [unwired: 5 in, 1 out]
                  }
                }
              }
            }
          }
          frame 2 {
            n1541 = case shown="True" w1422 {
              frame False {
              }
              frame True {
                n1542 = local read "state 1.1"() -> (w1424:enum16{"waiting", "sound", "ITI"})
                n1543 = case shown="\"sound\"" w1424 {
                  frame "waiting", Default {
                    w1433 = 0
                    n1544 = local read "LED 1"() -> (w1425:tag)
                    n1545 = local read "water # 1.1L"() -> (w1427:dbl)
                    n1546 = local read "lick # 1.2R"() -> (w1439:dbl)
                    n1547 = call "_digital_on.vi"("digital port"=w1425) -> ()  [unwired: 11 in]
                    n1548 = local read "water # 1.2R"() -> (w1440:dbl)
                    n1549 = local read "time (s)"() -> (w1436:dbl)
                    n1550 = local read "current sound"() -> (w1442:dbl)
                    n1551 = local read "lick # 1.1L"() -> (w1437:dbl)
                    n1552 = local write "state 1.2"(enum16{"waiting", "sound", "ITI"}."ITI") -> ()
                    n1553 = local write "state 1.1"(enum16{"waiting", "sound", "ITI"}."ITI") -> ()
                    n1554 = local read "mistake # 1.2R"() -> (w1430:dbl)
                    n1555 = local read "ITI (s)"() -> (w1443:dbl)
                    n1556 = Increment(x=w1437) -> (x+1=w1438:dbl)
                    n1557 = local write "lick # 1.1L"(w1438) -> ()
                    n1558 = local read "mistake # 1.1L"() -> (w1432:dbl)
                    n1559 = local read "trial #"() -> (w1441:dbl)
                    n1560 = Increment(x=w1430) -> (x+1=w1429:dbl)
                    n1561 = local read "Mouse path 1"() -> (w1445:path)
                    n1562 = local write "mistake # 1.2R"(w1429) -> ()
                    n1563 = Build Array(w1436, w1438, w1439, w1427, w1440, 0.0 ("element"), w1433, w1441, w1442, w1443, w1433, w1432, w1429) -> (w1444:dbl[])
                    n1564 = call-poly <vilib>:"Write To Spreadsheet File.vi"("append to file? (new file:F)"=TRUE, "1D data"=w1444, "file path (dialog if empty)"=w1445) -> ()  [unwired: 5 in, 1 out]
                    n1565 = local write "LED 1(i)"(1.0 ("LED 1(i)")) -> ()
                  }
                  frame "ITI" {
                    w1448 = 0 ("element")
                    n1566 = local read "lick # 1.1L"() -> (w1456:dbl)
                    n1567 = local read "water # 1.2R"() -> (w1452:dbl)
                    n1568 = local read "water # 1.1L"() -> (w1453:dbl)
                    n1569 = local read "lick # 1.2R"() -> (w1454:dbl)
                    n1570 = local read "mistake # 1.2R"() -> (w1446:dbl)
                    n1571 = local read "current sound"() -> (w1450:dbl)
                    n1572 = local read "mistake # 1.1L"() -> (w1447:dbl)
                    n1573 = local read "trial #"() -> (w1451:dbl)
                    n1574 = Increment(x=w1456) -> (x+1=w1455:dbl)
                    n1575 = local read "time (s)"() -> (w1457:dbl)
                    n1576 = local read "ITI (s)"() -> (w1449:dbl)
                    n1577 = local write "lick # 1.1L"(w1455) -> ()
                    n1578 = Build Array(w1457, w1455, w1454, w1453, w1452, w1448, w1448, w1451, w1450, w1449, w1448, w1447, w1446) -> (w1458:dbl[])
                    n1579 = local read "Mouse path 1"() -> (w1460:path)
                    n1580 = call-poly <vilib>:"Write To Spreadsheet File.vi"("append to file? (new file:F)"=TRUE, "1D data"=w1458, "file path (dialog if empty)"=w1460) -> ()  [unwired: 5 in, 1 out]
                  }
                  frame "sound" {
                    w1469 = 0 ("element")
                    n1581 = local write "state 1.2"(enum16{"waiting", "sound", "ITI"}."ITI") -> ()
                    n1582 = local read "fault 1"() -> (w1461:dbl)
                    n1583 = local write "state 1.1"(enum16{"waiting", "sound", "ITI"}."ITI") -> ()
                    n1584 = local read "water # 1.2R"() -> (w1473:dbl)
                    n1585 = local read "water # 1.1L"() -> (w1474:dbl)
                    n1586 = local read "lick # 1.2R"() -> (w1475:dbl)
                    n1587 = local read "mistake # 1.2R"() -> (w1467:dbl)
                    n1588 = Increment(x=w1461) -> (x+1=w1462:dbl)
                    n1589 = local read "mistake # 1.1L"() -> (w1468:dbl)
                    n1590 = local read "current sound"() -> (w1471:dbl)
                    n1591 = local read "lick # 1.1L"() -> (w1477:dbl)
                    n1592 = local read "trial #"() -> (w1472:dbl)
                    n1593 = local read "ITI (s)"() -> (w1470:dbl)
                    n1594 = local read "time (s)"() -> (w1478:dbl)
                    n1595 = local write "fault 1"(w1462) -> ()
                    n1596 = Increment(x=w1477) -> (x+1=w1476:dbl)
                    n1597 = local write "lick # 1.1L"(w1476) -> ()
                    n1598 = local read "Mouse path 1"() -> (w1481:path)
                    n1599 = Build Array(w1478, w1476, w1475, w1474, w1473, w1469, w1469, w1472, w1471, w1470, w1469, w1468, w1467) -> (w1479:dbl[])
                    n1600 = local read "1.1"() -> (w1465:bool)
                    n1601 = case shown="True" w1465 {
                      frame False {
                      }
                      frame True {
                        n1602 = local read "LED 1"() -> (w1482:tag)
                        n1603 = call "_digital_on.vi"("digital port"=w1482) -> ()  [unwired: 11 in]
                      }
                    }
                    n1604 = call-poly <vilib>:"Write To Spreadsheet File.vi"("append to file? (new file:F)"=TRUE, "1D data"=w1479, "file path (dialog if empty)"=w1481) -> ()  [unwired: 5 in, 1 out]
                    n1605 = local write "LED 1(i)"(1.0 ("LED 1(i)")) -> ()
                  }
                }
              }
            }
            n1606 = case shown="True" w1423 {
              frame False {
              }
              frame True {
                n1607 = local read "Mouse path 1"() -> (w1483:path)
                n1608 = local read "state 1.2"() -> (w1484:enum16{"waiting", "sound", "ITI"})
                n1609 = case shown="\"sound\"" w1484 {
                  tunnel: w1483 -> [w1492 _ w1531]
                  frame "waiting", Default {
                    w1498 = 0
                    n1610 = local read "lick # 1.1L"() -> (w1491:dbl)
                    n1611 = local read "lick # 1.2R"() -> (w1490:dbl)
                    n1612 = local read "time (s)"() -> (w1503:dbl)
                    n1613 = local read "water # 1.2R"() -> (w1501:dbl)
                    n1614 = Increment(x=w1490) -> (x+1=w1489:dbl)
                    n1615 = local write "last water 1.2R"(w1503) -> ()
                    n1616 = local write "lick # 1.2R"(w1489) -> ()
                    n1617 = Increment(x=w1501) -> (x+1=w1500:dbl)
                    n1618 = local read "free water 1.2"() -> (w1486:bool)
                    n1619 = local write "water # 1.2R"(w1500) -> ()
                    n1620 = case shown="False" w1486 {
                      frame False {
                        n1621 = call "_digital_on_duration_off.vi"("duration (ms)"="water dur (ms) 1.2", "digital port"="water port 1.2") -> ()  [unwired: 10 in]
                      }
                      frame True {
                      }
                    }
                    n1622 = local read "water # 1.1L"() -> (w1502:dbl)
                    n1623 = local read "current sound"() -> (w1496:dbl)
                    n1624 = local read "trial #"() -> (w1497:dbl)
                    n1625 = local read "mistake # 1.2R"() -> (w1487:dbl)
                    n1626 = local read "mistake # 1.1L"() -> (w1488:dbl)
                    n1627 = local read "ITI (s)"() -> (w1495:dbl)
                    n1628 = Build Array(w1503, w1491, w1489, w1502, w1500, 1, w1498, w1497, w1496, w1495, w1498, w1488, w1487) -> (w1494:dbl[])
                    n1629 = local write "state 1.1"(enum16{"waiting", "sound", "ITI"}."ITI") -> ()
                    n1630 = local write "state 1.2"(enum16{"waiting", "sound", "ITI"}."ITI") -> ()
                    n1631 = call-poly <vilib>:"Write To Spreadsheet File.vi"("append to file? (new file:F)"=TRUE, "1D data"=w1494, "file path (dialog if empty)"=w1492) -> ()  [unwired: 5 in, 1 out]
                  }
                  frame "sound" {
                    w1515 = 0 ("element")
                    n1632 = local write "state 1.2"(enum16{"waiting", "sound", "ITI"}."ITI") -> ()
                    n1633 = local write "state 1.1"(enum16{"waiting", "sound", "ITI"}."ITI") -> ()
                    n1634 = local read "water # 1.2R"() -> (w1519:dbl)
                    n1635 = local read "water # 1.1L"() -> (w1520:dbl)
                    n1636 = local read "lick # 1.1L"() -> (w1522:dbl)
                    n1637 = local read "lick # 1.2R"() -> (w1523:dbl)
                    n1638 = local read "current sound"() -> (w1517:dbl)
                    n1639 = local read "mistake # 1.1L"() -> (w1514:dbl)
                    n1640 = local read "ITI (s)"() -> (w1516:dbl)
                    n1641 = local read "mistake # 1.2R"() -> (w1513:dbl)
                    n1642 = local read "trial #"() -> (w1518:dbl)
                    n1643 = local read "time (s)"() -> (w1524:dbl)
                    n1644 = Increment(x=w1523) -> (x+1=w1521:dbl)
                    n1645 = local write "lick # 1.2R"(w1521) -> ()
                    n1646 = local read "Mouse path 1"() -> (w1527:path)
                    n1647 = Build Array(w1524, w1522, w1521, w1520, w1519, w1515, w1515, w1518, w1517, w1516, w1515, w1514, w1513) -> (w1525:dbl[])
                    n1648 = call-poly <vilib>:"Write To Spreadsheet File.vi"("append to file? (new file:F)"=TRUE, "1D data"=w1525, "file path (dialog if empty)"=w1527) -> ()  [unwired: 5 in, 1 out]
                    n1649 = local read "fault 1"() -> (w1509:dbl)
                    n1650 = local read "1.2"() -> (w1511:bool)
                    n1651 = Increment(x=w1509) -> (x+1=w1510:dbl)
                    n1652 = case shown="True" w1511 {
                      frame False {
                      }
                      frame True {
                        n1653 = local read "LED 1"() -> (w1528:tag)
                        n1654 = call "_digital_on.vi"("digital port"=w1528) -> ()  [unwired: 11 in]
                      }
                    }
                    n1655 = local write "fault 1"(w1510) -> ()
                    n1656 = local write "LED 1(i)"(1.0 ("LED 1(i)")) -> ()
                  }
                  frame "ITI" {
                    w1537 = 0
                    n1657 = local read "lick # 1.1L"() -> (w1532:dbl)
                    n1658 = local read "lick # 1.2R"() -> (w1541:dbl)
                    n1659 = local read "time (s)"() -> (w1542:dbl)
                    n1660 = Increment(x=w1541) -> (x+1=w1540:dbl)
                    n1661 = local write "lick # 1.2R"(w1540) -> ()
                    n1662 = local read "water # 1.1L"() -> (w1539:dbl)
                    n1663 = local read "current sound"() -> (w1535:dbl)
                    n1664 = local read "water # 1.2R"() -> (w1538:dbl)
                    n1665 = local read "trial #"() -> (w1536:dbl)
                    n1666 = local read "mistake # 1.1L"() -> (w1530:dbl)
                    n1667 = local read "mistake # 1.2R"() -> (w1529:dbl)
                    n1668 = local read "ITI (s)"() -> (w1534:dbl)
                    n1669 = Build Array(w1542, w1532, w1540, w1539, w1538, w1537, w1537, w1536, w1535, w1534, w1537, w1530, w1529) -> (w1533:dbl[])
                    n1670 = call-poly <vilib>:"Write To Spreadsheet File.vi"("append to file? (new file:F)"=TRUE, "1D data"=w1533, "file path (dialog if empty)"=w1531) -> ()  [unwired: 5 in, 1 out]
                  }
                }
              }
            }
          }
          frame 3 {
            n1671 = case shown="True" w1545 {
              frame False {
              }
              frame True {
                n1672 = local read "state 1.1"() -> (w1604:enum16{"waiting", "sound", "ITI"})
                n1673 = case shown="\"sound\"" w1604 {
                  frame "waiting", Default {
                    w1609 = 0 ("element")
                    n1674 = local read "water # 1.2R"() -> (w1614:dbl)
                    n1675 = local read "water # 1.1L"() -> (w1616:dbl)
                    n1676 = local read "lick # 1.2R"() -> (w1617:dbl)
                    n1677 = local read "lick # 1.1L"() -> (w1619:dbl)
                    n1678 = local read "time (s)"() -> (w1620:dbl)
                    n1679 = Increment(x=w1616) -> (x+1=w1615:dbl)
                    n1680 = Increment(x=w1619) -> (x+1=w1618:dbl)
                    n1681 = local write "state 1.1"(enum16{"waiting", "sound", "ITI"}."ITI") -> ()
                    n1682 = local write "water # 1.1L"(w1615) -> ()
                    n1683 = local read "Mouse path 1"() -> (w1622:path)
                    n1684 = local write "lick # 1.1L"(w1618) -> ()
                    n1685 = local write "last water 1.1L"(w1620) -> ()
                    n1686 = local read "current sound"() -> (w1611:dbl)
                    n1687 = local read "mistake # 1.2R"() -> (w1607:dbl)
                    n1688 = local read "mistake # 1.1L"() -> (w1608:dbl)
                    n1689 = local read "ITI (s)"() -> (w1610:dbl)
                    n1690 = local read "trial #"() -> (w1612:dbl)
                    n1691 = local read "free water 1.1"() -> (w1605:bool)
                    n1692 = local write "state 1.2"(enum16{"waiting", "sound", "ITI"}."ITI") -> ()
                    n1693 = case shown="False" w1605 {
                      frame False {
                        n1694 = local read "water port 1.1"() -> (w1625:tag)
                        n1695 = local read "water dur (ms) 1.1"() -> (w1626:dbl)
                        n1696 = call "_digital_on_duration_off.vi"("duration (ms)"=w1626, "digital port"=w1625) -> ()  [unwired: 10 in]
                      }
                      frame True {
                      }
                    }
                    n1697 = Build Array(w1620, w1618, w1617, w1615, w1614, 1 ("element"), w1609, w1612, w1611, w1610, w1609, w1608, w1607) -> (w1621:dbl[])
                    n1698 = call-poly <vilib>:"Write To Spreadsheet File.vi"("append to file? (new file:F)"=TRUE, "1D data"=w1621, "file path (dialog if empty)"=w1622) -> ()  [unwired: 5 in, 1 out]
                  }
                  frame "ITI" {
                    w1629 = 0 ("element")
                    n1699 = local read "water # 1.2R"() -> (w1633:dbl)
                    n1700 = local read "water # 1.1L"() -> (w1634:dbl)
                    n1701 = local read "lick # 1.1L"() -> (w1637:dbl)
                    n1702 = local read "lick # 1.2R"() -> (w1635:dbl)
                    n1703 = local read "current sound"() -> (w1631:dbl)
                    n1704 = local read "trial #"() -> (w1632:dbl)
                    n1705 = local read "ITI (s)"() -> (w1630:dbl)
                    n1706 = local read "time (s)"() -> (w1638:dbl)
                    n1707 = Increment(x=w1637) -> (x+1=w1636:dbl)
                    n1708 = local read "mistake # 1.1L"() -> (w1628:dbl)
                    n1709 = local read "mistake # 1.2R"() -> (w1627:dbl)
                    n1710 = local write "lick # 1.1L"(w1636) -> ()
                    n1711 = local read "Mouse path 1"() -> (w1641:path)
                    n1712 = Build Array(w1638, w1636, w1635, w1634, w1633, w1629, w1629, w1632, w1631, w1630, w1629, w1628, w1627) -> (w1639:dbl[])
                    n1713 = call-poly <vilib>:"Write To Spreadsheet File.vi"("append to file? (new file:F)"=TRUE, "1D data"=w1639, "file path (dialog if empty)"=w1641) -> ()  [unwired: 5 in, 1 out]
                  }
                  frame "sound" {
                    w1650 = 0 ("element")
                    n1714 = local read "water # 1.2R"() -> (w1654:dbl)
                    n1715 = local read "1.1"() -> (w1646:bool)
                    n1716 = local read "water # 1.1L"() -> (w1655:dbl)
                    n1717 = local read "lick # 1.2R"() -> (w1656:dbl)
                    n1718 = local read "lick # 1.1L"() -> (w1658:dbl)
                    n1719 = local read "current sound"() -> (w1652:dbl)
                    n1720 = local read "mistake # 1.2R"() -> (w1648:dbl)
                    n1721 = local read "ITI (s)"() -> (w1651:dbl)
                    n1722 = local read "trial #"() -> (w1653:dbl)
                    n1723 = local read "mistake # 1.1L"() -> (w1649:dbl)
                    n1724 = case shown="True" w1646 {
                      frame False {
                      }
                      frame True {
                        n1725 = local read "LED 1"() -> (w1663:tag)
                        n1726 = call "_digital_on.vi"("digital port"=w1663) -> ()  [unwired: 11 in]
                      }
                    }
                    n1727 = local read "time (s)"() -> (w1659:dbl)
                    n1728 = Increment(x=w1658) -> (x+1=w1657:dbl)
                    n1729 = local write "lick # 1.1L"(w1657) -> ()
                    n1730 = local read "Mouse path 1"() -> (w1662:path)
                    n1731 = Build Array(w1659, w1657, w1656, w1655, w1654, w1650, w1650, w1653, w1652, w1651, w1650, w1649, w1648) -> (w1660:dbl[])
                    n1732 = local write "LED 1(i)"(1.0 ("LED 1(i)")) -> ()
                    n1733 = call-poly <vilib>:"Write To Spreadsheet File.vi"("append to file? (new file:F)"=TRUE, "1D data"=w1660, "file path (dialog if empty)"=w1662) -> ()  [unwired: 5 in, 1 out]
                    n1734 = local read "fault 1"() -> (w1642:dbl)
                    n1735 = Increment(x=w1642) -> (x+1=w1643:dbl)
                    n1736 = local write "state 1.1"(enum16{"waiting", "sound", "ITI"}."ITI") -> ()
                    n1737 = local write "state 1.2"(enum16{"waiting", "sound", "ITI"}."ITI") -> ()
                    n1738 = local write "fault 1"(w1643) -> ()
                  }
                }
              }
            }
            n1739 = case shown="True" w1544 {
              frame False {
              }
              frame True {
                n1740 = local read "state 1.2"() -> (w1546:enum16{"waiting", "sound", "ITI"})
                n1741 = case shown="\"sound\"" w1546 {
                  frame "waiting", Default {
                    w1553 = 0 ("element")
                    n1742 = local read "water # 1.2R"() -> (w1557:dbl)
                    n1743 = local read "water # 1.1L"() -> (w1558:dbl)
                    n1744 = local read "lick # 1.2R"() -> (w1560:dbl)
                    n1745 = local read "lick # 1.1L"() -> (w1561:dbl)
                    n1746 = local read "current sound"() -> (w1555:dbl)
                    n1747 = local read "mistake # 1.1L"() -> (w1551:dbl)
                    n1748 = Increment(x=w1560) -> (x+1=w1559:dbl)
                    n1749 = local read "time (s)"() -> (w1562:dbl)
                    n1750 = local read "mistake # 1.2R"() -> (w1552:dbl)
                    n1751 = local read "trial #"() -> (w1556:dbl)
                    n1752 = local read "ITI (s)"() -> (w1554:dbl)
                    n1753 = local write "lick # 1.2R"(w1559) -> ()
                    n1754 = local write "state 1.1"(enum16{"waiting", "sound", "ITI"}."ITI") -> ()
                    n1755 = Increment(x=w1551) -> (x+1=w1550:dbl)
                    n1756 = local read "Mouse path 1"() -> (w1565:path)
                    n1757 = local write "mistake # 1.1L"(w1550) -> ()
                    n1758 = local write "LED 1(i)"(1.0 ("LED 1(i)")) -> ()
                    n1759 = Build Array(w1562, w1561, w1559, w1558, w1557, w1553, w1553, w1556, w1555, w1554, w1553, w1550, w1552) -> (w1564:dbl[])
                    n1760 = call-poly <vilib>:"Write To Spreadsheet File.vi"("append to file? (new file:F)"=TRUE, "1D data"=w1564, "file path (dialog if empty)"=w1565) -> ()  [unwired: 5 in, 1 out]
                    n1761 = local read "LED 1"() -> (w1547:tag)
                    n1762 = local write "state 1.2"(enum16{"waiting", "sound", "ITI"}."ITI") -> ()
                    n1763 = call "_digital_on.vi"("digital port"=w1547) -> ()  [unwired: 11 in]
                  }
                  frame "sound" {
                    w1575 = 0 ("element")
                    n1764 = local write "state 1.2"(enum16{"waiting", "sound", "ITI"}."ITI") -> ()
                    n1765 = local read "1.2"() -> (w1571:bool)
                    n1766 = local write "state 1.1"(enum16{"waiting", "sound", "ITI"}."ITI") -> ()
                    n1767 = local read "water # 1.2R"() -> (w1579:dbl)
                    n1768 = local read "water # 1.1L"() -> (w1580:dbl)
                    n1769 = local read "lick # 1.2R"() -> (w1582:dbl)
                    n1770 = local read "current sound"() -> (w1577:dbl)
                    n1771 = case shown="True" w1571 {
                      frame False {
                      }
                      frame True {
                        n1772 = local read "LED 1"() -> (w1588:tag)
                        n1773 = call "_digital_on.vi"("digital port"=w1588) -> ()  [unwired: 11 in]
                      }
                    }
                    n1774 = local read "mistake # 1.2R"() -> (w1573:dbl)
                    n1775 = local read "lick # 1.1L"() -> (w1583:dbl)
                    n1776 = local read "ITI (s)"() -> (w1576:dbl)
                    n1777 = local read "mistake # 1.1L"() -> (w1574:dbl)
                    n1778 = local read "trial #"() -> (w1578:dbl)
                    n1779 = Increment(x=w1582) -> (x+1=w1581:dbl)
                    n1780 = local read "time (s)"() -> (w1584:dbl)
                    n1781 = local write "lick # 1.2R"(w1581) -> ()
                    n1782 = local read "Mouse path 1"() -> (w1586:path)
                    n1783 = local read "fault 1"() -> (w1568:dbl)
                    n1784 = Build Array(w1584, w1583, w1581, w1580, w1579, w1575, w1575, w1578, w1577, w1576, w1575, w1574, w1573) -> (w1585:dbl[])
                    n1785 = local write "LED 1(i)"(1.0 ("LED 1(i)")) -> ()
                    n1786 = Increment(x=w1568) -> (x+1=w1567:dbl)
                    n1787 = call-poly <vilib>:"Write To Spreadsheet File.vi"("append to file? (new file:F)"=TRUE, "1D data"=w1585, "file path (dialog if empty)"=w1586) -> ()  [unwired: 5 in, 1 out]
                    n1788 = local write "fault 1"(w1567) -> ()
                  }
                  frame "ITI" {
                    w1591 = 0 ("element")
                    n1789 = local read "water # 1.2R"() -> (w1595:dbl)
                    n1790 = local read "water # 1.1L"() -> (w1596:dbl)
                    n1791 = local read "lick # 1.2R"() -> (w1598:dbl)
                    n1792 = local read "current sound"() -> (w1593:dbl)
                    n1793 = local read "lick # 1.1L"() -> (w1599:dbl)
                    n1794 = local read "mistake # 1.2R"() -> (w1589:dbl)
                    n1795 = local read "mistake # 1.1L"() -> (w1590:dbl)
                    n1796 = local read "trial #"() -> (w1594:dbl)
                    n1797 = local read "ITI (s)"() -> (w1592:dbl)
                    n1798 = local read "time (s)"() -> (w1600:dbl)
                    n1799 = Increment(x=w1598) -> (x+1=w1597:dbl)
                    n1800 = local write "lick # 1.2R"(w1597) -> ()
                    n1801 = local read "Mouse path 1"() -> (w1603:path)
                    n1802 = Build Array(w1600, w1599, w1597, w1596, w1595, w1591, w1591, w1594, w1593, w1592, w1591, w1590, w1589) -> (w1601:dbl[])
                    n1803 = call-poly <vilib>:"Write To Spreadsheet File.vi"("append to file? (new file:F)"=TRUE, "1D data"=w1601, "file path (dialog if empty)"=w1603) -> ()  [unwired: 5 in, 1 out]
                  }
                }
              }
            }
          }
          frame 4 {
            n1804 = case shown="True" w1665 {
              frame False {
              }
              frame True {
                n1805 = local read "state 1.1"() -> (w1726:enum16{"waiting", "sound", "ITI"})
                n1806 = case shown="\"sound\"" w1726 {
                  frame "waiting", Default {
                    w1736 = 0 ("element")
                    n1807 = local read "water # 1.1L"() -> (w1738:dbl)
                    n1808 = local read "lick # 1.2R"() -> (w1739:dbl)
                    n1809 = local read "lick # 1.1L"() -> (w1741:dbl)
                    n1810 = local read "water # 1.2R"() -> (w1737:dbl)
                    n1811 = local read "mistake # 1.2R"() -> (w1731:dbl)
                    n1812 = local read "mistake # 1.1L"() -> (w1732:dbl)
                    n1813 = local read "current sound"() -> (w1734:dbl)
                    n1814 = local read "time (s)"() -> (w1742:dbl)
                    n1815 = Increment(x=w1741) -> (x+1=w1740:dbl)
                    n1816 = local read "trial #"() -> (w1735:dbl)
                    n1817 = local read "ITI (s)"() -> (w1733:dbl)
                    n1818 = local write "state 1.2"(enum16{"waiting", "sound", "ITI"}."ITI") -> ()
                    n1819 = local write "state 1.1"(enum16{"waiting", "sound", "ITI"}."ITI") -> ()
                    n1820 = local write "lick # 1.1L"(w1740) -> ()
                    n1821 = Increment(x=w1731) -> (x+1=w1730:dbl)
                    n1822 = local write "mistake # 1.2R"(w1730) -> ()
                    n1823 = local read "Mouse path 1"() -> (w1745:path)
                    n1824 = Build Array(w1742, w1740, w1739, w1738, w1737, w1736, w1736, w1735, w1734, w1733, w1732, w1730) -> (w1743:dbl[])
                    n1825 = local read "LED 1"() -> (w1727:tag)
                    n1826 = call-poly <vilib>:"Write To Spreadsheet File.vi"("append to file? (new file:F)"=TRUE, "1D data"=w1743, "file path (dialog if empty)"=w1745) -> ()  [unwired: 5 in, 1 out]
                    n1827 = call "_digital_on.vi"("digital port"=w1727) -> ()  [unwired: 11 in]
                    n1828 = local write "LED 1(i)"(1.0 ("LED 1(i)")) -> ()
                  }
                  frame "sound" {
                    w1755 = 0 ("element")
                    n1829 = local read "fault 1"() -> (w1747:dbl)
                    n1830 = local read "water # 1.2R"() -> (w1759:dbl)
                    n1831 = local read "water # 1.1L"() -> (w1760:dbl)
                    n1832 = local read "lick # 1.2R"() -> (w1761:dbl)
                    n1833 = local read "mistake # 1.2R"() -> (w1753:dbl)
                    n1834 = local read "current sound"() -> (w1757:dbl)
                    n1835 = local read "lick # 1.1L"() -> (w1763:dbl)
                    n1836 = local read "mistake # 1.1L"() -> (w1754:dbl)
                    n1837 = Increment(x=w1747) -> (x+1=w1748:dbl)
                    n1838 = local read "trial #"() -> (w1758:dbl)
                    n1839 = local read "ITI (s)"() -> (w1756:dbl)
                    n1840 = local read "time (s)"() -> (w1764:dbl)
                    n1841 = local write "fault 1"(w1748) -> ()
                    n1842 = local read "1.1"() -> (w1751:bool)
                    n1843 = Increment(x=w1763) -> (x+1=w1762:dbl)
                    n1844 = local read "Mouse path 1"() -> (w1767:path)
                    n1845 = local write "lick # 1.1L"(w1762) -> ()
                    n1846 = case shown="True" w1751 {
                      frame False {
                      }
                      frame True {
                        n1847 = local read "LED 1"() -> (w1768:tag)
                        n1848 = call "_digital_on.vi"("digital port"=w1768) -> ()  [unwired: 11 in]
                      }
                    }
                    n1849 = Build Array(w1764, w1762, w1761, w1760, w1759, w1755, w1755, w1758, w1757, w1756, w1755, w1754, w1753) -> (w1765:dbl[])
                    n1850 = call-poly <vilib>:"Write To Spreadsheet File.vi"("append to file? (new file:F)"=TRUE, "1D data"=w1765, "file path (dialog if empty)"=w1767) -> ()  [unwired: 5 in, 1 out]
                    n1851 = local write "state 1.2"(enum16{"waiting", "sound", "ITI"}."ITI") -> ()
                    n1852 = local write "state 1.1"(enum16{"waiting", "sound", "ITI"}."ITI") -> ()
                    n1853 = local write "LED 1(i)"(1.0 ("LED 1(i)")) -> ()
                  }
                  frame "ITI" {
                    w1771 = 0 ("element")
                    n1854 = local read "water # 1.2R"() -> (w1775:dbl)
                    n1855 = local read "lick # 1.1L"() -> (w1779:dbl)
                    n1856 = local read "water # 1.1L"() -> (w1776:dbl)
                    n1857 = local read "lick # 1.2R"() -> (w1777:dbl)
                    n1858 = local read "mistake # 1.2R"() -> (w1769:dbl)
                    n1859 = local read "current sound"() -> (w1773:dbl)
                    n1860 = local read "mistake # 1.1L"() -> (w1770:dbl)
                    n1861 = Increment(x=w1779) -> (x+1=w1778:dbl)
                    n1862 = local read "trial #"() -> (w1774:dbl)
                    n1863 = local read "ITI (s)"() -> (w1772:dbl)
                    n1864 = local read "time (s)"() -> (w1780:dbl)
                    n1865 = local write "lick # 1.1L"(w1778) -> ()
                    n1866 = local read "Mouse path 1"() -> (w1783:path)
                    n1867 = Build Array(w1780, w1778, w1777, w1776, w1775, w1771, w1771, w1774, w1773, w1772, w1771, w1770, w1769) -> (w1781:dbl[])
                    n1868 = call-poly <vilib>:"Write To Spreadsheet File.vi"("append to file? (new file:F)"=TRUE, "1D data"=w1781, "file path (dialog if empty)"=w1783) -> ()  [unwired: 5 in, 1 out]
                  }
                }
              }
            }
            n1869 = case shown="True" w1664 {
              frame False {
              }
              frame True {
                n1870 = local read "state 1.2"() -> (w1666:enum16{"waiting", "sound", "ITI"})
                n1871 = case shown="\"sound\"" w1666 {
                  frame "waiting", Default {
                    w1671 = 0 ("element")
                    n1872 = local read "water # 1.2R"() -> (w1677:dbl)
                    n1873 = local read "lick # 1.2R"() -> (w1680:dbl)
                    n1874 = local read "free water 1.2"() -> (w1667:bool)
                    n1875 = local read "water # 1.1L"() -> (w1678:dbl)
                    n1876 = local read "lick # 1.1L"() -> (w1681:dbl)
                    n1877 = local read "time (s)"() -> (w1682:dbl)
                    n1878 = local write "state 1.2"(enum16{"waiting", "sound", "ITI"}."ITI") -> ()
                    n1879 = local write "state 1.1"(enum16{"waiting", "sound", "ITI"}."ITI") -> ()
                    n1880 = Increment(x=w1677) -> (x+1=w1676:dbl)
                    n1881 = Increment(x=w1680) -> (x+1=w1679:dbl)
                    n1882 = case shown="False" w1667 {
                      frame False {
                        n1883 = local read "water dur (ms) 1.2"() -> (w1688:dbl)
                        n1884 = local read "water port 1.2"() -> (w1687:tag)
                        n1885 = call "_digital_on_duration_off.vi"("duration (ms)"=w1688, "digital port"=w1687) -> ()  [unwired: 10 in]
                      }
                      frame True {
                      }
                    }
                    n1886 = local write "water # 1.2R"(w1676) -> ()
                    n1887 = local write "lick # 1.2R"(w1679) -> ()
                    n1888 = local write "last water 1.2R"(w1682) -> ()
                    n1889 = local read "mistake # 1.2R"() -> (w1669:dbl)
                    n1890 = local read "mistake # 1.1L"() -> (w1670:dbl)
                    n1891 = local read "current sound"() -> (w1673:dbl)
                    n1892 = local read "ITI (s)"() -> (w1672:dbl)
                    n1893 = local read "trial #"() -> (w1674:dbl)
                    n1894 = local read "Mouse path 1"() -> (w1685:path)
                    n1895 = Build Array(w1682, w1681, w1679, w1678, w1676, 1 ("element"), w1671, w1674, w1673, w1672, w1671, w1670, w1669) -> (w1683:dbl[])
                    n1896 = call-poly <vilib>:"Write To Spreadsheet File.vi"("append to file? (new file:F)"=TRUE, "1D data"=w1683, "file path (dialog if empty)"=w1685) -> ()  [unwired: 5 in, 1 out]
                  }
                  frame "sound" {
                    w1697 = 0 ("element")
                    n1897 = local read "1.2"() -> (w1693:bool)
                    n1898 = local write "state 1.2"(enum16{"waiting", "sound", "ITI"}."ITI") -> ()
                    n1899 = case shown="True" w1693 {
                      frame False {
                      }
                      frame True {
                        n1900 = local read "LED 1"() -> (w1710:tag)
                        n1901 = call "_digital_on.vi"("digital port"=w1710) -> ()  [unwired: 11 in]
                      }
                    }
                    n1902 = local write "state 1.1"(enum16{"waiting", "sound", "ITI"}."ITI") -> ()
                    n1903 = local read "lick # 1.2R"() -> (w1704:dbl)
                    n1904 = local read "water # 1.2R"() -> (w1701:dbl)
                    n1905 = local read "water # 1.1L"() -> (w1702:dbl)
                    n1906 = local read "lick # 1.1L"() -> (w1705:dbl)
                    n1907 = local read "mistake # 1.2R"() -> (w1695:dbl)
                    n1908 = local read "current sound"() -> (w1699:dbl)
                    n1909 = local read "fault 1"() -> (w1689:dbl)
                    n1910 = Increment(x=w1704) -> (x+1=w1703:dbl)
                    n1911 = local read "mistake # 1.1L"() -> (w1696:dbl)
                    n1912 = local read "time (s)"() -> (w1706:dbl)
                    n1913 = local read "trial #"() -> (w1700:dbl)
                    n1914 = local read "ITI (s)"() -> (w1698:dbl)
                    n1915 = local write "lick # 1.2R"(w1703) -> ()
                    n1916 = local read "Mouse path 1"() -> (w1709:path)
                    n1917 = Increment(x=w1689) -> (x+1=w1690:dbl)
                    n1918 = local write "fault 1"(w1690) -> ()
                    n1919 = Build Array(w1706, w1705, w1703, w1702, w1701, w1697, w1697, w1700, w1699, w1698, w1697, w1696, w1695) -> (w1707:dbl[])
                    n1920 = call-poly <vilib>:"Write To Spreadsheet File.vi"("append to file? (new file:F)"=TRUE, "1D data"=w1707, "file path (dialog if empty)"=w1709) -> ()  [unwired: 5 in, 1 out]
                    n1921 = local write "LED 1(i)"(1.0 ("LED 1(i)")) -> ()
                  }
                  frame "ITI" {
                    w1713 = 0 ("element")
                    n1922 = local read "water # 1.2R"() -> (w1717:dbl)
                    n1923 = local read "water # 1.1L"() -> (w1718:dbl)
                    n1924 = local read "lick # 1.2R"() -> (w1720:dbl)
                    n1925 = local read "lick # 1.1L"() -> (w1721:dbl)
                    n1926 = local read "mistake # 1.2R"() -> (w1711:dbl)
                    n1927 = local read "current sound"() -> (w1715:dbl)
                    n1928 = local read "mistake # 1.1L"() -> (w1712:dbl)
                    n1929 = Increment(x=w1720) -> (x+1=w1719:dbl)
                    n1930 = local read "ITI (s)"() -> (w1714:dbl)
                    n1931 = local read "trial #"() -> (w1716:dbl)
                    n1932 = local read "time (s)"() -> (w1722:dbl)
                    n1933 = local write "lick # 1.2R"(w1719) -> ()
                    n1934 = local read "Mouse path 1"() -> (w1725:path)
                    n1935 = Build Array(w1722, w1721, w1719, w1718, w1717, w1713, w1713, w1716, w1715, w1714, w1713, w1712, w1711) -> (w1723:dbl[])
                    n1936 = call-poly <vilib>:"Write To Spreadsheet File.vi"("append to file? (new file:F)"=TRUE, "1D data"=w1723, "file path (dialog if empty)"=w1725) -> ()  [unwired: 5 in, 1 out]
                  }
                }
              }
            }
          }
        }
        n1937 = call "_loop_time.vi"("from shift register"=w85) -> ("to shift register"=w84:dbl)  [unwired: 9 in, 1 out]
        n1938 = call "Elapsed Time"() -> ("Elapsed Time (s)"=→"time (s)":dbl)  [unwired: 12 in, 7 out]
      }
      n1939 = call <vilib>:"DAQmx Clear Task.vi"("task in"=w31) -> ()  [unwired: 14 in, 1 out]
      n1940 = while {
        shift-right: [w1787] -> _
        shift-left: T1."prepare" -> [w1786]
        stop <- FALSE stop-if-true
        n1941 = local write "trial state"(w1786) -> ()
        n1942 = case shown="\"reaction window\"" w1786 {
          tunnel: [w1788 w1817 w1861 w1876 w1882 T1."ITI" T1."prepare"] -> w1787
          frame "prepare", Default {
            n1943 = flat-sequence {
              tunnel: [T1."sound"] -> w1788
              frame #0 {
                w1792 = 500
                w1799 = 1000
                n1944 = Subtract(x="ITI max (ms)", y=w1792) -> (x-y=w1795:dbl)
                n1945 = Subtract(x="ITI min (ms)", y=w1792) -> (x-y=w1796:dbl)
                n1946 = local read "next sound"() -> (w1802:dbl[])
                n1947 = Divide(x=w1795, y=w1799) -> (x/y=w1790:dbl)
                n1948 = Divide(x=w1796, y=w1799) -> (x/y=w1789:dbl)
                n1949 = Delete From Array(array=w1802, index=0) -> (deleted portion=w1800:dbl, array with subset deleted=w1801:dbl[])  [unwired: 1 in]
                n1950 = local write "next sound"(w1801) -> ()
                n1951 = call "_random_integer.vi"("max"=w1790, "min"=w1789) -> ("output"=w1793:dbl)  [unwired: 9 in]
                n1952 = local write "current sound"(w1800) -> ()
                n1953 = Add(x=w1793, y=0.5) -> (x+y=w1794:dbl)
                n1954 = local write "ITI (s)"(w1794) -> ()
              }
              frame #1 {
                w1804 = 0
                n1955 = local read "current sound"() -> (w1808:dbl)
                n1956 = local read "time (s)"() -> (w1811:dbl)
                n1957 = local read "trial #"() -> (w1814:dbl)
                n1958 = local read "ITI (s)"() -> (w1807:dbl)
                n1959 = Increment(x=w1814) -> (x+1=w1809:dbl)
                n1960 = local read "Mouse path 1"() -> (w1813:path)
                n1961 = local write "trial #"(w1809) -> ()
                n1962 = Build Array(w1811, w1804, w1804, w1804, w1804, w1804, 1, w1809, w1808, w1807, 0, w1804, w1804) -> (w1805:dbl[])
                n1963 = call-poly <vilib>:"Write To Spreadsheet File.vi"("append to file? (new file:F)"=TRUE, "1D data"=w1805, "file path (dialog if empty)"=w1813) -> ()  [unwired: 5 in, 1 out]
              }
              frame #2 {
                w1815 = enum16{"waiting", "sound", "ITI"}."sound"
                n1964 = local write "state 1.2"(w1815) -> ()
                n1965 = local write "state 1.1"(w1815) -> ()
                n1966 = local write "state 3.2"(w1815) -> ()
                n1967 = local write "state 3.1"(w1815) -> ()
                n1968 = local write "state 4.2"(w1815) -> ()
                n1969 = local write "state 2.1"(w1815) -> ()
                n1970 = local write "state 2.2"(w1815) -> ()
                n1971 = local write "state 4.1"(w1815) -> ()
              }
              frame #3 {
              }
            }
          }
          frame "sound" {
            n1972 = flat-sequence {
              tunnel: [T1."free water"] -> w1817
              frame #0 {
                n1973 = local read "current sound"() -> (w1823:dbl)
                n1974 = case shown="3" w1823 {
                  tunnel: "sound dur (ms)" -> [w1828 w1833 w1838 w1842]
                  tunnel: "sound port 1" -> [w1825 _ w1835 _]
                  tunnel: "sound port 2" -> [_ w1830 _ w1843]
                  tunnel: "sound file 1" -> [w1824 _ _ w1839]
                  tunnel: "sound file 2" -> [_ w1829 w1834 _]
                  frame ..1 {
                    n1975 = local read "Left Speaker"() -> (w1827:dbl)
                    n1976 = Increment(x=w1827) -> (x+1=w1826:dbl)
                    n1977 = local write "Left Speaker"(w1826) -> ()
                    n1978 = call "_play_wave_file.vi"("sound length (ms)"=w1828, "sound file"=w1824, "sound port"=w1825) -> ()  [unwired: 9 in]
                  }
                  frame 2 {
                    n1979 = local read "Right Speaker"() -> (w1832:dbl)
                    n1980 = Increment(x=w1832) -> (x+1=w1831:dbl)
                    n1981 = call "_play_wave_file.vi"("sound length (ms)"=w1833, "sound file"=w1829, "sound port"=w1830) -> ()  [unwired: 9 in]
                    n1982 = local write "Right Speaker"(w1831) -> ()
                  }
                  frame 3 {
                    n1983 = local read "Left Speaker"() -> (w1837:dbl)
                    n1984 = call "_play_wave_file.vi"("sound length (ms)"=w1838, "sound file"=w1834, "sound port"=w1835) -> ()  [unwired: 9 in]
                    n1985 = Increment(x=w1837) -> (x+1=w1836:dbl)
                    n1986 = local write "Left Speaker"(w1836) -> ()
                  }
                  frame 4.. {
                    n1987 = local read "Right Speaker"() -> (w1841:dbl)
                    n1988 = Increment(x=w1841) -> (x+1=w1840:dbl)
                    n1989 = call "_play_wave_file.vi"("sound length (ms)"=w1842, "sound file"=w1839, "sound port"=w1843) -> ()  [unwired: 9 in]
                    n1990 = local write "Right Speaker"(w1840) -> ()
                  }
                }
              }
              frame #1 {
                n1991 = local read "LED 4 (i)"() -> (w1844:dbl)
                n1992 = local read "LED 3 (i)"() -> (w1845:dbl)
                n1993 = local read "LED 2 (i)"() -> (w1846:dbl)
                n1994 = local read "LED 1(i)"() -> (w1847:dbl)
                n1995 = case shown="1" w1845 {
                  frame 0, Default {
                    w1851 = enum16{"waiting", "sound", "ITI"}."waiting"
                    n1996 = local write "state 3.2"(w1851) -> ()
                    n1997 = local write "state 3.1"(w1851) -> ()
                  }
                  frame 1 {
                    n1998 = local read "LED 3"() -> (w1853:tag)
                    n1999 = local write "LED 3 (i)"(0.0 ("LED 3 (i)")) -> ()
                    n2000 = call "_digital_off.vi"("digital port"=w1853) -> ()  [unwired: 11 in]
                  }
                }
                n2001 = case shown="1" w1844 {
                  frame 0, Default {
                    w1848 = enum16{"waiting", "sound", "ITI"}."waiting"
                    n2002 = local write "state 4.1"(w1848) -> ()
                    n2003 = local write "state 4.2"(w1848) -> ()
                  }
                  frame 1 {
                    n2004 = local read "LED 4"() -> (w1849:tag)
                    n2005 = local write "LED 4 (i)"(0.0 ("LED 4 (i)")) -> ()
                    n2006 = call "_digital_off.vi"("digital port"=w1849) -> ()  [unwired: 11 in]
                  }
                }
                n2007 = case shown="1" w1846 {
                  frame 0, Default {
                    w1854 = enum16{"waiting", "sound", "ITI"}."waiting"
                    n2008 = local write "state 2.1"(w1854) -> ()
                    n2009 = local write "state 2.2"(w1854) -> ()
                  }
                  frame 1 {
                    n2010 = local read "LED 2"() -> (w1856:tag)
                    n2011 = local write "LED 2 (i)"(0.0 ("LED 2 (i)")) -> ()
                    n2012 = call "_digital_off.vi"("digital port"=w1856) -> ()  [unwired: 11 in]
                  }
                }
                n2013 = case shown="1" w1847 {
                  frame 0, Default {
                    w1857 = enum16{"waiting", "sound", "ITI"}."waiting"
                    n2014 = local write "state 1.1"(w1857) -> ()
                    n2015 = local write "state 1.2"(w1857) -> ()
                  }
                  frame 1 {
                    n2016 = local read "LED 1"() -> (w1858:tag)
                    n2017 = local write "LED 1(i)"(0.0 ("LED 1(i)")) -> ()
                    n2018 = call "_digital_off.vi"("digital port"=w1858) -> ()  [unwired: 11 in]
                  }
                }
              }
              frame #2 {
              }
            }
          }
          frame "reaction window" {
            n2019 = flat-sequence {
              tunnel: [T1."graph"] -> w1861
              frame #0 {
                n2020 = Wait (ms)(milliseconds to wait="reaction dur (ms)") -> ()  [unwired: 1 out]
              }
              frame #1 {
                n2021 = local read "LED 2 (i)"() -> (w1865:dbl)
                n2022 = local read "LED 3 (i)"() -> (w1864:dbl)
                n2023 = local read "LED 1(i)"() -> (w1866:dbl)
                n2024 = local read "LED 4 (i)"() -> (w1863:dbl)
                n2025 = case shown="1" w1866 {
                  frame 0, Default {
                  }
                  frame 1 {
                    n2026 = local write "LED 1(i)"(0.0 ("LED 1(i)")) -> ()
                    n2027 = call "_digital_on_LED.vi"("digital port"="LED 1") -> ()  [unwired: 11 in]
                  }
                }
                n2028 = case shown="1" w1865 {
                  frame 0, Default {
                  }
                  frame 1 {
                    n2029 = local read "LED 2"() -> (w1872:tag)
                    n2030 = local write "LED 2 (i)"(0.0 ("LED 2 (i)")) -> ()
                    n2031 = call "_digital_on_LED.vi"("digital port"=w1872) -> ()  [unwired: 11 in]
                  }
                }
                n2032 = case shown="1" w1864 {
                  frame 0, Default {
                  }
                  frame 1 {
                    n2033 = local read "LED 3"() -> (w1870:tag)
                    n2034 = local write "LED 3 (i)"(0.0 ("LED 3 (i)")) -> ()
                    n2035 = call "_digital_on_LED.vi"("digital port"=w1870) -> ()  [unwired: 11 in]
                  }
                }
                n2036 = case shown="1" w1863 {
                  frame 0, Default {
                  }
                  frame 1 {
                    n2037 = local read "LED 4"() -> (w1868:tag)
                    n2038 = local write "LED 4 (i)"(0.0 ("LED 4 (i)")) -> ()
                    n2039 = call "_digital_on_LED.vi"("digital port"=w1868) -> ()  [unwired: 11 in]
                  }
                }
              }
              frame #2 {
              }
            }
          }
          frame "ITI" {
            n2040 = flat-sequence {
              tunnel: [T1."prepare"] -> w1876
              frame #0 {
                w1877 = enum16{"waiting", "sound", "ITI"}."ITI"
                n2041 = local write "state 1.1"(w1877) -> ()
                n2042 = local write "state 4.1"(w1877) -> ()
                n2043 = local write "state 1.2"(w1877) -> ()
                n2044 = local write "state 4.2"(w1877) -> ()
                n2045 = local write "state 2.2"(w1877) -> ()
                n2046 = local write "state 3.1"(w1877) -> ()
                n2047 = local write "state 2.1"(w1877) -> ()
                n2048 = local write "state 3.2"(w1877) -> ()
              }
              frame #1 {
                n2049 = local read "ITI (s)"() -> (w1880:dbl)
                n2050 = Multiply(x=w1880, y=1000) -> (x*y=w1878:dbl)
                n2051 = Wait (ms)(milliseconds to wait=w1878) -> ()  [unwired: 1 out]
              }
              frame #2 {
              }
            }
          }
          frame "free water" {
            n2052 = flat-sequence {
              tunnel: [T1."reaction window"] -> w1882
              frame #0 {
                n2053 = local read "state 4.2"() -> (w1886:enum16{"waiting", "sound", "ITI"})
                n2054 = local read "state 4.1"() -> (w1887:enum16{"waiting", "sound", "ITI"})
                n2055 = local read "state 1.1"() -> (w1911:enum16{"waiting", "sound", "ITI"})
                n2056 = local read "state 1.2"() -> (w1910:enum16{"waiting", "sound", "ITI"})
                n2057 = local read "state 2.1"() -> (w1898:enum16{"waiting", "sound", "ITI"})
                n2058 = local read "state 2.2"() -> (w1897:enum16{"waiting", "sound", "ITI"})
                n2059 = local read "state 3.1"() -> (w1894:enum16{"waiting", "sound", "ITI"})
                n2060 = local read "state 3.2"() -> (w1893:enum16{"waiting", "sound", "ITI"})
                n2061 = Build Array(w1911, w1910, w1898, w1897, w1894, w1893, w1887, w1886) -> (w1909:enum16{"waiting", "sound", "ITI"}[])
                n2062 = local write "free water 1.1"("free water 1.1") -> ()
                n2063 = local write "free water 1.2"("free water 1.2") -> ()
                n2064 = local write "free water 2.1"("free water 2.1") -> ()
                n2065 = local write "free water 3.1"("free water 3.1") -> ()
                n2066 = local write "free water 2.2"("free water 2.2") -> ()
                n2067 = local write "free water 3.2"("free water 3.2") -> ()
                n2068 = local write "free water 4.2"("free water 4.2") -> ()
                n2069 = local write "free water 4.1"("free water 4.1") -> ()
                n2070 = Build Array("free water 1.1", "free water 1.2", "free water 2.1", "free water 2.2", "free water 3.1", "free water 3.2", "free water 4.1", "free water 4.2") -> (w1913:bool[])
                n2071 = Equal?(x=w1909, y=enum16{"waiting", "water", "ITI"}."waiting") -> (x = y?=w1914:bool[])
                n2072 = And(x=w1914, y=w1913) -> (x .and. y?=w1912:bool[])
                n2073 = Index Array(array=w1912) -> (element #1=w1907:bool, element #2=w1904:bool, element #3=w1900:bool, element #4=w1899:bool, element #5=w1891:bool, element #6=w1890:bool, element #7=w1884:bool, element #8=w1883:bool)  [unwired: 8 in]
                n2074 = local read "current sound"() -> (w1908:dbl)
                n2075 = local read "current sound"() -> (w1901:dbl)
                n2076 = local read "current sound"() -> (w1885:dbl)
                n2077 = local read "current sound"() -> (w1892:dbl)
                n2078 = case shown="1" w1908 {
                  tunnel: w1907 -> [_ w1952 _ w1976 _]
                  tunnel: w1904 -> [_ _ w1964 _ w1979]
                  frame 0, Default {
                  }
                  frame 1 {
                    n2079 = case shown="True" w1952 {
                      frame False {
                      }
                      frame True {
                        w1953 = 0
                        n2080 = local read "water port 1.1"() -> (w1955:tag)
                        n2081 = local read "water dur (ms) 1.1"() -> (w1954:dbl)
                        n2082 = local read "current sound"() -> (w1959:dbl)
                        n2083 = local read "trial #"() -> (w1960:dbl)
                        n2084 = local read "ITI (s)"() -> (w1958:dbl)
                        n2085 = local read "time (s)"() -> (w1961:dbl)
                        n2086 = call "_digital_on_duration_off.vi"("duration (ms)"=w1954, "digital port"=w1955) -> ()  [unwired: 10 in]
                        n2087 = local read "Mouse path 1"() -> (w1962:path)
                        n2088 = Build Array(w1961, w1953, w1953, w1953, w1953, w1953, w1953, w1960, w1959, w1958, 1, w1953, w1953) -> (w1956:dbl[])
                        n2089 = call-poly <vilib>:"Write To Spreadsheet File.vi"("append to file? (new file:F)"=TRUE, "1D data"=w1956, "file path (dialog if empty)"=w1962) -> ()  [unwired: 5 in, 1 out]
                      }
                    }
                  }
                  frame 2 {
                    n2090 = case shown="True" w1964 {
                      frame False {
                      }
                      frame True {
                        w1967 = 0 ("element")
                        n2091 = local read "water dur (ms) 1.2"() -> (w1965:dbl)
                        n2092 = local read "current sound"() -> (w1970:dbl)
                        n2093 = local read "water port 1.2"() -> (w1966:tag)
                        n2094 = local read "trial #"() -> (w1971:dbl)
                        n2095 = local read "ITI (s)"() -> (w1969:dbl)
                        n2096 = local read "time (s)"() -> (w1972:dbl)
                        n2097 = call "_digital_on_duration_off.vi"("duration (ms)"=w1965, "digital port"=w1966) -> ()  [unwired: 10 in]
                        n2098 = local read "Mouse path 1"() -> (w1974:path)
                        n2099 = Build Array(w1972, w1967, w1967, w1967, w1967, w1967, w1967, w1971, w1970, w1969, 1 ("element"), w1967, w1967) -> (w1973:dbl[])
                        n2100 = call-poly <vilib>:"Write To Spreadsheet File.vi"("append to file? (new file:F)"=TRUE, "1D data"=w1973, "file path (dialog if empty)"=w1974) -> ()  [unwired: 5 in, 1 out]
                      }
                    }
                  }
                  frame 3 {
                    n2101 = case shown="True" w1976 {
                      frame False {
                      }
                      frame True {
                        n2102 = local read "water dur (ms) 1.1"() -> (w1977:dbl)
                        n2103 = local read "water port 1.1"() -> (w1978:tag)
                        n2104 = call "_digital_on_duration_off.vi"("duration (ms)"=w1977, "digital port"=w1978) -> ()  [unwired: 10 in]
                      }
                    }
                  }
                  frame 4 {
                    n2105 = case shown="True" w1979 {
                      frame False {
                      }
                      frame True {
                        n2106 = local read "water dur (ms) 1.2"() -> (w1980:dbl)
                        n2107 = local read "water port 1.2"() -> (w1981:tag)
                        n2108 = call "_digital_on_duration_off.vi"("duration (ms)"=w1980, "digital port"=w1981) -> ()  [unwired: 10 in]
                      }
                    }
                  }
                }
                n2109 = case shown="1" w1892 {
                  tunnel: w1891 -> [_ w1928 _ w1934 _]
                  tunnel: w1890 -> [_ _ w1931 _ w1937]
                  frame 0, Default {
                  }
                  frame 1 {
                    n2110 = case shown="True" w1928 {
                      frame False {
                      }
                      frame True {
                        n2111 = local read "water dur (ms) 3.1"() -> (w1929:dbl)
                        n2112 = local read "water port 3.1"() -> (w1930:tag)
                        n2113 = call "_digital_on_duration_off.vi"("duration (ms)"=w1929, "digital port"=w1930) -> ()  [unwired: 10 in]
                      }
                    }
                  }
                  frame 2 {
                    n2114 = case shown="True" w1931 {
                      frame False {
                      }
                      frame True {
                        n2115 = local read "water dur (ms) 3. 2"() -> (w1932:dbl)
                        n2116 = local read "water port 3.2"() -> (w1933:tag)
                        n2117 = call "_digital_on_duration_off.vi"("duration (ms)"=w1932, "digital port"=w1933) -> ()  [unwired: 10 in]
                      }
                    }
                  }
                  frame 3 {
                    n2118 = case shown="True" w1934 {
                      frame False {
                      }
                      frame True {
                        n2119 = local read "water dur (ms) 3.1"() -> (w1935:dbl)
                        n2120 = local read "water port 3.1"() -> (w1936:tag)
                        n2121 = call "_digital_on_duration_off.vi"("duration (ms)"=w1935, "digital port"=w1936) -> ()  [unwired: 10 in]
                      }
                    }
                  }
                  frame 4 {
                    n2122 = case shown="True" w1937 {
                      frame False {
                      }
                      frame True {
                        n2123 = local read "water dur (ms) 3. 2"() -> (w1938:dbl)
                        n2124 = local read "water port 3.2"() -> (w1939:tag)
                        n2125 = call "_digital_on_duration_off.vi"("duration (ms)"=w1938, "digital port"=w1939) -> ()  [unwired: 10 in]
                      }
                    }
                  }
                }
                n2126 = case shown="1" w1901 {
                  tunnel: w1900 -> [_ w1940 _ w1946 _]
                  tunnel: w1899 -> [_ _ w1943 _ w1949]
                  frame 0, Default {
                  }
                  frame 1 {
                    n2127 = case shown="True" w1940 {
                      frame False {
                      }
                      frame True {
                        n2128 = local read "water dur (ms) 2.1"() -> (w1941:dbl)
                        n2129 = local read "water port 2.1"() -> (w1942:tag)
                        n2130 = call "_digital_on_duration_off.vi"("duration (ms)"=w1941, "digital port"=w1942) -> ()  [unwired: 10 in]
                      }
                    }
                  }
                  frame 2 {
                    n2131 = case shown="True" w1943 {
                      frame False {
                      }
                      frame True {
                        n2132 = local read "water dur (ms) 2.2"() -> (w1944:dbl)
                        n2133 = local read "water port 2.2"() -> (w1945:tag)
                        n2134 = call "_digital_on_duration_off.vi"("duration (ms)"=w1944, "digital port"=w1945) -> ()  [unwired: 10 in]
                      }
                    }
                  }
                  frame 3 {
                    n2135 = case shown="True" w1946 {
                      frame False {
                      }
                      frame True {
                        n2136 = local read "water dur (ms) 2.1"() -> (w1947:dbl)
                        n2137 = local read "water port 2.1"() -> (w1948:tag)
                        n2138 = call "_digital_on_duration_off.vi"("duration (ms)"=w1947, "digital port"=w1948) -> ()  [unwired: 10 in]
                      }
                    }
                  }
                  frame 4 {
                    n2139 = case shown="True" w1949 {
                      frame False {
                      }
                      frame True {
                        n2140 = local read "water dur (ms) 2.2"() -> (w1950:dbl)
                        n2141 = local read "water port 2.2"() -> (w1951:tag)
                        n2142 = call "_digital_on_duration_off.vi"("duration (ms)"=w1950, "digital port"=w1951) -> ()  [unwired: 10 in]
                      }
                    }
                  }
                }
                n2143 = case shown="4" w1885 {
                  tunnel: w1884 -> [_ w1916 _ w1922 _]
                  tunnel: w1883 -> [_ _ w1919 _ w1925]
                  frame 0, Default {
                  }
                  frame 1 {
                    n2144 = case shown="True" w1916 {
                      frame False {
                      }
                      frame True {
                        n2145 = local read "water dur (ms) 4.1"() -> (w1917:dbl)
                        n2146 = local read "water port 4.1"() -> (w1918:tag)
                        n2147 = call "_digital_on_duration_off.vi"("duration (ms)"=w1917, "digital port"=w1918) -> ()  [unwired: 10 in]
                      }
                    }
                  }
                  frame 2 {
                    n2148 = case shown="True" w1919 {
                      frame False {
                      }
                      frame True {
                        n2149 = local read "water dur (ms) 4.2"() -> (w1920:dbl)
                        n2150 = local read "water port 4.2"() -> (w1921:tag)
                        n2151 = call "_digital_on_duration_off.vi"("duration (ms)"=w1920, "digital port"=w1921) -> ()  [unwired: 10 in]
                      }
                    }
                  }
                  frame 3 {
                    n2152 = case shown="True" w1922 {
                      frame False {
                      }
                      frame True {
                        n2153 = local read "water dur (ms) 4.1"() -> (w1923:dbl)
                        n2154 = local read "water port 4.1"() -> (w1924:tag)
                        n2155 = call "_digital_on_duration_off.vi"("duration (ms)"=w1923, "digital port"=w1924) -> ()  [unwired: 10 in]
                      }
                    }
                  }
                  frame 4 {
                    n2156 = case shown="True" w1925 {
                      frame False {
                      }
                      frame True {
                        n2157 = local read "water dur (ms) 4.2"() -> (w1926:dbl)
                        n2158 = local read "water port 4.2"() -> (w1927:tag)
                        n2159 = call "_digital_on_duration_off.vi"("duration (ms)"=w1926, "digital port"=w1927) -> ()  [unwired: 10 in]
                      }
                    }
                  }
                }
              }
              frame #1 {
              }
            }
          }
          frame "graph" {
            n2160 = local read "mistake # 2.2R"() -> (w2017:dbl)
            n2161 = local read "mistake # 3.1L"() -> (w2009:dbl)
            n2162 = local read "mistake # 4.2R"() -> (w1985:dbl)
            n2163 = local read "mistake # 4.1L"() -> (w1993:dbl)
            n2164 = local read "water # 4.2R"() -> (w1986:dbl)
            n2165 = local read "water # 2.2R"() -> (w2018:dbl)
            n2166 = local read "water # 4.2R"() -> (w1987:dbl)
            n2167 = local read "mistake # 2.1L"() -> (w2025:dbl)
            n2168 = local read "water # 3.1L"() -> (w2010:dbl)
            n2169 = local read "water # 2.2R"() -> (w2019:dbl)
            n2170 = local read "water # 4.1L"() -> (w1994:dbl)
            n2171 = local read "water # 2.1L"() -> (w2026:dbl)
            n2172 = local read "water # 3.1L"() -> (w2012:dbl)
            n2173 = local read "mistake # 3.2R"() -> (w2001:dbl)
            n2174 = local read "mistake # 1.2R"() -> (w2034:dbl)
            n2175 = local read "water # 3.2R"() -> (w2002:dbl)
            n2176 = local read "water # 2.1L"() -> (w2027:dbl)
            n2177 = local read "water # 4.1L"() -> (w1996:dbl)
            n2178 = local read "mistake # 1.1L"() -> (w2041:dbl)
            n2179 = local read "water # 3.2R"() -> (w2004:dbl)
            n2180 = local read "water # 1.1L"() -> (w2042:dbl)
            n2181 = local read "water # 1.2R"() -> (w2035:dbl)
            n2182 = local read "water # 1.2R"() -> (w2036:dbl)
            n2183 = local read "water # 1.1L"() -> (w2044:dbl)
            n2184 = Add(x=w1986, y=w1985) -> (x+y=w1984:dbl)
            n2185 = Add(x=w2018, y=w2017) -> (x+y=w2016:dbl)
            n2186 = Add(x=w2026, y=w2025) -> (x+y=w2024:dbl)
            n2187 = Add(x=w2010, y=w2009) -> (x+y=w2008:dbl)
            n2188 = Add(x=w2042, y=w2041) -> (x+y=w2040:dbl)
            n2189 = Add(x=w2002, y=w2001) -> (x+y=w2000:dbl)
            n2190 = Add(x=w2035, y=w2034) -> (x+y=w2033:dbl)
            n2191 = Add(x=w1994, y=w1993) -> (x+y=w1992:dbl)
            n2192 = Divide(x=w2027, y=w2024) -> (x/y=w2028:dbl)
            n2193 = Divide(x=w2004, y=w2000) -> (x/y=w2003:dbl)
            n2194 = Divide(x=w2012, y=w2008) -> (x/y=w2011:dbl)
            n2195 = Divide(x=w2019, y=w2016) -> (x/y=w2020:dbl)
            n2196 = Divide(x=w2036, y=w2033) -> (x/y=w2032:dbl)
            n2197 = Divide(x=w2044, y=w2040) -> (x/y=w2043:dbl)
            n2198 = Divide(x=w1987, y=w1984) -> (x/y=w1988:dbl)
            n2199 = Divide(x=w1996, y=w1992) -> (x/y=w1995:dbl)
            n2200 = local read "time (s)"() -> (w2048:dbl)
            n2201 = call <vilib>:"Mean PtByPt.vi"("x"=w2011) -> ("mean"=w2013:dbl)  [unwired: 3 in, 1 out]
            n2202 = call <vilib>:"Mean PtByPt.vi"("x"=w2003) -> ("mean"=w2005:dbl)  [unwired: 3 in, 1 out]
            n2203 = call <vilib>:"Mean PtByPt.vi"("x"=w2032) -> ("mean"=w2037:dbl)  [unwired: 3 in, 1 out]
            n2204 = call <vilib>:"Mean PtByPt.vi"("x"=w1995) -> ("mean"=w1997:dbl)  [unwired: 3 in, 1 out]
            n2205 = call <vilib>:"Mean PtByPt.vi"("x"=w1988) -> ("mean"=w1983:dbl)  [unwired: 3 in, 1 out]
            n2206 = call <vilib>:"Mean PtByPt.vi"("x"=w2028) -> ("mean"=w2029:dbl)  [unwired: 3 in, 1 out]
            n2207 = call <vilib>:"Mean PtByPt.vi"("x"=w2020) -> ("mean"=w2021:dbl)  [unwired: 3 in, 1 out]
            n2208 = call <vilib>:"Mean PtByPt.vi"("x"=w2043) -> ("mean"=w2045:dbl)  [unwired: 3 in, 1 out]
            n2209 = local write "ratio 1.2R"(w2037) -> ()
            n2210 = local write "ratio 1.1L"(w2045) -> ()
            n2211 = local write "ratio 2.1L"(w2029) -> ()
            n2212 = local write "ratio 3.1L"(w2013) -> ()
            n2213 = local write "ratio 2.2R"(w2021) -> ()
            n2214 = local write "ratio 3.2R"(w2005) -> ()
            n2215 = call "ratio"("Signals"=w2048) -> ("Collected Signals"=w1989:dynamicdata)  [unwired: 9 in, 1 out]
            n2216 = call "ratio1"("Signals"=w2045) -> ("Collected Signals"=w2047:dynamicdata)  [unwired: 9 in, 1 out]
            n2217 = local write "ratio 4.2R"(w1983) -> ()
            n2218 = call "ratio2"("Signals"=w2037) -> ("Collected Signals"=w2039:dynamicdata)  [unwired: 9 in, 1 out]
            n2219 = local write "ratio 4.1L"(w1997) -> ()
            n2220 = call "ratio3"("Signals"=w2029) -> ("Collected Signals"=w2031:dynamicdata)  [unwired: 9 in, 1 out]
            n2221 = call "ratio5"("Signals"=w2013) -> ("Collected Signals"=w2015:dynamicdata)  [unwired: 9 in, 1 out]
            n2222 = call "ratio4"("Signals"=w2021) -> ("Collected Signals"=w2023:dynamicdata)  [unwired: 9 in, 1 out]
            n2223 = call "ratio6"("Signals"=w2005) -> ("Collected Signals"=w2007:dynamicdata)  [unwired: 9 in, 1 out]
            n2224 = call "ratio7"("Signals"=w1997) -> ("Collected Signals"=w1999:dynamicdata)  [unwired: 9 in, 1 out]
            n2225 = call "ratio8"("Signals"=w1983) -> ("Collected Signals"=w1991:dynamicdata)  [unwired: 9 in, 1 out]
            n2226 = call "Build ratio1"("Y Input"=w2047, "X Input"=w1989) -> ("XY Graph"=→"ratio 1.1L":cluster{"Y":dbl[], "Y":dbl[]}[])  [unwired: 3 in, 6 out]
            n2227 = call "Build ratio"("Y Input"=w2039, "X Input"=w1989) -> ("XY Graph"=→"ratio 1.2R":cluster{"Y":dbl[], "Y":dbl[]}[])  [unwired: 3 in, 6 out]
            n2228 = call "Build ratio2"("Y Input"=w2031, "X Input"=w1989) -> ("XY Graph"=→"ratio 2.1L":cluster{"Y":dbl[], "Y":dbl[]}[])  [unwired: 3 in, 6 out]
            n2229 = call "Build ratio4"("Y Input"=w2015, "X Input"=w1989) -> ("XY Graph"=→"ratio 3.1L":cluster{"Y":dbl[], "Y":dbl[]}[])  [unwired: 3 in, 6 out]
            n2230 = call "Build ratio3"("Y Input"=w2023, "X Input"=w1989) -> ("XY Graph"=→"ratio 2.2R":cluster{"Y":dbl[], "Y":dbl[]}[])  [unwired: 3 in, 6 out]
            n2231 = call "Build ratio5"("Y Input"=w2007, "X Input"=w1989) -> ("XY Graph"=→"ratio 3.2R":cluster{"Y":dbl[], "Y":dbl[]}[])  [unwired: 3 in, 6 out]
            n2232 = call "Build ratio6"("Y Input"=w1999, "X Input"=w1989) -> ("XY Graph"=→"ratio 4.1L":cluster{"Y":dbl[], "Y":dbl[]}[])  [unwired: 3 in, 6 out]
            n2233 = call "Build ratio7"("Y Input"=w1991, "X Input"=w1989) -> ("XY Graph"=→"ratio 4.2R":cluster{"Y":dbl[], "Y":dbl[]}[])  [unwired: 3 in, 6 out]
          }
          frame "data collection" {
          }
        }
        n2234 = Wait (ms)(milliseconds to wait=u32 0) -> ()  [unwired: 1 out]
      }
    }
  }
